vi "DetectorTest_MainV9.vi"() -> ()   [LabVIEW 2012]
uses:
  LabVIEW/Detector IV/SMU Settings.ctl
  <vilib>/Utility/file.llb/Write To Spreadsheet File (string).vi
  <vilib>/Utility/file.llb/Read From Spreadsheet File (string).vi
  <vilib>/Utility/file.llb/Read From Spreadsheet File (DBL).vi
  <vilib>/Analysis/NI_AALBase.lvlib
panel:
  out "RecipeID":string
  in  "Sweep Direction (Keysight)":i32(ring) items=["Up", "Down"]
  in  "Auto Adjust Compliance?":bool
  out "Auto Temp Counter":i32
  out "iteration":i32
  in  "Temp Data":T1={"Ambient Temperature"=20.38176242851337, "Chuck Set Temperature"=35.0} {"Chuck Set Temperature" format="%#.1g"; "Ambient Temperature" format="%#.1g"}
  in  "Wafer Info 3":T2={"Cell Name (Automatic)"="Open_Diode_1000", "Package"="", "Coating"="FOR_AIR", "Comment"="IV test for lot 371", "Flash Setup"="5500_99_03p5", "Hrs under test"=0.0}
  out "TempCounter":i32
  out "WaferCounter":i32
  in  "Profile Z":bool
  in  "Load Wafer":bool
  out "Raw Test Skipped":bool=TRUE
  out "device name w skip":string="Open_Diode_1000(skip)"
  in  "4-wire":bool
  out "Laser Counter":i32
  out "Output Power (mW)":dbl=5.674
  out "Counter":i32
  out "NameList":string[](array[string])
  in  "Wafer Info Flash 2":T3={"Cell Name"="5500_130_05", "Package"="", "Coating"="", "LRC?"=enum."J2", "Comment"="", "Hours Under Test"=0.0}
  in  "Parameters Flash 2":T4 {"Voc" format="%#_4g"; "Isc" format="%#_4g"; "FF" format="%#_4g"; "Imax" format="%#_4g"; "Vmax" format="%#_4g"; "Pmax" format="%#_4g"; "Itest" format="%#_4g"}
  in  "Wafer Info Flash":T3={"Cell Name"="Open_Diode_1000", "Package"="", "Coating"="", "LRC?"=enum."J2", "Comment"="", "Hours Under Test"=0.0}
  in  "Parameters Flash":T4={"Voc"=0.0, "Isc"=0.0, "FF"=0.0, "Vtest"=0.0, "Imax"=0.0, "Vmax"=0.0, "Pmax"=0.0, "Itest"=0.0, "Efficiency"=0.0, "Incident Power"=5.674, "Power Density (W/cm^2)"=0.6679328011361159, "Cell Area (cm²)"=849486.6535, "Number of AM1.5D Suns"=0.0, "Input Current (mA)"=40.0, "Equivalent 1 sun Jsc"=0.0} {"Voc" format="%#_4g"; "Isc" format="%#_4g"; "FF" format="%#_4g"; "Imax" format="%#_4g"; "Vmax" format="%#_4g"; "Pmax" format="%#_4g"; "Itest" format="%#_4g"}
  out "RawData file":path=path "C:/Users/Flash/Desktop/Data/Detector test data/SJC_ENG_371_4-GaAs/A-3719-2-A/Raw Data/A-3719-2-A_Open_Diode_1000_20180913075240.csv"
  out "Fine Cell Clusters":T5(array[cluster])=[{"Cell Name"="Open_Diode_1000", "X-coord"=46800.0, "Y-coord"=22950.0, "Area"=849486.6535, "Grid Shadowing"=0.0, "Xdim"=500.0, "Ydim"=500.0, "Mesa Area"=785398.1634}]
  out "Selected Data":cluster{dbl[], dbl[]}={[nan, nan, nan, nan, nan, nan, nan, nan, nan, nan, nan, nan, nan, nan, nan, nan, nan, nan, nan, nan, nan, nan, nan, nan, nan, nan, nan, nan, nan, nan, nan, nan, nan, nan, nan, nan, nan, nan, nan, nan, nan, nan, nan, nan, nan, nan, nan, nan, nan, nan, nan, nan, nan, nan, nan, nan, nan, nan, nan, nan, nan, nan, nan, nan, nan, nan, nan, nan, nan, nan, nan, nan, nan, nan, nan, nan, nan, nan, nan, nan, nan, nan, nan, nan], [nan, nan, nan, nan, nan, nan, nan, nan, nan, nan, nan, nan, nan, nan, nan, nan, nan, nan, nan, nan, nan, nan, nan, nan, nan, nan, nan, nan, nan, nan, nan, nan, nan, nan, nan, nan, nan, nan, nan, nan, nan, nan, nan, nan, nan, nan, nan, nan, nan, nan, nan, nan, nan, nan, nan, nan, nan, nan, nan, nan, nan, nan, nan, nan, nan, nan, nan, nan, nan, nan, nan, nan, nan, nan, nan, nan, nan, nan, nan, nan, nan, nan, nan, nan]}
  in  "Test Results 2":T6
  in  "Session Info 2":T7={"V set"=-1.0, "I compliance"=0.001, "J set"=0.01, "I set"=0.0, "V compliance"=1.0, "Laser Power (mW)"=0.0, "TestID"=0, "Session Time"=timestamp(0 s since 1904-01-01), "Operator"="Radek"} {"V compliance" format="%#_6f"; "I compliance" format="%#_6e"}
  in  "Die Info 2":T8={"Device Name"="", "ActiveArea_um2"=3848.451, "MesaArea_um2"=3848.451, "x"=0.0, "y"=0.0}
  in  "Wafer Info 2":T9
  in  "Test Results":T6={"I meas"=-1.83245e-12, "V meas"=6.01176, "Time"=timestamp(3619695820.3512325 s since 1904-01-01)}
  in  "Session Info":T7={"V set"=-6.0, "I compliance"=0.001, "J set"=0.01, "I set"=1.9634954079999997e-05, "V compliance"=6.0, "Laser Power (mW)"=0.0, "TestID"=1794, "Session Time"=timestamp(3619695160.866512 s since 1904-01-01), "Operator"="sswifter"} {"V compliance" format="%#_6f"; "I compliance" format="%#_6e"}
  in  "Die Info":T8={"Device Name"="Open_Diode_1000", "ActiveArea_um2"=849486.6535, "MesaArea_um2"=785398.1634, "x"=26800.0, "y"=72950.0}
  in  "Wafer Info":T9={"Wafer Name"="A-3719-2-A", "Scribe"="BJ325-089", "Mask"="PH001", "Lot"="SJC_ENG_371_4-GaAs"}
  in  "Name Array":string[](array[string])=["Wafer name", "Scribe", "Mask", "Lot", "Device name", "Active Area", "Mesa Area", "x", "y", "Imeas", "Vmeas", "Time", "Vset", "Icomp", "Jset", "Iset", "Vcomp", "Laser Power", "TestID", "SessionTime", "Operator", "Selected"]
  in  "TestID file":path=path "C:/Users/Flash/Desktop/LabVIEW/Detector IV/rawtest_log.csv"
  in  "update wafer":bool
  in  "Lot":string="SJC_ENG_370_4-GaAs"
  in  "Laser Current (mA)":dbl
  in  "Device Name":string="Open_Diode_100"
  in  "Scribe":string="BO534-034"
  in  "MesaArea_um2":dbl=15393.804
  out "Status":string="idle"
  out "error out":errorcluster
  in  "error in (no error)":errorcluster
  out "Manaul Plot 1":cluster{"V manual":dbl[], dbl[]}[](array[cluster])=[{"V manual"=[-1.0, -0.964103, -0.928205, -0.892308, -0.85641, -0.820513, -0.784615, -0.748718, -0.712821, -0.676923, -0.641026, -0.605128, -0.569231, -0.533333, -0.497436, -0.461538, -0.425641, -0.389744, -0.353846, -0.317949, -0.282051, -0.246154, -0.210256, -0.174359, -0.138462, -0.102564, -0.0666667, -0.0307693, 0.00512815, 0.0410256, 0.076923, 0.11282, 0.148718, 0.184615, 0.220513, 0.25641, 0.292308, 0.328205, 0.364102, 0.4], [6.85852e-09, 6.65466e-09, 6.5737e-09, 6.49824e-09, 6.4243e-09, 6.35309e-09, 6.27965e-09, 6.20877e-09, 6.13492e-09, 6.06098e-09, 5.98696e-09, 5.91398e-09, 5.83835e-09, 5.76118e-09, 5.68377e-09, 5.60285e-09, 5.52235e-09, 5.437e-09, 5.34957e-09, 5.26073e-09, 5.1657e-09, 5.06509e-09, 4.95213e-09, 4.8214e-09, 4.64754e-09, 4.36963e-09, 3.83525e-09, 2.58988e-09, 1.53713e-10, 2.90069e-08, 4.00867e-08, 2.32852e-07, 3.64301e-07, 1.01107e-06, 2.70206e-06, 6.95726e-06, 1.74528e-05, 3.97407e-05, 8.44992e-05, 0.000100038]}, {"V manual"=[-6.0, nan, nan, nan, nan, nan, nan, nan, nan, nan, nan, nan, nan, nan, nan, nan, nan, nan, nan, nan, nan, nan, nan, nan, nan, nan, nan, nan, nan, nan, nan, nan, nan, nan, nan, nan, nan, nan, nan, nan], [1.709842e-08, nan, nan, nan, nan, nan, nan, nan, nan, nan, nan, nan, nan, nan, nan, nan, nan, nan, nan, nan, nan, nan, nan, nan, nan, nan, nan, nan, nan, nan, nan, nan, nan, nan, nan, nan, nan, nan, nan, nan]}, {"V manual"=[0.126049, nan, nan, nan, nan, nan, nan, nan, nan, nan, nan, nan, nan, nan, nan, nan, nan, nan, nan, nan, nan, nan, nan, nan, nan, nan, nan, nan, nan, nan, nan, nan, nan, nan, nan, nan, nan, nan, nan, nan], [1.9634954080000002e-07, nan, nan, nan, nan, nan, nan, nan, nan, nan, nan, nan, nan, nan, nan, nan, nan, nan, nan, nan, nan, nan, nan, nan, nan, nan, nan, nan, nan, nan, nan, nan, nan, nan, nan, nan, nan, nan, nan, nan]}]
  out "Manual Plot 0":cluster{"V manual":dbl[], "I manual":dbl[]}[](array[cluster])=[{"V manual"=[-1.0, -0.964103, -0.928205, -0.892308, -0.85641, -0.820513, -0.784615, -0.748718, -0.712821, -0.676923, -0.641026, -0.605128, -0.569231, -0.533333, -0.497436, -0.461538, -0.425641, -0.389744, -0.353846, -0.317949, -0.282051, -0.246154, -0.210256, -0.174359, -0.138462, -0.102564, -0.0666667, -0.0307693, 0.00512815, 0.0410256, 0.076923, 0.11282, 0.148718, 0.184615, 0.220513, 0.25641, 0.292308, 0.328205, 0.364102, 0.4], "I manual"=[-6.85852e-09, -6.65466e-09, -6.5737e-09, -6.49824e-09, -6.4243e-09, -6.35309e-09, -6.27965e-09, -6.20877e-09, -6.13492e-09, -6.06098e-09, -5.98696e-09, -5.91398e-09, -5.83835e-09, -5.76118e-09, -5.68377e-09, -5.60285e-09, -5.52235e-09, -5.437e-09, -5.34957e-09, -5.26073e-09, -5.1657e-09, -5.06509e-09, -4.95213e-09, -4.8214e-09, -4.64754e-09, -4.36963e-09, -3.83525e-09, -2.58988e-09, 1.53713e-10, 2.90069e-08, 4.00867e-08, 2.32852e-07, 3.64301e-07, 1.01107e-06, 2.70206e-06, 6.95726e-06, 1.74528e-05, 3.97407e-05, 8.44992e-05, 0.000100038]}, {"V manual"=[-6.0, nan, nan, nan, nan, nan, nan, nan, nan, nan, nan, nan, nan, nan, nan, nan, nan, nan, nan, nan, nan, nan, nan, nan, nan, nan, nan, nan, nan, nan, nan, nan, nan, nan, nan, nan, nan, nan, nan, nan], "I manual"=[-1.709842e-08, nan, nan, nan, nan, nan, nan, nan, nan, nan, nan, nan, nan, nan, nan, nan, nan, nan, nan, nan, nan, nan, nan, nan, nan, nan, nan, nan, nan, nan, nan, nan, nan, nan, nan, nan, nan, nan, nan, nan]}, {"V manual"=[0.126049, nan, nan, nan, nan, nan, nan, nan, nan, nan, nan, nan, nan, nan, nan, nan, nan, nan, nan, nan, nan, nan, nan, nan, nan, nan, nan, nan, nan, nan, nan, nan, nan, nan, nan, nan, nan, nan, nan, nan], "I manual"=[1.9634954080000002e-07, nan, nan, nan, nan, nan, nan, nan, nan, nan, nan, nan, nan, nan, nan, nan, nan, nan, nan, nan, nan, nan, nan, nan, nan, nan, nan, nan, nan, nan, nan, nan, nan, nan, nan, nan, nan, nan, nan, nan]}]
  in  "Reset 1st die":bool
  in  "Sweep Settings":T10={"Channel"=enum."Channel A", "Vstart"=-2.0, "Vend"=0.5, "# of points"=30, "NPLC"=1.0, "I compliance"=0.001, "Delay ms"=500.0}
  in  "Reset xy":bool
  out "current y":i32=1870
  out "current x":i32=23900
  in  "sweep delay ms":dbl=500.0
  in  "I compliance sweep":dbl=0.0001
  in  "points":u16=40
  in  "V end":dbl=0.4
  in  "V start":dbl=-1.0
  in  "Repeat Vf":u32=1
  out "I set":dbl=1.5393804e-06
  in  "V compliance":dbl=6.0 format="%#_6f"
  in  "Vf delay ms":dbl=100.0
  in  "J set A/cm2":dbl=0.01
  in  "Repeat Id":u32=5
  in  "I compliance":dbl=0.001 format="%#_6e"
  in  "Id delay ms":dbl=500.0
  in  "V set":dbl=-6.0
  out "Vmeas Settings":T11={"Channel"=enum."Channel A", "Vset"=1.9634954080000002e-07, "NPLC"=1.0, "I compliance"=6.0, "Repeat time"=1, "Delay ms"=100.0, "4-wire"=FALSE}
  out "Imeas Settings":T11={"Channel"=enum."Channel A", "Vset"=-6.0, "NPLC"=1.0, "I compliance"=0.001, "Repeat time"=5, "Delay ms"=500.0, "4-wire"=FALSE}
  out "Array of Cell Data Clusters":T12(array[cluster])=[{"Cell Name"="Open_Diode_100", "X-coord"=19500.0, "Y-coord"=-4780.0, "Area"=7853.981634, "Grid Shadowing"=0.0, "Ydim"=70.0, "Xdim"=70.0, "Meas Area"=15393.804}, {"Cell Name"="Open_Diode_100", "X-coord"=29500.0, "Y-coord"=-4780.0, "Area"=7853.981634, "Grid Shadowing"=0.0, "Ydim"=70.0, "Xdim"=70.0, "Meas Area"=15393.804}, {"Cell Name"="Open_Diode_100", "X-coord"=3900.0, "Y-coord"=1870.0, "Area"=7853.981634, "Grid Shadowing"=0.0, "Ydim"=70.0, "Xdim"=70.0, "Meas Area"=15393.804}, {"Cell Name"="Open_Diode_100", "X-coord"=13900.0, "Y-coord"=1870.0, "Area"=7853.981634, "Grid Shadowing"=0.0, "Ydim"=70.0, "Xdim"=70.0, "Meas Area"=15393.804}, {"Cell Name"="Open_Diode_100", "X-coord"=23900.0, "Y-coord"=1870.0, "Area"=7853.981634, "Grid Shadowing"=0.0, "Ydim"=70.0, "Xdim"=70.0, "Meas Area"=15393.804}, {"Cell Name"="Open_Diode_100", "X-coord"=9500.0, "Y-coord"=5220.0, "Area"=7853.981634, "Grid Shadowing"=0.0, "Ydim"=70.0, "Xdim"=70.0, "Meas Area"=15393.804}, {"Cell Name"="Open_Diode_100", "X-coord"=19500.0, "Y-coord"=15220.0, "Area"=7853.981634, "Grid Shadowing"=0.0, "Ydim"=70.0, "Xdim"=70.0, "Meas Area"=15393.804}, {"Cell Name"="Open_Diode_100", "X-coord"=39500.0, "Y-coord"=15220.0, "Area"=7853.981634, "Grid Shadowing"=0.0, "Ydim"=70.0, "Xdim"=70.0, "Meas Area"=15393.804}, {"Cell Name"="Open_Diode_100", "X-coord"=-16100.0, "Y-coord"=31870.0, "Area"=7853.981634, "Grid Shadowing"=0.0, "Ydim"=70.0, "Xdim"=70.0, "Meas Area"=15393.804}, {"Cell Name"="Open_Diode_100", "X-coord"=-10500.0, "Y-coord"=55220.0, "Area"=7853.981634, "Grid Shadowing"=0.0, "Ydim"=70.0, "Xdim"=70.0, "Meas Area"=15393.804}]
  in  "stop":bool
  in  "ActiveArea_um2":dbl=7853.981634
  in  "NPLC":dbl=1.0
  in  "Operator":string(combo)="sswifter"
  in  "Mask":string="PH001"
  in  "Wafer Name":string="A-3680-2-A"
  in  "Tab Control":T13(tab)=enum."Manual Test"
  in  "First Wafer Loaded?":bool
  in  "begin lot test":bool
  in  "Desired Wafer Name":string
  in  "Wafer List":i32(listbox)=-1
  in  "Add to wafer list":bool
  in  "Remove from wafer list":bool
  in  "Clear wafer list":bool
  in  "Generate Report":bool
  in  "Only Raw Test":bool
  in  "Clear Laser List":bool
  in  "Remove from Laser List":bool
  in  "Add to Laser":bool
  in  "Desired Current (mA)":dbl=40.0
  in  "Laser List":i32(listbox)=-1
  in  "Start auto":bool
  in  "Clear List":bool
  in  "Refresh Device":bool
  in  "Mask Name":string
  in  "Remove from List":bool
  in  "Add to list":bool
  in  "Available Device Name":string(combo)="Open_Diode_1000"
  in  "Test List":i32(listbox)=-1
  in  "Mask File all":path=path "C:/Users/Flash/Desktop/Mask Files/PH001 Detector GSG/PH001_Detector Aligner mask map file _ full top_open top 10_open top 5 diodes.csv"
  in  "Skip Raw Test?":bool
  in  "Test description":string="IV test for lot 371"
  in  "Clear temp list Auto":bool
  in  "Remove from Temp Auto":bool
  in  "Add to Temp Auto":bool
  in  "Auto Temp Set":dbl=25.0
  in  "Auto Temperature List":i32(listbox)=-1
  in  "Manual_Test":bool
  in  "Manual IV settting":enum32{"Linear plot", "Log plot"}(radio)
  out "Vmeas manual":dbl=0.126049
  out "Imeas manual":dbl=-1.709842e-08
  out "Iarray manual":dbl[](array[numeric])=[-6.85852e-09, -6.65466e-09, -6.5737e-09, -6.49824e-09, -6.4243e-09, -6.35309e-09, -6.27965e-09, -6.20877e-09, -6.13492e-09, -6.06098e-09, -5.98696e-09, -5.91398e-09, -5.83835e-09, -5.76118e-09, -5.68377e-09, -5.60285e-09, -5.52235e-09, -5.437e-09, -5.34957e-09, -5.26073e-09, -5.1657e-09, -5.06509e-09, -4.95213e-09, -4.8214e-09, -4.64754e-09, -4.36963e-09, -3.83525e-09, -2.58988e-09, 1.53713e-10, 2.90069e-08, 4.00867e-08, 2.32852e-07, 3.64301e-07, 1.01107e-06, 2.70206e-06, 6.95726e-06, 1.74528e-05, 3.97407e-05, 8.44992e-05, 0.000100038]
  out "Varray manual":dbl[](array[numeric])=[-1.0, -0.964103, -0.928205, -0.892308, -0.85641, -0.820513, -0.784615, -0.748718, -0.712821, -0.676923, -0.641026, -0.605128, -0.569231, -0.533333, -0.497436, -0.461538, -0.425641, -0.389744, -0.353846, -0.317949, -0.282051, -0.246154, -0.210256, -0.174359, -0.138462, -0.102564, -0.0666667, -0.0307693, 0.00512815, 0.0410256, 0.076923, 0.11282, 0.148718, 0.184615, 0.220513, 0.25641, 0.292308, 0.328205, 0.364102, 0.4]
  out "y target":i32=1870
  out "x target":i32=23900
  in  "Die Number":u16(ring)=4 items=["0", "1", "2", "3", "4", "5", "6", "7", "8", "9", "10", "11", "12", "13", "14", "15", "16", "17", "18", "19", "20", "21", "22", "23", "24", "25", "26", "27", "28", "29", "30", "31", "32", "33", "34", "35", "36", "37", "38", "39", "40", "41", "42", "43", "44", "45", "46", "47", "48", "49", "50", "51", "52", "53", "54", "55", "56", "57", "58", "59", "60", "61", "62", "63", "64", "65", "66", "67", "68", "69", "70", "71", "72", "73", "74", "75", "76", "77", "78", "79", "80", "81", "82", "83", "84", "85"]
  in  "load file":bool
  in  "Move to":bool
  in  "Mask File Manual":path=path "C:/Users/Flash/Desktop/Data/Detector test data/SJC_ENG_370_4-GaAs/A-3680-2-A/Raw Data/PH001_Detector Aligner mask map file _ full top_open top 10_open top 5 diodes_Open_Diode_100_A-3680-2-A_080118_021510.3PM.csv"
  out "Manual IV":cluster{"V manual":dbl[], "I manual":dbl[]}[](graph)=[{"V manual"=[-1.0, -0.964103, -0.928205, -0.892308, -0.85641, -0.820513, -0.784615, -0.748718, -0.712821, -0.676923, -0.641026, -0.605128, -0.569231, -0.533333, -0.497436, -0.461538, -0.425641, -0.389744, -0.353846, -0.317949, -0.282051, -0.246154, -0.210256, -0.174359, -0.138462, -0.102564, -0.0666667, -0.0307693, 0.00512815, 0.0410256, 0.076923, 0.11282, 0.148718, 0.184615, 0.220513, 0.25641, 0.292308, 0.328205, 0.364102, 0.4], "I manual"=[-6.85852e-09, -6.65466e-09, -6.5737e-09, -6.49824e-09, -6.4243e-09, -6.35309e-09, -6.27965e-09, -6.20877e-09, -6.13492e-09, -6.06098e-09, -5.98696e-09, -5.91398e-09, -5.83835e-09, -5.76118e-09, -5.68377e-09, -5.60285e-09, -5.52235e-09, -5.437e-09, -5.34957e-09, -5.26073e-09, -5.1657e-09, -5.06509e-09, -4.95213e-09, -4.8214e-09, -4.64754e-09, -4.36963e-09, -3.83525e-09, -2.58988e-09, 1.53713e-10, 2.90069e-08, 4.00867e-08, 2.32852e-07, 3.64301e-07, 1.01107e-06, 2.70206e-06, 6.95726e-06, 1.74528e-05, 3.97407e-05, 8.44992e-05, 0.000100038]}, {"V manual"=[-6.0, nan, nan, nan, nan, nan, nan, nan, nan, nan, nan, nan, nan, nan, nan, nan, nan, nan, nan, nan, nan, nan, nan, nan, nan, nan, nan, nan, nan, nan, nan, nan, nan, nan, nan, nan, nan, nan, nan, nan], "I manual"=[-1.709842e-08, nan, nan, nan, nan, nan, nan, nan, nan, nan, nan, nan, nan, nan, nan, nan, nan, nan, nan, nan, nan, nan, nan, nan, nan, nan, nan, nan, nan, nan, nan, nan, nan, nan, nan, nan, nan, nan, nan, nan]}, {"V manual"=[0.126049, nan, nan, nan, nan, nan, nan, nan, nan, nan, nan, nan, nan, nan, nan, nan, nan, nan, nan, nan, nan, nan, nan, nan, nan, nan, nan, nan, nan, nan, nan, nan, nan, nan, nan, nan, nan, nan, nan, nan], "I manual"=[1.9634954080000002e-07, nan, nan, nan, nan, nan, nan, nan, nan, nan, nan, nan, nan, nan, nan, nan, nan, nan, nan, nan, nan, nan, nan, nan, nan, nan, nan, nan, nan, nan, nan, nan, nan, nan, nan, nan, nan, nan, nan, nan]}]
  in  "Measure 2 Point?":bool=TRUE
  in  "Manual Test Comments":string="IV test for lot 371"
  in  "Load raw":bool
  in  "Select":bool
  in  "Number Select":u16=10
  in  "Vmax":dbl=5.699999999999999
  in  "Vmin":dbl=0.05
  out "Test FileName":string="A-3719-2-A_Open_Diode_1000_20180913075240.csv"
  out "RawTest ID":u32=1794
  out "Progress":u8(slide)=99 scale=0.0..100.0
  out "Current Device":u32=84
  out "Total Device":u32=84
  out "V meas":dbl[](array[numeric])=[6.01142, 6.01054, 6.01089, 0.000137925, 6.01222, 6.01216, 6.01145, 6.01193, 6.0103, 6.01103, 6.01162, 6.01132, 6.01127, 6.01137, 6.01132, 6.01125, 6.01108, 6.01134, 6.01154, 6.01135, 6.01146, 6.01204, 6.01111, 6.01101, 6.01053, 6.01143, 6.01152, 6.01128, 6.00993, 6.00994, 6.01042, 3.58707, 6.01175, 6.01164, 6.01056, 6.01166, 6.01073, 6.01098, 6.01142, 6.01026, 6.01071, 6.01116, 6.01174, 6.01214, 6.01026, 6.01093, 5.99486, 6.01138, 6.01091, 6.01133, 6.01086, 6.01094, 6.01192, 6.01232, 6.01069, 6.01162, 6.01233, 6.01184, 6.0022, 5.17964, 6.01156, 6.01223, 6.01107, 6.0102, 6.0108, 6.01164, 5.75188, 5.06441, 6.01144, 6.01129, 6.01161, 6.01159, 6.01096, 5.61419, 5.16536, 6.01197, 6.01142, 6.01186, 6.01133, 6.01132, 6.01119, 6.01113, 5.83632, 6.01176]
  out "I meas":dbl[](array[numeric])=[-3.868033999999999e-11, -1.2052780000000002e-09, -6.028065999999999e-11, -0.0009999796, -3.0170019999999996e-11, -4.752688e-11, -4.8625459999999994e-11, -3.7159980000000005e-11, -1.7203160000000002e-07, -2.00883e-08, -7.974548e-11, -3.897576e-11, -3.555112e-11, -2.188194e-08, -5.2771619999999994e-11, -2.9935519999999994e-11, -3.295828e-11, -5.707007999999999e-08, -4.796104e-07, -2.002028e-08, -7.080146e-08, -4.18e-11, -2.108774e-11, -4.09959e-11, -4.424556e-11, -3.3264100000000003e-09, -2.0351338000000002e-10, -6.144901999999999e-09, -4.3002719999999993e-11, -3.898936e-09, -2.0389360000000002e-11, -2.049748e-08, -6.527374000000001e-10, -1.0336196000000001e-10, -2.697004e-11, -3.376518e-08, -6.171924e-11, -2.02069e-10, -1.200538e-09, -2.8179300000000003e-11, -6.537938e-10, -5.153115999999999e-11, -2.8508420000000003e-09, -7.534774e-07, -2.636916e-07, -1.446754e-09, -9.464432000000001e-11, -1.0602588000000001e-10, -4.217728e-11, -7.227086e-08, -3.990094e-11, -2.7389038000000002e-11, -1.90881e-07, -2.2892700000000004e-12, -4.745506e-08, -4.579318e-11, -4.5842860000000003e-11, -5.953868e-11, -3.758154e-11, -4.4363539999999995e-09, -7.143562e-11, -1.397812e-10, -7.11463e-11, -5.56664e-11, -2.6296820000000003e-08, -1.1582659999999999e-07, -2.317642e-11, -5.807276000000001e-11, -2.17813e-12, -5.7970201999999995e-11, -6.71486e-11, -8.667722000000001e-12, 3.2483739999999993e-12, -6.306573999999999e-11, -8.307524e-11, -2.4324079999999998e-12, -2.795726e-12, -2.185576e-12, -2.0225460000000002e-12, -2.122472e-12, -1.6340760000000001e-06, -2.5727129999999997e-06, -3.269066e-11, -1.83245e-12]
  in  "RawData Save Path":path=path "C:/Users/Flash/Desktop/Data/Detector test data"
  in  "StartRaw":bool
  out "Vforward hist":T14(graph)={"X Values"=[0.30074752875, 0.90196673625, 1.5031859437500001, 2.10440515125, 2.70562435875, 3.3068435662500004, 3.90806277375, 4.50928198125, 5.110501188750001, 5.7117203962500005], "Histogram: h(x)"=[1, 0, 0, 0, 0, 1, 0, 0, 3, 79]}
  out "Idark hist":T14(graph)={"X Values"=[-0.0009499806198375813, -0.0008499826595127439, -0.0007499846991879066, -0.0006499867388630691, -0.0005499887785382317, -0.0004499908182133943, -0.0003499928578885569, -0.0002499948975637195, -0.0001499969372388821, -4.99989769140447e-05], "Histogram: h(x)"=[1, 0, 0, 0, 0, 0, 0, 0, 0, 83]}
  in  "Mask File Raw":path=path "C:/Users/Flash/Desktop/Mask Files/PH001 Detector GSG/PH001_Detector Aligner mask map file _ full top_open top 10_open top 5 diodes_Open_Diode_1000.csv"
  out "Spec Plot":cluster{"V meas":dbl[], "I meas":dbl[]}[](graph)=[{"V meas"=[6.01142, 6.01054, 6.01089, 0.000137925, 6.01222, 6.01216, 6.01145, 6.01193, 6.0103, 6.01103, 6.01162, 6.01132, 6.01127, 6.01137, 6.01132, 6.01125, 6.01108, 6.01134, 6.01154, 6.01135, 6.01146, 6.01204, 6.01111, 6.01101, 6.01053, 6.01143, 6.01152, 6.01128, 6.00993, 6.00994, 6.01042, 3.58707, 6.01175, 6.01164, 6.01056, 6.01166, 6.01073, 6.01098, 6.01142, 6.01026, 6.01071, 6.01116, 6.01174, 6.01214, 6.01026, 6.01093, 5.99486, 6.01138, 6.01091, 6.01133, 6.01086, 6.01094, 6.01192, 6.01232, 6.01069, 6.01162, 6.01233, 6.01184, 6.0022, 5.17964, 6.01156, 6.01223, 6.01107, 6.0102, 6.0108, 6.01164, 5.75188, 5.06441, 6.01144, 6.01129, 6.01161, 6.01159, 6.01096, 5.61419, 5.16536, 6.01197, 6.01142, 6.01186, 6.01133, 6.01132, 6.01119, 6.01113, 5.83632, 6.01176], "I meas"=[-3.868033999999999e-11, -1.2052780000000002e-09, -6.028065999999999e-11, -0.0009999796, -3.0170019999999996e-11, -4.752688e-11, -4.8625459999999994e-11, -3.7159980000000005e-11, -1.7203160000000002e-07, -2.00883e-08, -7.974548e-11, -3.897576e-11, -3.555112e-11, -2.188194e-08, -5.2771619999999994e-11, -2.9935519999999994e-11, -3.295828e-11, -5.707007999999999e-08, -4.796104e-07, -2.002028e-08, -7.080146e-08, -4.18e-11, -2.108774e-11, -4.09959e-11, -4.424556e-11, -3.3264100000000003e-09, -2.0351338000000002e-10, -6.144901999999999e-09, -4.3002719999999993e-11, -3.898936e-09, -2.0389360000000002e-11, -2.049748e-08, -6.527374000000001e-10, -1.0336196000000001e-10, -2.697004e-11, -3.376518e-08, -6.171924e-11, -2.02069e-10, -1.200538e-09, -2.8179300000000003e-11, -6.537938e-10, -5.153115999999999e-11, -2.8508420000000003e-09, -7.534774e-07, -2.636916e-07, -1.446754e-09, -9.464432000000001e-11, -1.0602588000000001e-10, -4.217728e-11, -7.227086e-08, -3.990094e-11, -2.7389038000000002e-11, -1.90881e-07, -2.2892700000000004e-12, -4.745506e-08, -4.579318e-11, -4.5842860000000003e-11, -5.953868e-11, -3.758154e-11, -4.4363539999999995e-09, -7.143562e-11, -1.397812e-10, -7.11463e-11, -5.56664e-11, -2.6296820000000003e-08, -1.1582659999999999e-07, -2.317642e-11, -5.807276000000001e-11, -2.17813e-12, -5.7970201999999995e-11, -6.71486e-11, -8.667722000000001e-12, 3.2483739999999993e-12, -6.306573999999999e-11, -8.307524e-11, -2.4324079999999998e-12, -2.795726e-12, -2.185576e-12, -2.0225460000000002e-12, -2.122472e-12, -1.6340760000000001e-06, -2.5727129999999997e-06, -3.269066e-11, -1.83245e-12]}, {"V meas"=[3.58707, nan, nan, nan, nan, nan, nan, nan, nan, nan, nan, nan, nan, nan, nan, nan, nan, nan, nan, nan, nan, nan, nan, nan, nan, nan, nan, nan, nan, nan, nan, nan, nan, nan, nan, nan, nan, nan, nan, nan, nan, nan, nan, nan, nan, nan, nan, nan, nan, nan, nan, nan, nan, nan, nan, nan, nan, nan, nan, nan, nan, nan, nan, nan, nan, nan, nan, nan, nan, nan, nan, nan, nan, nan, nan, nan, nan, nan, nan, nan, nan, nan, nan, nan], "I meas"=[-2.049748e-08, nan, nan, nan, nan, nan, nan, nan, nan, nan, nan, nan, nan, nan, nan, nan, nan, nan, nan, nan, nan, nan, nan, nan, nan, nan, nan, nan, nan, nan, nan, nan, nan, nan, nan, nan, nan, nan, nan, nan, nan, nan, nan, nan, nan, nan, nan, nan, nan, nan, nan, nan, nan, nan, nan, nan, nan, nan, nan, nan, nan, nan, nan, nan, nan, nan, nan, nan, nan, nan, nan, nan, nan, nan, nan, nan, nan, nan, nan, nan, nan, nan, nan, nan]}]
  in  "Explore Data":bool
  out "no file":bool
  in  "Comments":string="IV test for lot 371"
  in  "FineTest save path":path=path "C:/Users/Flash/Desktop/Data/Detector test data"
  out "I fine":dbl[](array[numeric])=[-2.70504e-08, -2.32087e-08, -1.94015e-08, -1.62001e-08, -1.3396e-08, -1.06144e-08, -8.14274e-09, -5.83125e-09, -3.66964e-09, -2.05099e-09, -1.05505e-09, -6.56038e-10, -4.43558e-10, -3.24538e-10, -2.3071e-10, -1.84326e-10, -1.50747e-10, -1.31042e-10, -1.1589e-10, -1.0217e-10, -9.29752e-11, -8.22993e-11, -7.74358e-11, -6.84813e-11, -6.19634e-11, -5.51294e-11, -4.86827e-11, -4.15262e-11, -3.40749e-11, -2.82174e-11, -2.14966e-11, -1.33787e-11, -7.37435e-12, -5.50663e-12, 4.69868e-12, 1.38179e-11, 4.52471e-11, 2.99241e-10, 1.96981e-09, 2.81104e-08]
  out "V fine":dbl[](array[numeric])=[-6.0, -5.82051, -5.64103, -5.46154, -5.28205, -5.10256, -4.92308, -4.74359, -4.5641, -4.38461, -4.20513, -4.02564, -3.84615, -3.66667, -3.48718, -3.30769, -3.1282, -2.94872, -2.76923, -2.58974, -2.41026, -2.23077, -2.05128, -1.87179, -1.69231, -1.51282, -1.33333, -1.15384, -0.974358, -0.79487, -0.615383, -0.435896, -0.256409, -0.0769218, 0.102565, 0.282053, 0.46154, 0.641027, 0.820514, 1.0]
  out "Current Device":u32=1
  out "Total Device":u32=1
  out "IV fine log":cluster{dbl[], dbl[]}[](graph)=[{[-6.0, -5.82051, -5.64103, -5.46154, -5.28205, -5.10256, -4.92308, -4.74359, -4.5641, -4.38461, -4.20513, -4.02564, -3.84615, -3.66667, -3.48718, -3.30769, -3.1282, -2.94872, -2.76923, -2.58974, -2.41026, -2.23077, -2.05128, -1.87179, -1.69231, -1.51282, -1.33333, -1.15384, -0.974358, -0.79487, -0.615383, -0.435896, -0.256409, -0.0769218, 0.102565, 0.282053, 0.46154, 0.641027, 0.820514, 1.0], [2.70504e-08, 2.32087e-08, 1.94015e-08, 1.62001e-08, 1.3396e-08, 1.06144e-08, 8.14274e-09, 5.83125e-09, 3.66964e-09, 2.05099e-09, 1.05505e-09, 6.56038e-10, 4.43558e-10, 3.24538e-10, 2.3071e-10, 1.84326e-10, 1.50747e-10, 1.31042e-10, 1.1589e-10, 1.0217e-10, 9.29752e-11, 8.22993e-11, 7.74358e-11, 6.84813e-11, 6.19634e-11, 5.51294e-11, 4.86827e-11, 4.15262e-11, 3.40749e-11, 2.82174e-11, 2.14966e-11, 1.33787e-11, 7.37435e-12, 5.50663e-12, 4.69868e-12, 1.38179e-11, 4.52471e-11, 2.99241e-10, 1.96981e-09, 2.81104e-08]}]
  out "Progress 2":u8(slide)=100 scale=0.0..100.0
  in  "StartFine":bool
  out "IV fine linear":cluster{dbl[], dbl[]}[](graph)=[{[-6.0, -5.82051, -5.64103, -5.46154, -5.28205, -5.10256, -4.92308, -4.74359, -4.5641, -4.38461, -4.20513, -4.02564, -3.84615, -3.66667, -3.48718, -3.30769, -3.1282, -2.94872, -2.76923, -2.58974, -2.41026, -2.23077, -2.05128, -1.87179, -1.69231, -1.51282, -1.33333, -1.15384, -0.974358, -0.79487, -0.615383, -0.435896, -0.256409, -0.0769218, 0.102565, 0.282053, 0.46154, 0.641027, 0.820514, 1.0], [-2.70504e-08, -2.32087e-08, -1.94015e-08, -1.62001e-08, -1.3396e-08, -1.06144e-08, -8.14274e-09, -5.83125e-09, -3.66964e-09, -2.05099e-09, -1.05505e-09, -6.56038e-10, -4.43558e-10, -3.24538e-10, -2.3071e-10, -1.84326e-10, -1.50747e-10, -1.31042e-10, -1.1589e-10, -1.0217e-10, -9.29752e-11, -8.22993e-11, -7.74358e-11, -6.84813e-11, -6.19634e-11, -5.51294e-11, -4.86827e-11, -4.15262e-11, -3.40749e-11, -2.82174e-11, -2.14966e-11, -1.33787e-11, -7.37435e-12, -5.50663e-12, 4.69868e-12, 1.38179e-11, 4.52471e-11, 2.99241e-10, 1.96981e-09, 2.81104e-08]}]
  in  "Mask File Fine":path=path "C:/Users/Flash/Desktop/Data/Detector test data/SJC_ENG_371_4-GaAs/A-3719-2-A/Raw Data/PH001_Detector Aligner mask map file _ full top_open top 10_open top 5 diodes_Open_Diode_1000_A-3719-2-A_091318_080341.5AM.csv"
  out "Y":dbl
  out "X":dbl
  in  "move prober 2":bool
  in  "load file for temp series":bool
  in  "Mask File Temperature":path=path "C:/Users/Flash/Desktop/Data/Detector test data/PH001 Detector Aligner mask map file _ full top_open top 10_open top 5 diodes_Open_Diode_5_300_A-3605-1-A_052518_113739.0AM.csv"
  out "IV temp linear":cluster{dbl[], dbl[]}[](graph)
  in  "Start temp":bool
  out "IV temp log":cluster{dbl[], dbl[]}[](graph)
  out "V fine temp":dbl[](array[numeric])=[-1.5, -1.45128, -1.40256, -1.35385, -1.30513, -1.25641, -1.20769, -1.15897, -1.11026, -1.06154, -1.01282, -0.964102, -0.915384, -0.866666, -0.817948, -0.76923, -0.720512, -0.671794, -0.623076, -0.574358, -0.52564, -0.476923, -0.428205, -0.379487, -0.330769, -0.282051, -0.233333, -0.184615, -0.135897, -0.087179, -0.038461, 0.0102569, 0.0589749, 0.107693, 0.156411, 0.205129, 0.253847, 0.302565, 0.351283, 0.400001]
  out "I fine temp":dbl[](array[numeric])=[-1.28772e-07, -1.20805e-07, -1.15592e-07, -1.10987e-07, -1.06412e-07, -1.02022e-07, -4.62038e-08, -9.34188e-08, -8.97462e-08, -8.60003e-08, -8.23237e-08, -7.87101e-08, -7.52945e-08, -7.18306e-08, -6.85145e-08, -6.5287e-08, -6.2088e-08, -5.90038e-08, -5.59938e-08, -5.29941e-08, -5.00661e-08, -4.71812e-08, -4.43421e-08, -4.15389e-08, -3.87298e-08, -3.5945e-08, -3.31511e-08, -3.027e-08, -2.71168e-08, -2.30654e-08, -1.54139e-08, 7.82768e-09, 2.30625e-07, 5.07951e-07, 2.21662e-06, 9.15235e-06, 3.37902e-05, 9.47719e-05, 0.000202989, 0.000357986]
  in  "Temperature Series save path":path=path "C:/Users/Flash/Desktop/Data/Detector test data"
  in  "Comments Temp":string
  in  "Single Device Temperature List":i32(listbox)=-1
  in  "Desired Temperature":dbl=25.0
  in  "Add to Temp":bool
  in  "Remove from Temp":bool
  in  "Clear temp list":bool
  in  "Desired Device":u16(ring)=50 items=["0", "1", "2", "3", "4", "5", "6", "7", "8", "9"]
  in  "Channel Keysight":dbl
  in  "Keysight SMU":refnum<visa-resource-name>="GPIB0::23::INSTR"
  in  "update temp":bool
  out "Current Temp":string="0\r"
  in  "Temp Setpoint":string="25"
  in  "Temptronics VISA":refnum<visa-resource-name>="GPIB0::9::INSTR"
  in  "Prober GPIB":string="0:1"
  in  "Keithley SMU":refnum<visa-resource-name>="GPIB0::26::INSTR"
  in  "Channel":enum32{"Channel A", "Channel B"}(ring)
  out "Calibration":cluster{"Y":dbl[], "Y":dbl[]}[](graph)=[{"Y"=[0.1, 0.2, 0.3, 0.4, 0.5, 0.6, 0.7, 0.8, 0.9, 1.0, 1.1, 1.2, 1.3, 1.4, 1.5, 1.6, 1.7, 1.8, 1.9, 2.0, 2.1, 2.2, 2.3, 2.4, 2.5, 2.6, 2.7, 2.8, 2.9, 3.0, 3.1, 3.2, 3.3, 3.4, 3.5, 3.6, 3.7, 3.8, 3.9, 4.0, 4.1, 4.2, 4.3, 4.4, 4.5, 4.6, 4.7, 4.8, 4.9, 5.0, 5.1, 5.2, 5.3, 5.4, 5.5, 5.6, 5.7, 5.8, 5.9, 6.0, 6.1, 6.2, 6.3, 6.4, 6.5, 6.6, 6.7, 6.8, 6.9, 7.0, 7.1, 7.2, 7.3, 7.4, 7.5, 7.6, 7.7, 7.8, 7.9, 8.0, 8.1, 8.2, 8.3, 8.4, 8.5, 8.6, 8.7, 8.8, 8.9, 9.0, 9.1, 9.2, 9.3, 9.4, 9.5, 9.6, 9.7, 9.8, 9.9, 10.0, 10.1, 10.2, 10.3, 10.4, 10.5, 10.6, 10.7, 10.8, 10.9, 11.0, 11.1, 11.2, 11.3, 11.4, 11.5, 11.6, 11.7, 11.8, 11.9, 12.0, 12.1, 12.2, 12.3, 12.4, 12.5, 12.6, 12.7, 12.8, 12.9, 13.0, 13.1, 13.2, 13.3, 13.4, 13.5, 13.6, 13.7, 13.8, 13.9, 14.0, 14.1, 14.2, 14.3, 14.4, 14.5, 14.6, 14.7, 14.8, 14.9, 15.0, 15.1, 15.2, 15.3, 15.4, 15.5, 15.6, 15.7, 15.8, 15.9, 16.0, 16.1, 16.2, 16.3, 16.4, 16.5, 16.6, 16.7, 16.8, 16.9, 17.0, 17.1, 17.2, 17.3, 17.4, 17.5, 17.6, 17.7, 17.8, 17.9, 18.0, 18.1, 18.2, 18.3, 18.4, 18.5, 18.6, 18.7, 18.8, 18.9, 19.0, 19.1, 19.2, 19.3, 19.4, 19.5, 19.6, 19.7, 19.8, 19.9, 20.0, 20.1, 20.2, 20.3, 20.4, 20.5, 20.6, 20.7, 20.8, 20.9, 21.0, 21.1, 21.2, 21.3, 21.4, 21.5, 21.6, 21.7, 21.8, 21.9, 22.0, 22.1, 22.2, 22.3, 22.4, 22.5, 22.6, 22.7, 22.8, 22.9, 23.0, 23.1, 23.2, 23.3, 23.4, 23.5, 23.6, 23.7, 23.8, 23.9, 24.0, 24.1, 24.2, 24.3, 24.4, 24.5, 24.6, 24.7, 24.8, 24.9, 25.0, 25.1, 25.2, 25.3, 25.4, 25.5, 25.6, 25.7, 25.8, 25.9, 26.0, 26.1, 26.2, 26.3, 26.4, 26.5, 26.6, 26.7, 26.8, 26.9, 27.0, 27.1, 27.2, 27.3, 27.4, 27.5, 27.6, 27.7, 27.8, 27.9, 28.0, 28.1, 28.2, 28.3, 28.4, 28.5, 28.6, 28.7, 28.8, 28.9, 29.0, 29.1, 29.2, 29.3, 29.4, 29.5, 29.6, 29.7, 29.8, 29.9, 30.0, 30.1, 30.2, 30.3, 30.4, 30.5, 30.6, 30.7, 30.8, 30.9, 31.0, 31.1, 31.2, 31.3, 31.4, 31.5, 31.6, 31.7, 31.8, 31.9, 32.0, 32.1, 32.2, 32.3, 32.4, 32.5, 32.6, 32.7, 32.8, 32.9, 33.0, 33.1, 33.2, 33.3, 33.4, 33.5, 33.6, 33.7, 33.8, 33.9, 34.0, 34.1, 34.2, 34.3, 34.4, 34.5, 34.6, 34.7, 34.8, 34.9, 35.0, 35.1, 35.2, 35.3, 35.4, 35.5, 35.6, 35.7, 35.8, 35.9, 36.0, 36.1, 36.2, 36.3, 36.4, 36.5, 36.6, 36.7, 36.8, 36.9, 37.0, 37.1, 37.2, 37.3, 37.4, 37.5, 37.6, 37.7, 37.8, 37.9, 38.0, 38.1, 38.2, 38.3, 38.4, 38.5, 38.6, 38.7, 38.8, 38.9, 39.0, 39.1, 39.2, 39.3, 39.4, 39.5, 39.6, 39.7, 39.8, 39.9, 40.0], "Y"=[0.0, 0.0, 0.0, 0.0, 0.0, 0.0, 0.0, 0.0, 0.0, 0.0, 0.0, 0.0, 0.0, 0.0, 0.0, 0.0, 0.0, 0.0, 0.001, 0.001, 0.001, 0.001, 0.001, 0.001, 0.001, 0.001, 0.001, 0.001, 0.001, 0.001, 0.001, 0.001, 0.001, 0.001, 0.001, 0.002, 0.002, 0.002, 0.002, 0.002, 0.002, 0.002, 0.002, 0.002, 0.002, 0.003, 0.003, 0.003, 0.003, 0.003, 0.003, 0.004, 0.004, 0.004, 0.004, 0.004, 0.005, 0.005, 0.005, 0.005, 0.006, 0.006, 0.006, 0.007, 0.007, 0.007, 0.008, 0.008, 0.008, 0.009, 0.009, 0.01, 0.01, 0.01, 0.011, 0.012, 0.012, 0.013, 0.013, 0.014, 0.015, 0.016, 0.018, 0.023, 0.036, 0.055, 0.071, 0.088, 0.105, 0.121, 0.143, 0.159, 0.176, 0.194, 0.209, 0.232, 0.249, 0.276, 0.28, 0.301, 0.317, 0.335, 0.354, 0.37, 0.388, 0.407, 0.423, 0.438, 0.455, 0.481, 0.493, 0.522, 0.535, 0.558, 0.57, 0.579, 0.608, 0.62, 0.648, 0.662, 0.671, 0.693, 0.703, 0.738, 0.756, 0.773, 0.782, 0.813, 0.817, 0.846, 0.841, 0.865, 0.892, 0.904, 0.933, 0.952, 0.972, 0.989, 1.01, 1.002, 1.032, 1.049, 1.067, 1.088, 1.1, 1.132, 1.144, 1.168, 1.158, 1.184, 1.223, 1.242, 1.265, 1.263, 1.305, 1.322, 1.304, 1.319, 1.346, 1.374, 1.375, 1.393, 1.448, 1.465, 1.465, 1.465, 1.523, 1.539, 1.534, 1.533, 1.59, 1.598, 1.631, 1.612, 1.62, 1.669, 1.69, 1.675, 1.743, 1.708, 1.765, 1.792, 1.818, 1.802, 1.849, 1.86, 1.885, 1.878, 1.925, 1.898, 1.933, 1.954, 2.001, 1.968, 1.999, 2.011, 2.068, 2.088, 2.093, 2.076, 2.114, 2.142, 2.124, 2.194, 2.202, 2.222, 2.246, 2.238, 2.229, 2.251, 2.265, 2.274, 2.308, 2.377, 2.382, 2.344, 2.43, 2.443, 2.404, 2.426, 2.457, 2.524, 2.511, 2.511, 2.504, 2.582, 2.604, 2.555, 2.583, 2.625, 3.197, 2.696, 2.645, 2.677, 2.73, 2.716, 2.711, 2.739, 2.796, 2.848, 2.864, 2.809, 2.898, 2.837, 2.86, 2.9, 2.964, 2.937, 2.994, 2.997, 2.966, 2.981, 2.995, 3.086, 3.108, 3.131, 3.063, 3.166, 3.164, 3.177, 3.156, 3.188, 3.248, 3.2, 3.239, 3.236, 3.307, 3.278, 3.333, 3.298, 3.403, 3.412, 3.394, 3.397, 3.469, 3.414, 3.479, 3.518, 3.464, 3.525, 3.483, 3.499, 3.554, 3.529, 3.653, 3.658, 3.64, 3.606, 3.711, 3.667, 3.648, 3.756, 3.752, 3.755, 3.742, 3.808, 3.775, 3.812, 3.83, 3.884, 3.868, 3.959, 3.966, 3.901, 3.934, 4.01, 4.032, 4.011, 4.045, 4.004, 4.096, 4.131, 4.163, 4.17, 4.084, 4.219, 4.195, 4.184, 4.2, 4.165, 4.246, 4.204, 4.233, 4.256, 4.344, 4.377, 4.299, 4.33, 4.326, 4.344, 4.485, 4.513, 4.507, 4.427, 4.473, 4.582, 4.461, 4.559, 4.63, 4.638, 4.569, 4.583, 4.569, 4.63, 4.596, 4.765, 4.758, 4.682, 4.821, 4.692, 4.757, 4.868, 4.783, 4.891, 4.808, 4.879, 4.88, 4.873, 4.99, 4.965, 5.016, 4.934, 5.058, 5.076, 5.076, 5.058, 5.066, 5.085, 5.138, 5.185, 5.185, 5.228, 5.218, 5.266, 5.176, 5.184, 5.266, 5.196, 5.333, 5.358, 5.246, 5.3, 5.314, 5.297, 5.32, 5.486, 5.353, 5.483, 5.442, 5.408, 5.557, 5.436, 5.581, 5.619, 5.616, 5.564, 5.557, 5.669, 5.7, 5.674]}]
  out "Laser Error":errorcluster caption="error out" {"code" format="%.0x"}
  in  "Load Calibration File":path=path "C:/Users/Flash/Desktop/Laser Calibration Files/Calib7_23_18.csv"
  in  "TL4000 In":refnum<visa-resource-name>="USB0::0x1313::0x804F::M00445403::INSTR" caption="resource name"
  in  "Enable Laser":bool=TRUE
  out "Raw Test Filename":path=path "C:/Users/Flash/Desktop/Data/Detector test data/SJC_ENG_371_4-GaAs/A-3719-2-A/Raw Data/A-3719-2-A_Open_Diode_1000_20180913075240.csv"
  out "new raw data save path":path=path "C:/Users/Flash/Desktop/Data/Detector test data/SJC_ENG_371_4-GaAs/A-3719-2-A/Raw Data"
  out "Error Out":errorcluster
  in  "Wait after load":u32
  in  "Keysight":bool
  out "Test Type":string="Auto Test"
  in  "Update viewer":bool
  in  "Logview":i32(listbox)
  in  "Add Comments":string
  in  "Save Comment":bool
  out "Last Measurement":T15={"result string"="9_13_2018", "time string"="11:39 AM", "Wafer Name"="A-3719-2-A", "Operator"="sswifter", "Test description"="IV test for lot 371", "Test Type"="Auto Test"}
  # "0 is for dark IV!"
  # "Sweep Settings"
  # "Forward Voltage"
  # "Dark/Light Current"
  # "Check settings before click start!"
  # "Make sure current x and y are same as prober before click Start!"
  # "TEC Control"
  # "TL4000 Settings"
  # "Keithley"
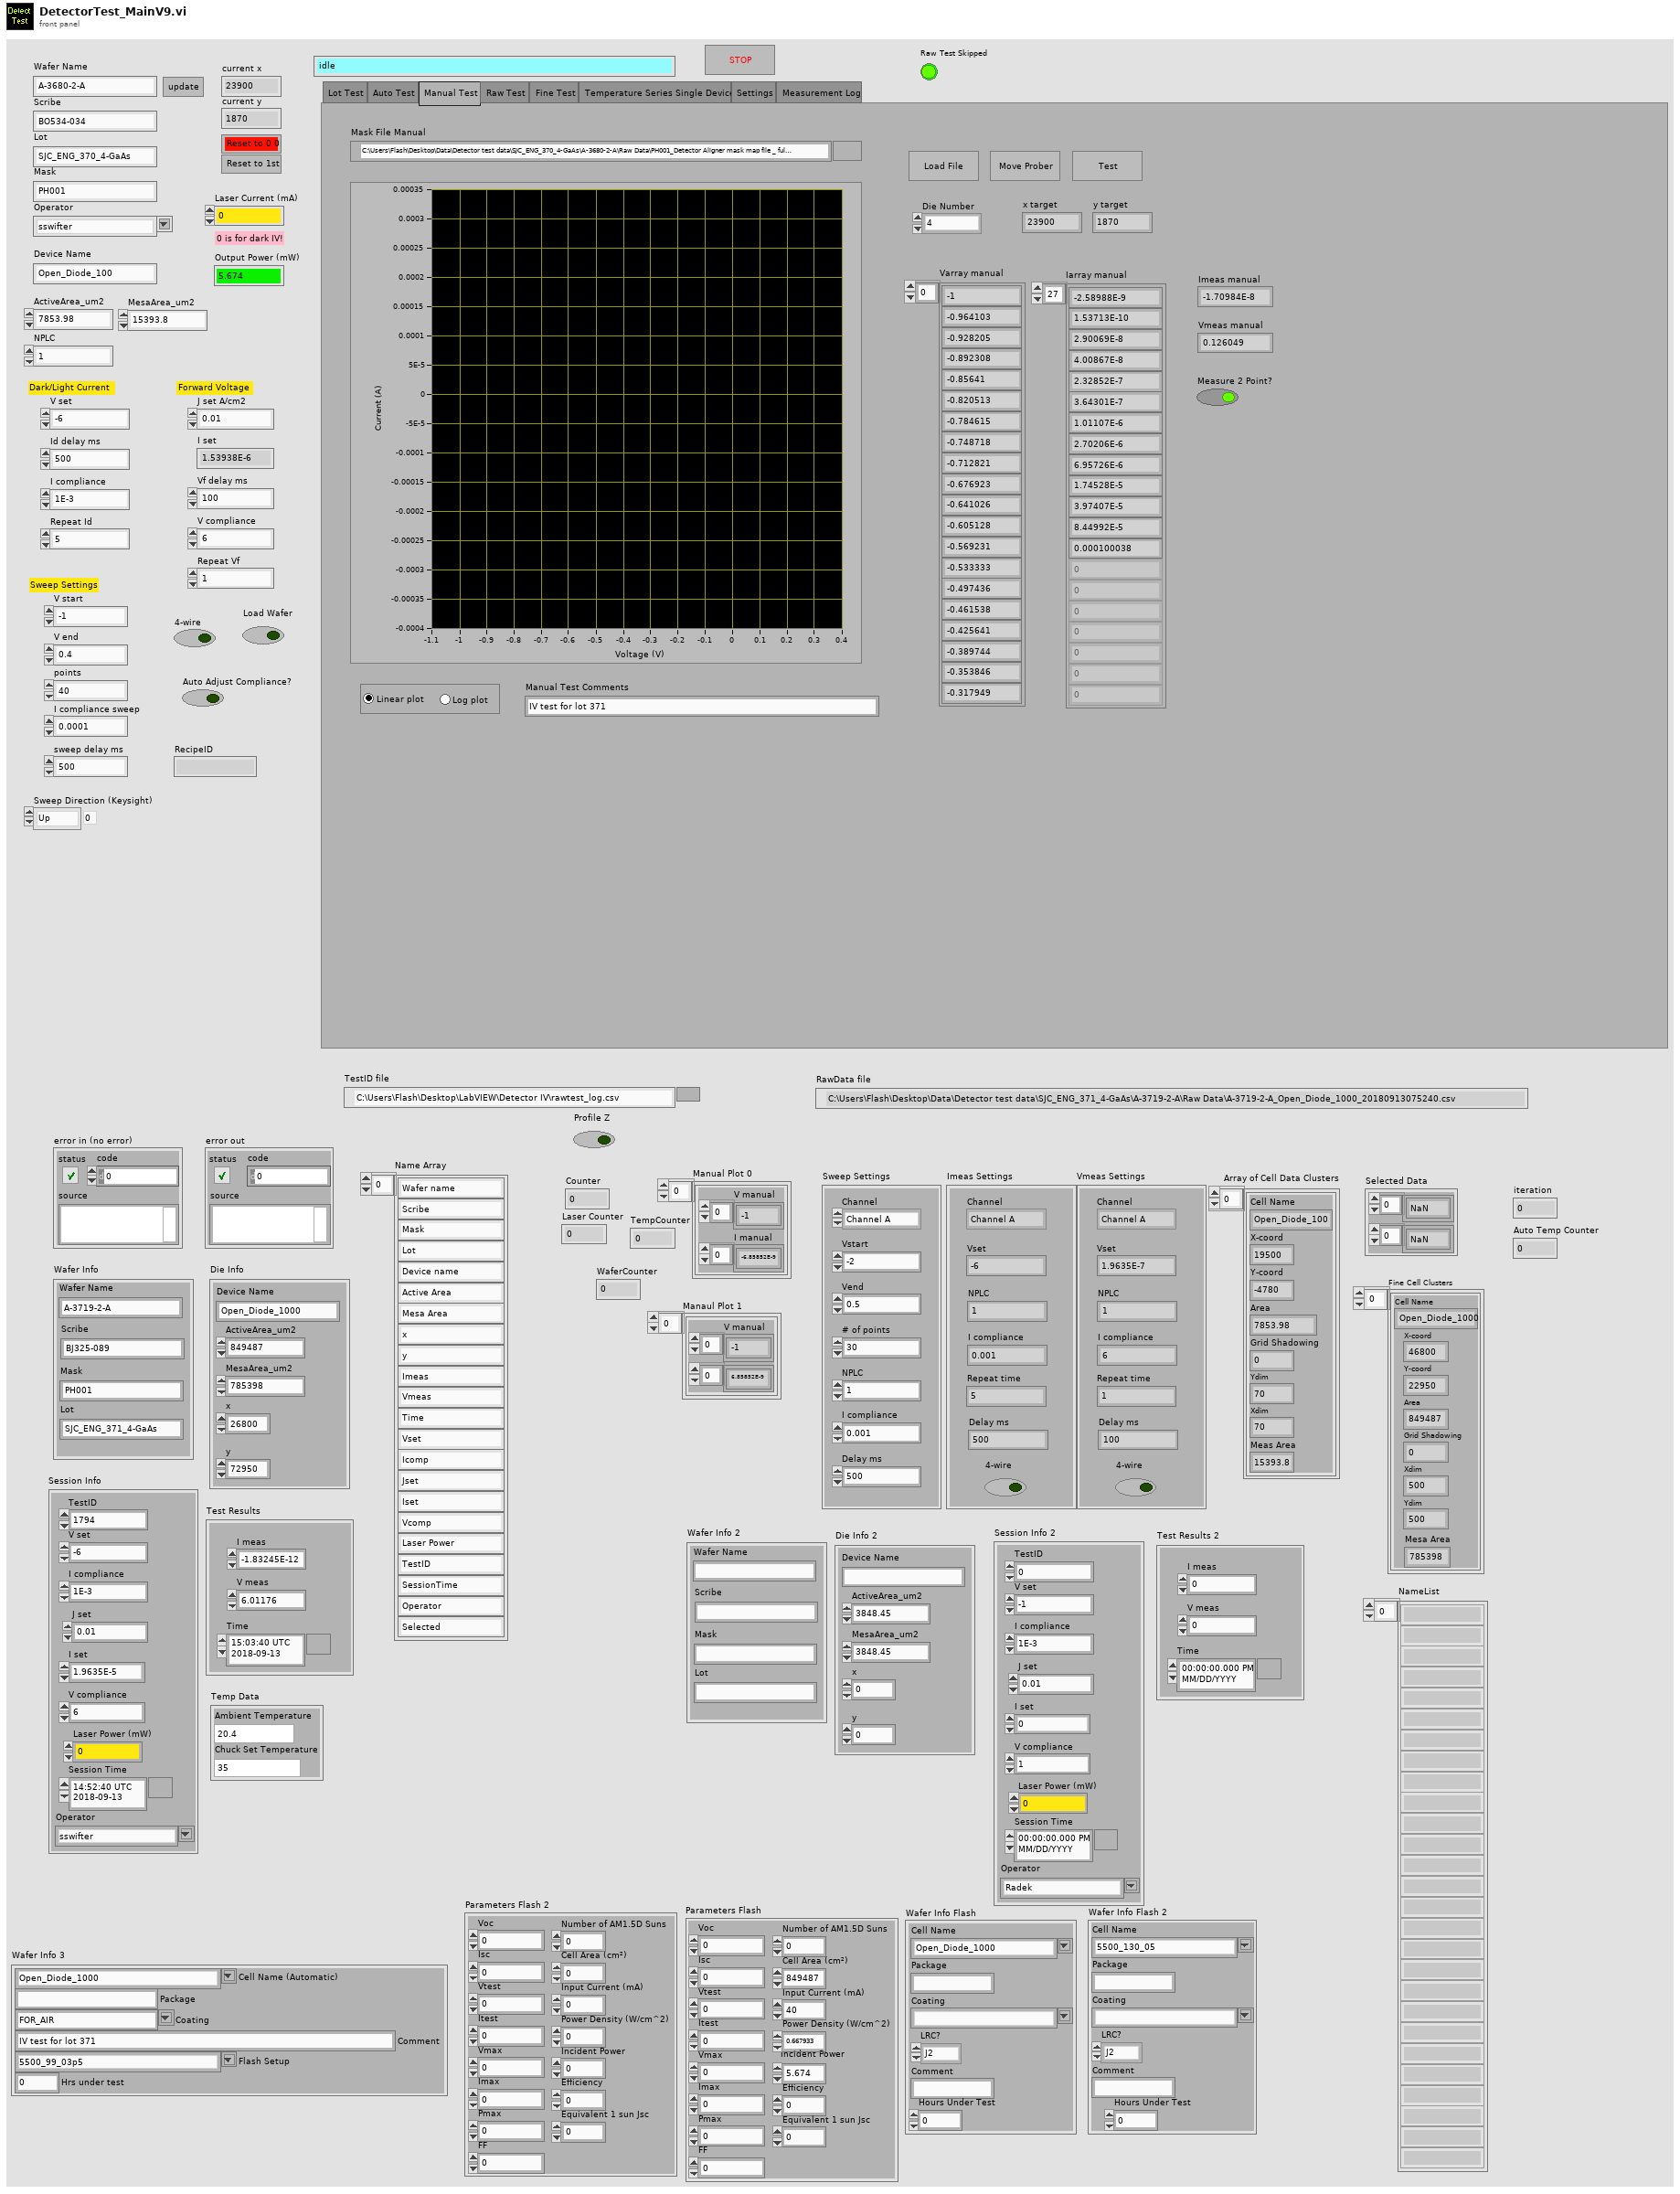
[diagram p1: front panel]
types:
  T1 = cluster{"Ambient Temperature":dbl, "Chuck Set Temperature":dbl}
  T2 = cluster{"Cell Name (Automatic)":string, "Package":string, "Coating":string, "Comment":string, "Flash Setup":string, "Hrs under test":dbl}
  T3 = cluster{"Cell Name":string, "Package":string, "Coating":string, "LRC?":enum16{"J1", "J2", "LRC"}, "Comment":string, "Hours Under Test":dbl}
  T4 = cluster{"Voc":dbl, "Isc":dbl, "FF":dbl, "Vtest":dbl, "Imax":dbl, "Vmax":dbl, "Pmax":dbl, "Itest":dbl, "Efficiency":dbl, "Incident Power":dbl, "Power Density (W/cm^2)":dbl, "Cell Area (cm²)":dbl, "Number of AM1.5D Suns":dbl, "Input Current (mA)":dbl, "Equivalent 1 sun Jsc":dbl}
  T5 = cluster{"Cell Name":string, "X-coord":dbl, "Y-coord":dbl, "Area":dbl, "Grid Shadowing":dbl, "Xdim":dbl, "Ydim":dbl, "Mesa Area":dbl}[]
  T6 = cluster{"I meas":dbl, "V meas":dbl, "Time":timestamp}
  T7 = cluster{"V set":dbl, "I compliance":dbl, "J set":dbl, "I set":dbl, "V compliance":dbl, "Laser Power (mW)":dbl, "TestID":u32, "Session Time":timestamp, "Operator":string}
  T8 = cluster{"Device Name":string, "ActiveArea_um2":dbl, "MesaArea_um2":dbl, "x":dbl, "y":dbl}
  T9 = cluster{"Wafer Name":string, "Scribe":string, "Mask":string, "Lot":string}
  T10 = cluster{"Channel":enum32{"Channel A", "Channel B"}, "Vstart":dbl, "Vend":dbl, "# of points":u16, "NPLC":dbl, "I compliance":dbl, "Delay ms":dbl}
  T11 = typedef "SMU Settings.ctl" = cluster{"Channel":enum32{"Channel A", "Channel B"}, "Vset":dbl, "NPLC":dbl, "I compliance":dbl, "Repeat time":u16, "Delay ms":dbl, "4-wire":bool}
  T12 = cluster{"Cell Name":string, "X-coord":dbl, "Y-coord":dbl, "Area":dbl, "Grid Shadowing":dbl, "Ydim":dbl, "Xdim":dbl, "Meas Area":dbl}[]
  T13 = enum32{"Lot Test", "Auto Test", "Manual Test", "Raw Test", "Fine Test", "Temperature Series Single Device", "Settings", "Measurement Log"}
  T14 = cluster{"X Values":dbl[], "Histogram: h(x)":i32[]}
  T15 = cluster{"result string":string, "time string":string, "Wafer Name":string, "Operator":string, "Test description":string, "Test Type":string}
  T16 = enum32{"Lot Test", "Auto Test", "Manual Test", "Raw Test", "Fine Test", "Temperature Series Single Device", "Settings"}
  T17 = cluster{"Cell Name":string, "X-coord":dbl, "Y-coord":dbl, "Area":dbl, "Grid Shadowing":dbl, "Ydim":dbl, "Xdim":dbl, "Meas Area":dbl}
  T18 = cluster{"Varray manual":dbl[], "Iarray manual":dbl[]}[]
  T19 = cluster{"WaferName":string, "Scribe":string, "Structure":string, "Lot":string, "Mask":string}
  T20 = cluster{"V set":dbl, "I compliance":dbl, "J set":dbl, "I set":dbl, "V compliance":dbl, "Laser Power (mW)":dbl, "TestID":u32, "Operator":string}
  T21 = cluster{"Device Name":string, "ActiveArea_um2":dbl, "MesaArea_um2":dbl}
  T22 = cluster{"Cell Name":string, "X-coord":dbl, "Y-coord":dbl, "Area":dbl, "Grid Shadowing":dbl, "Xdim":dbl, "Ydim":dbl, "Mesa Area":dbl}
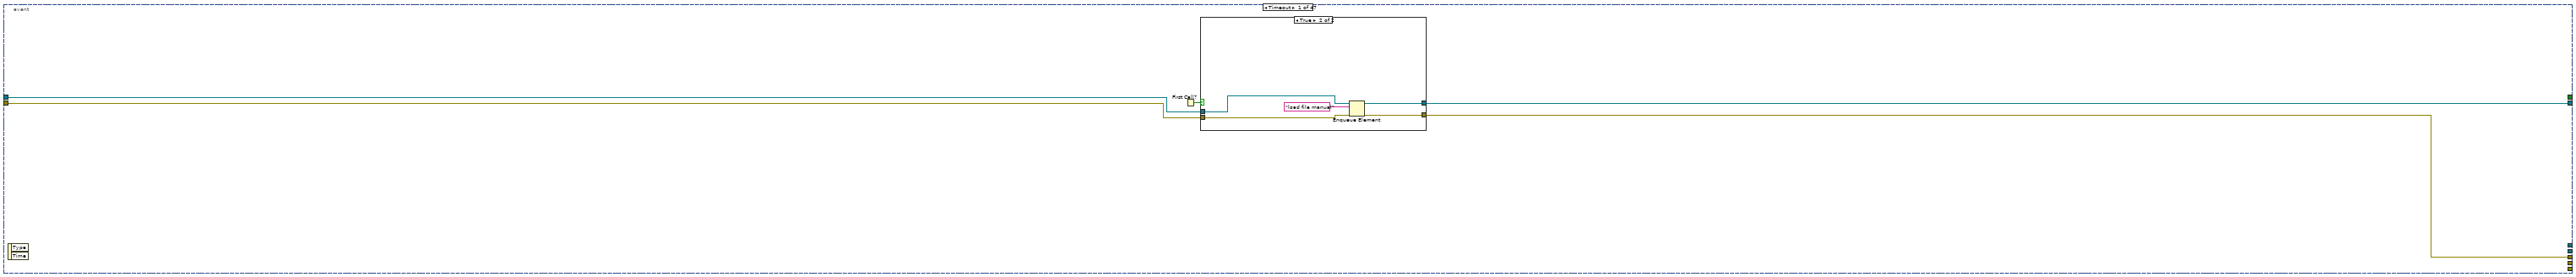
[diagram p3: hidden frame]
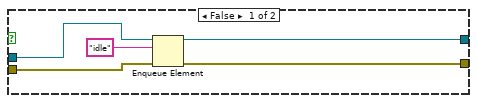
[diagram p4: hidden frame]
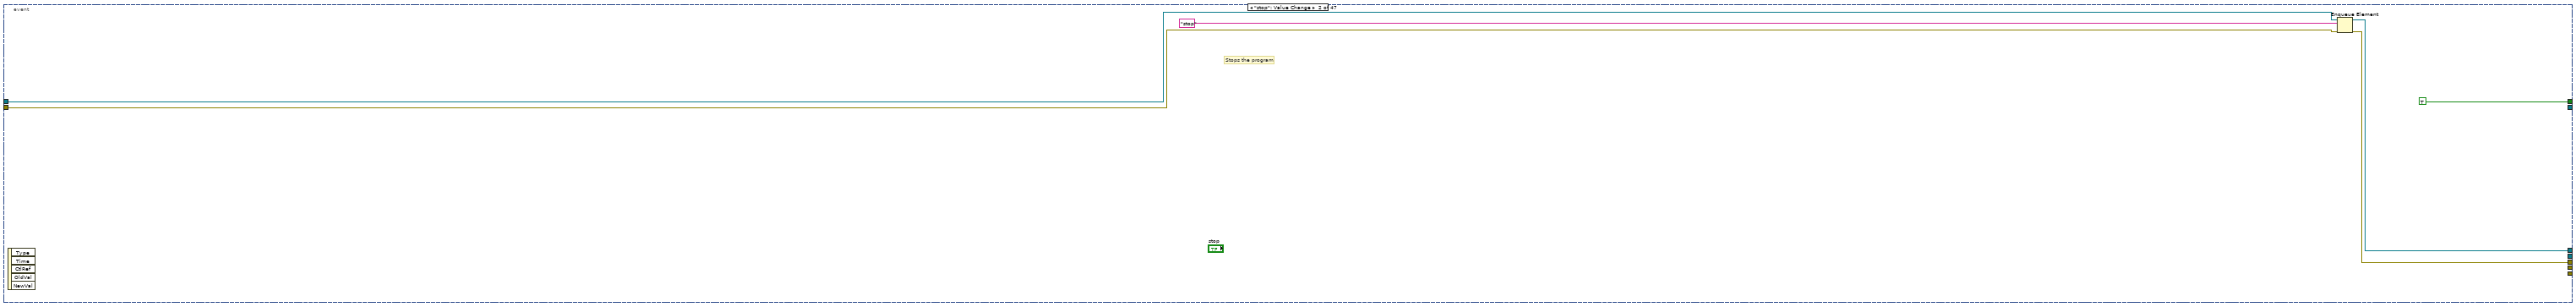
[diagram p5: hidden frame]
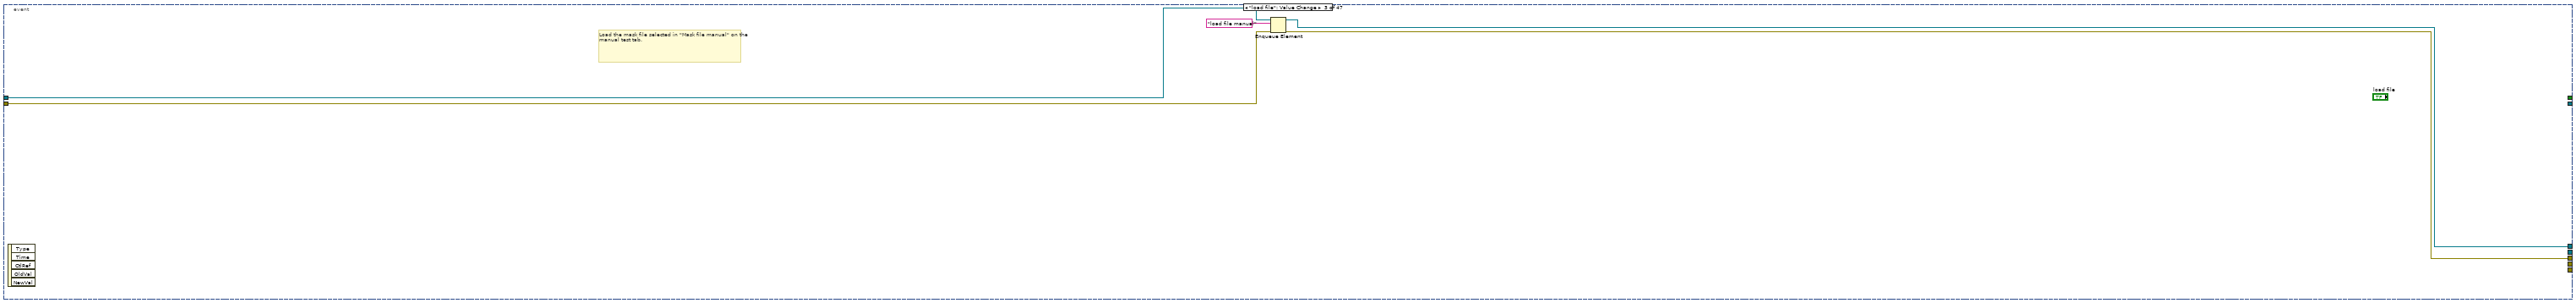
[diagram p6: hidden frame]
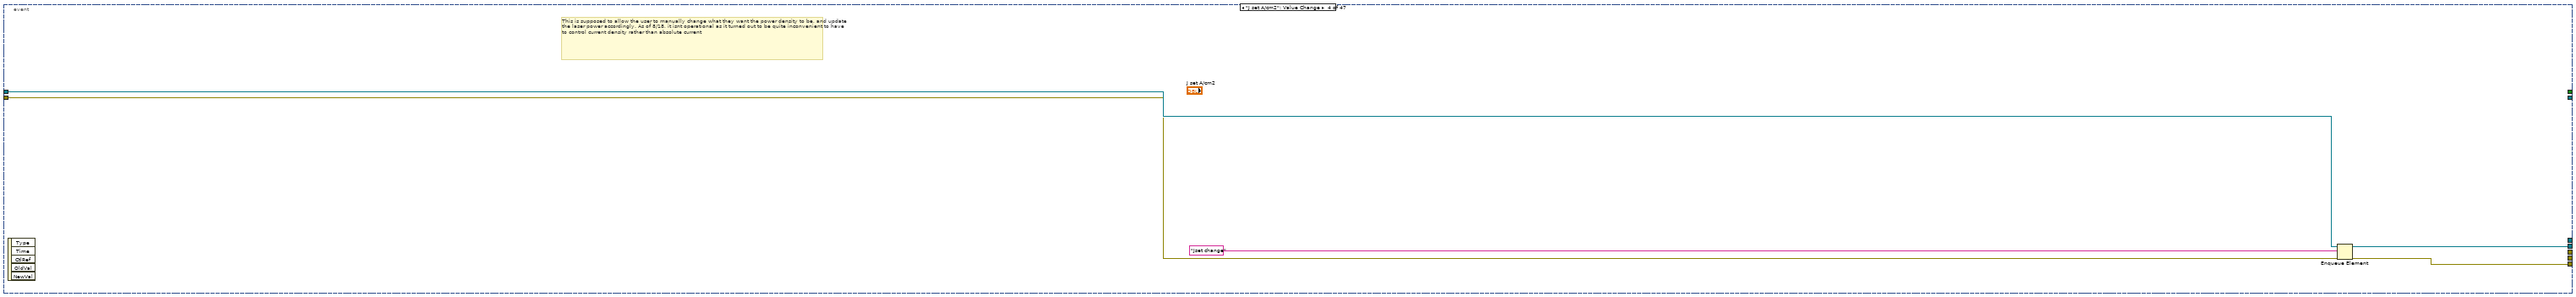
[diagram p7: hidden frame]
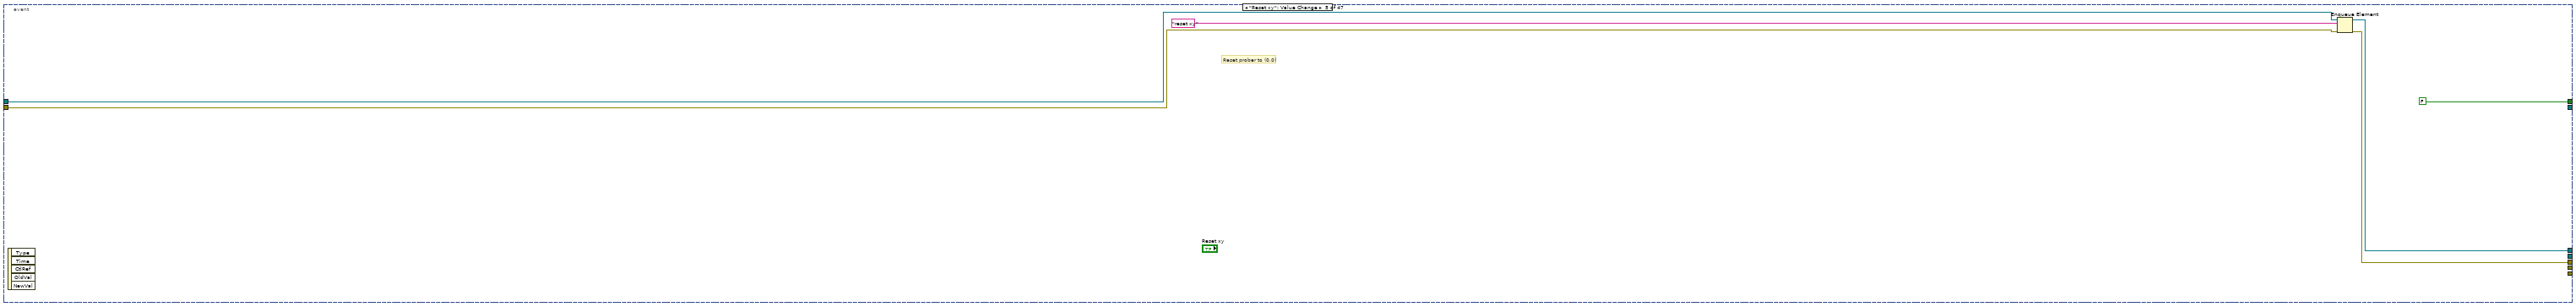
[diagram p8: hidden frame]
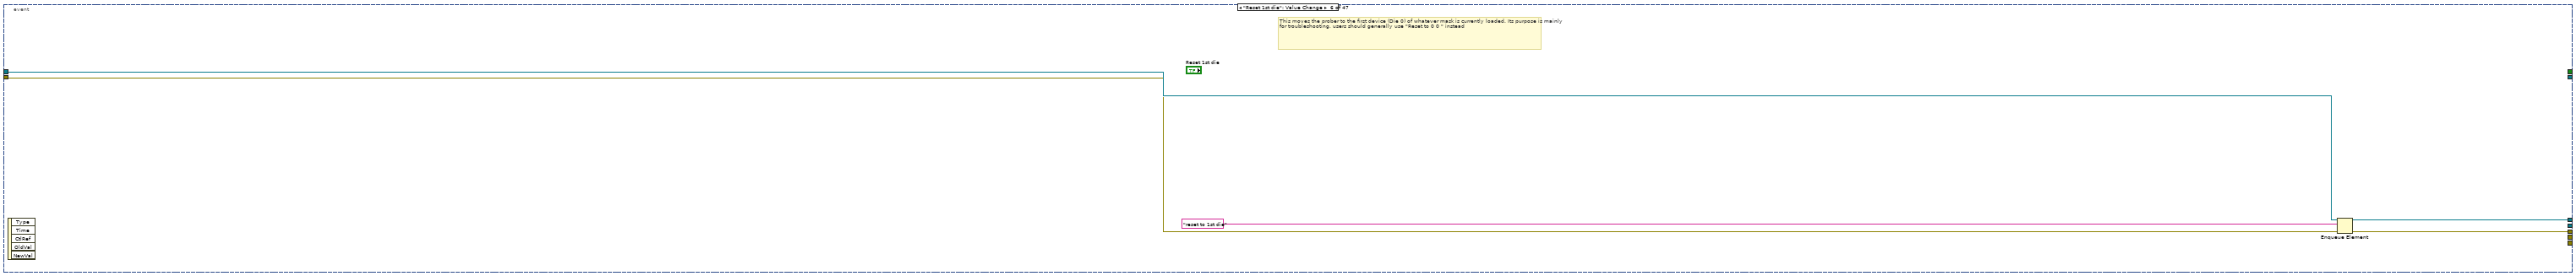
[diagram p9: hidden frame]
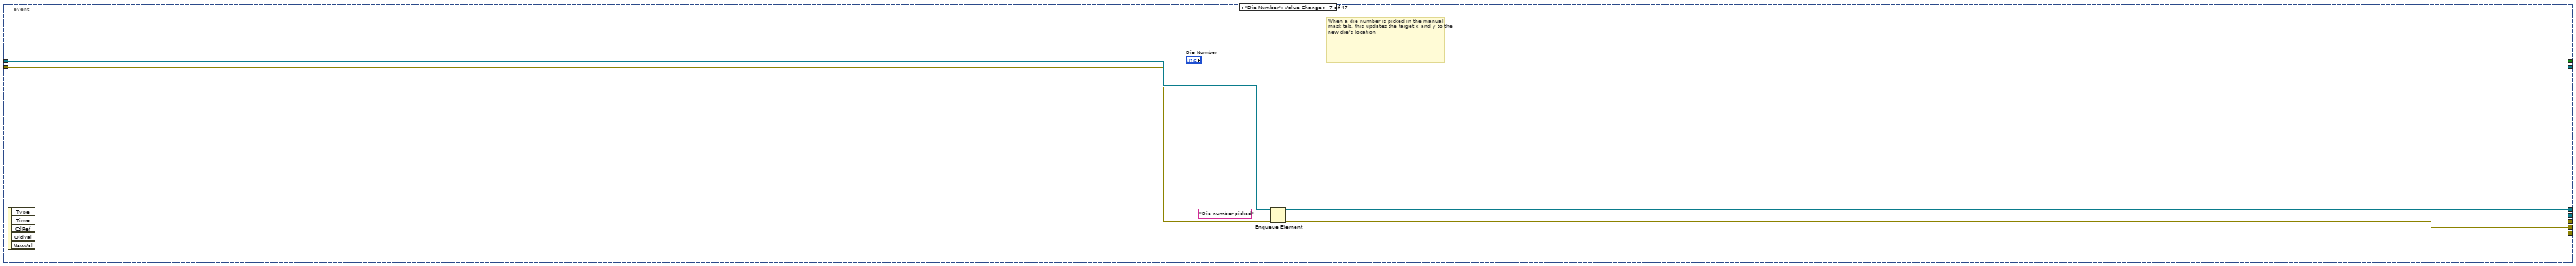
[diagram p10: hidden frame]
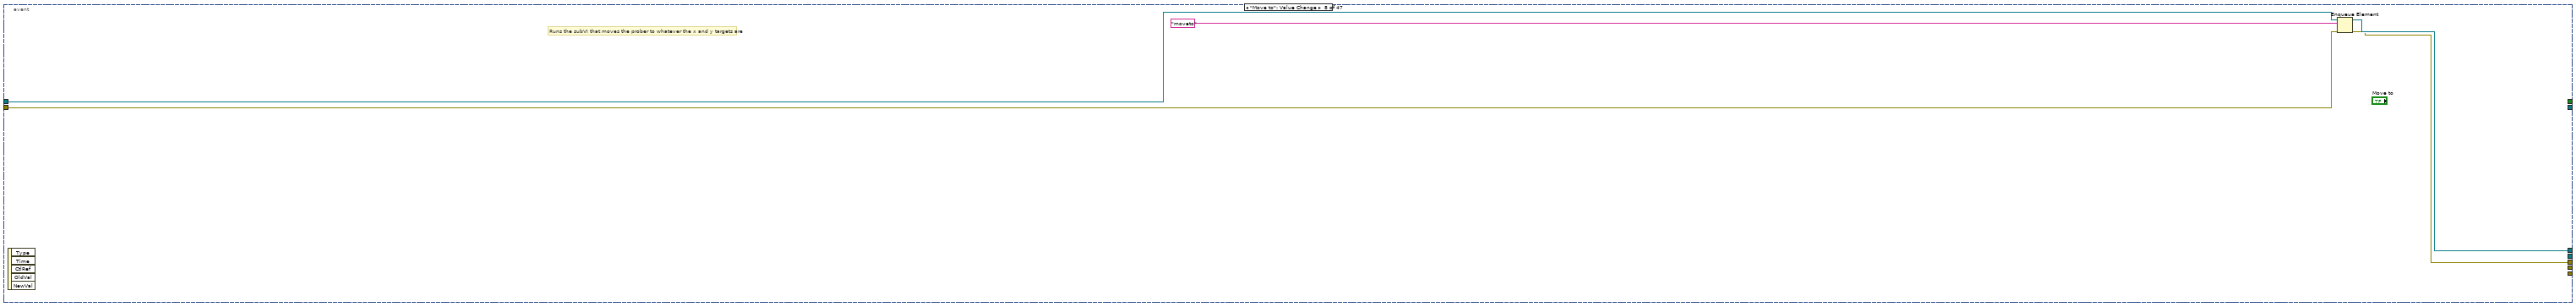
[diagram p11: hidden frame]
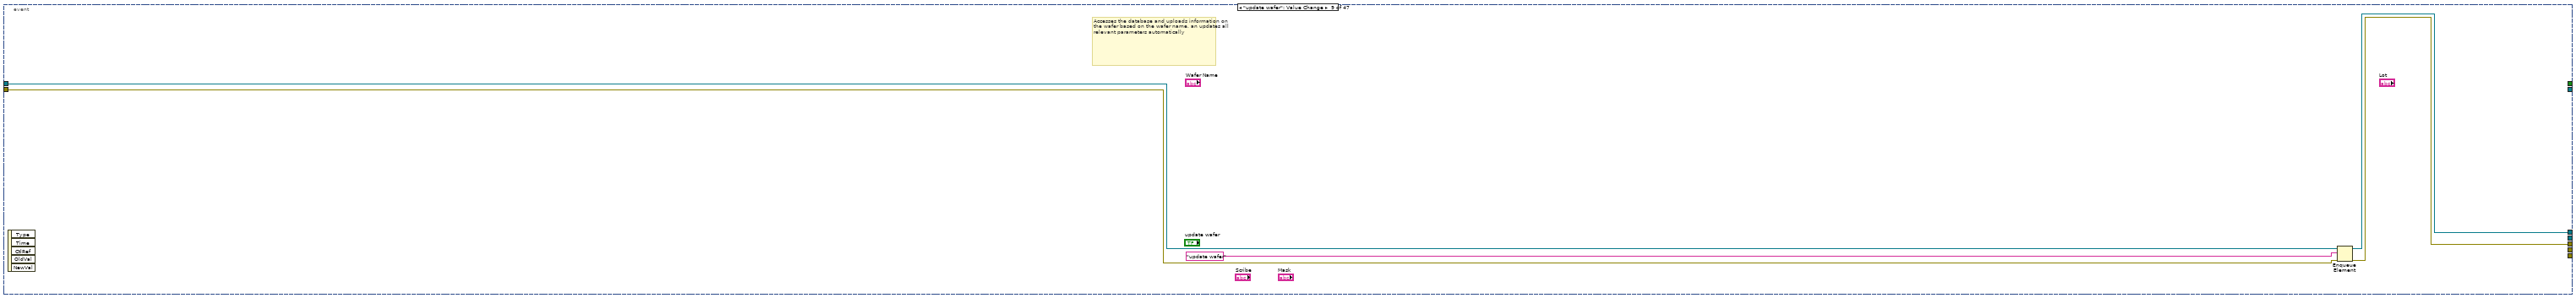
[diagram p12: hidden frame]
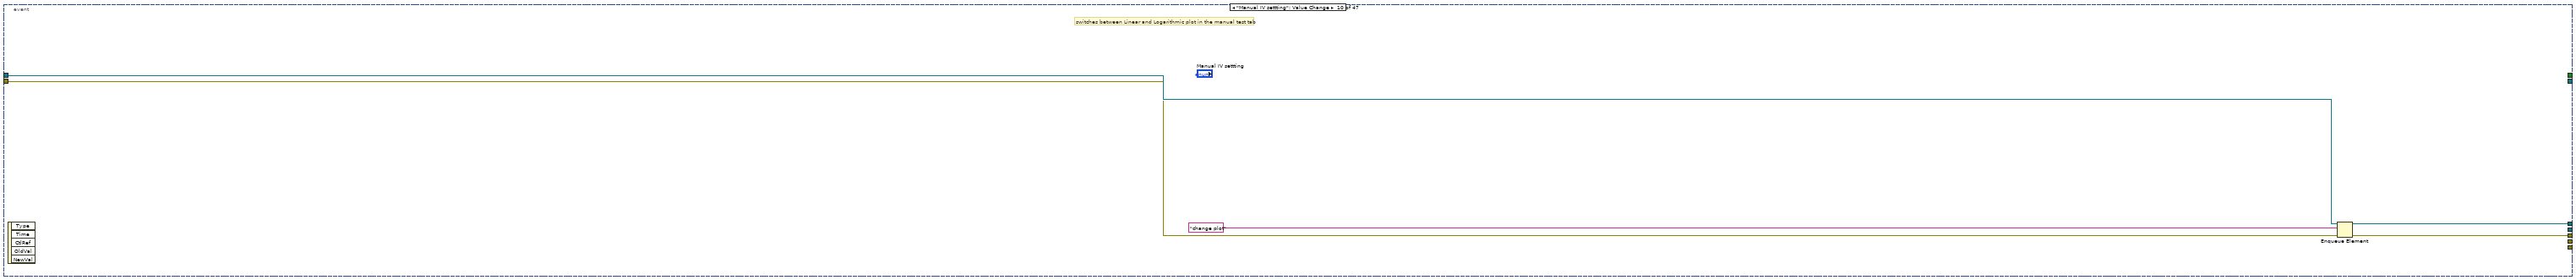
[diagram p13: hidden frame]
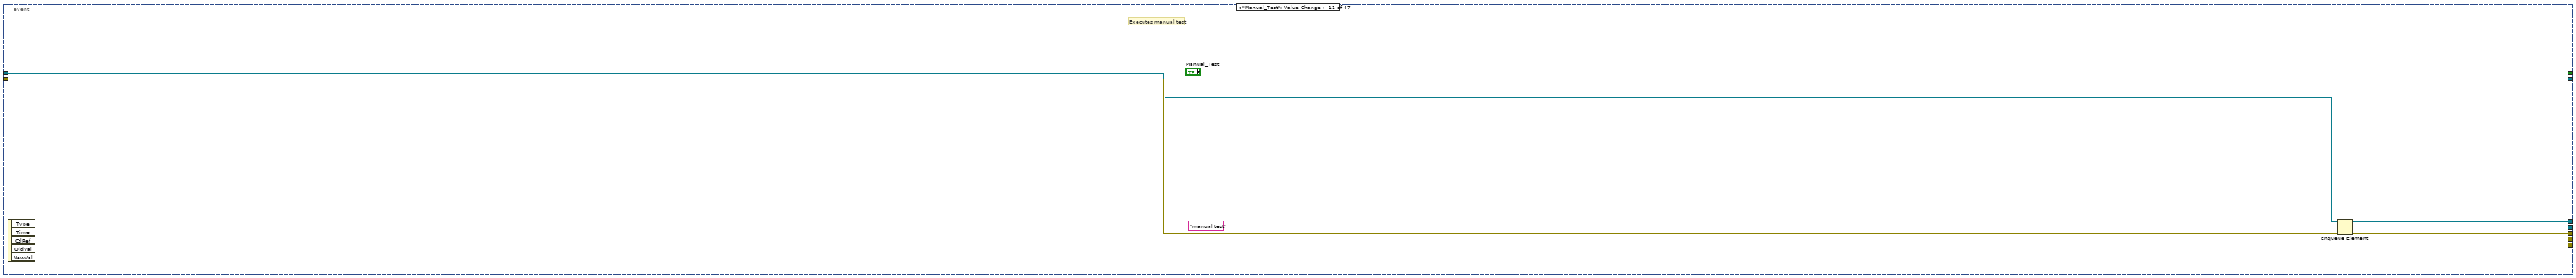
[diagram p14: hidden frame]
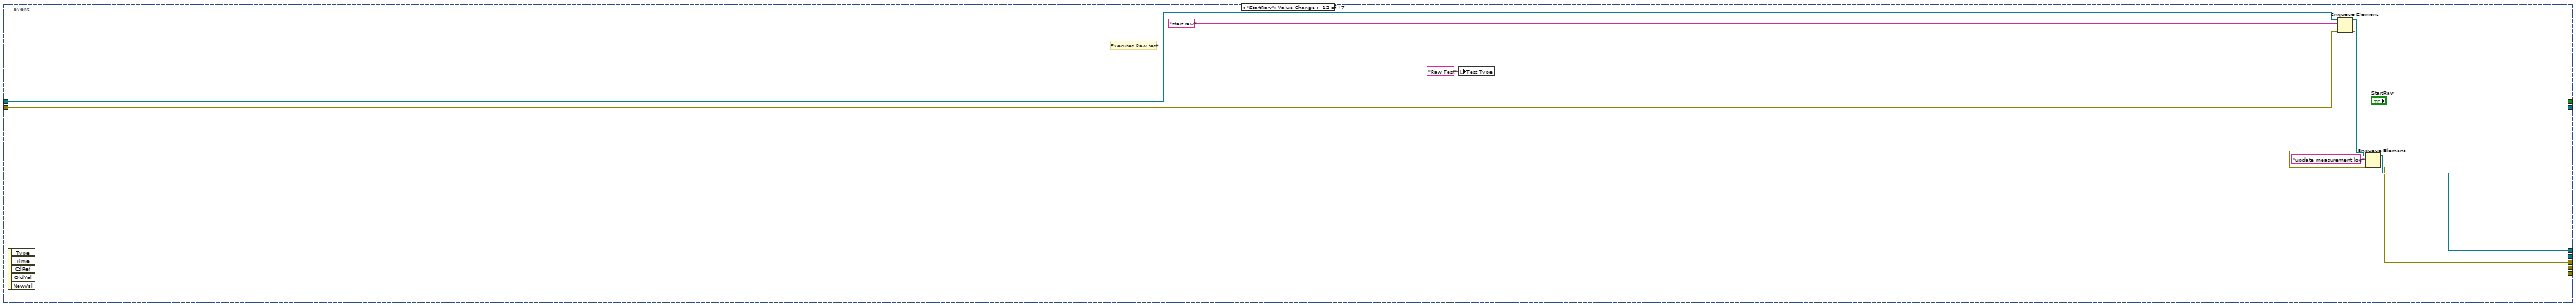
[diagram p15: hidden frame]
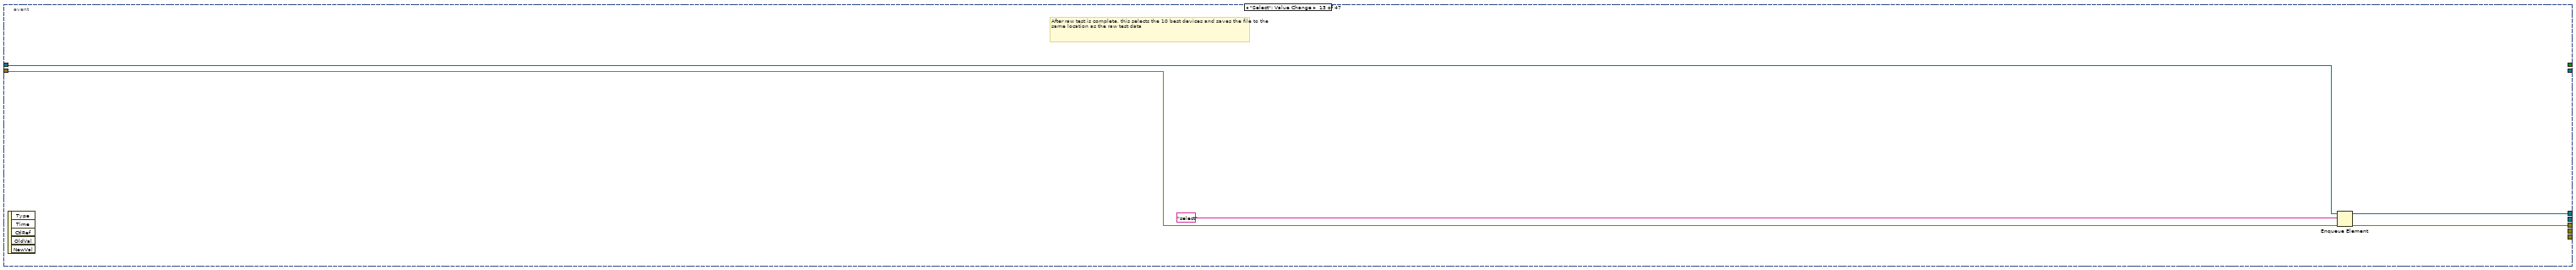
[diagram p16: hidden frame]
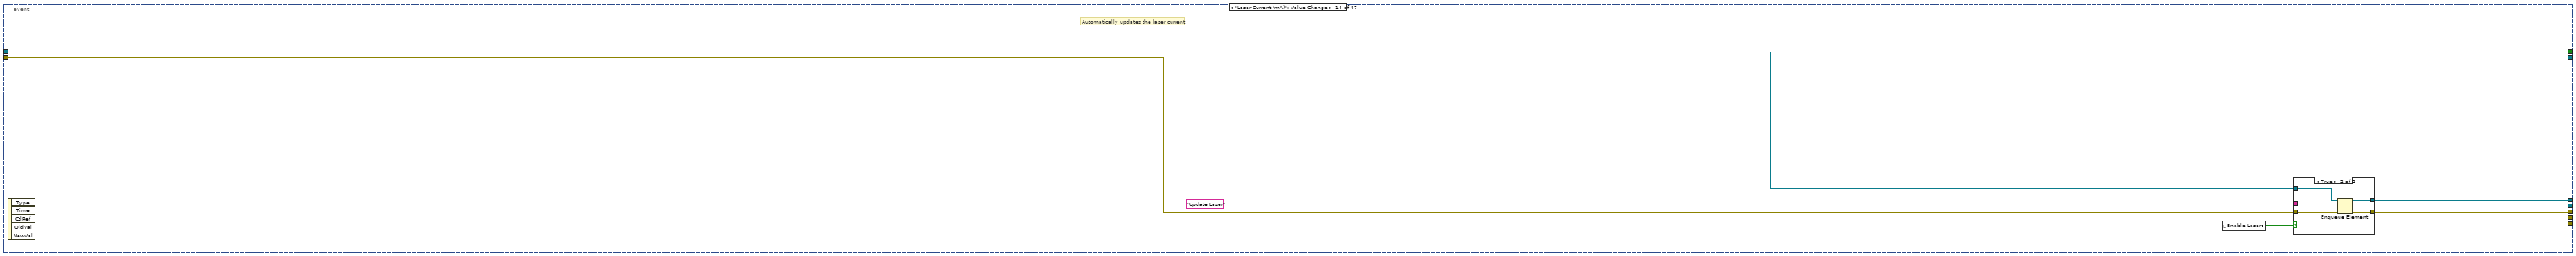
[diagram p17: hidden frame]
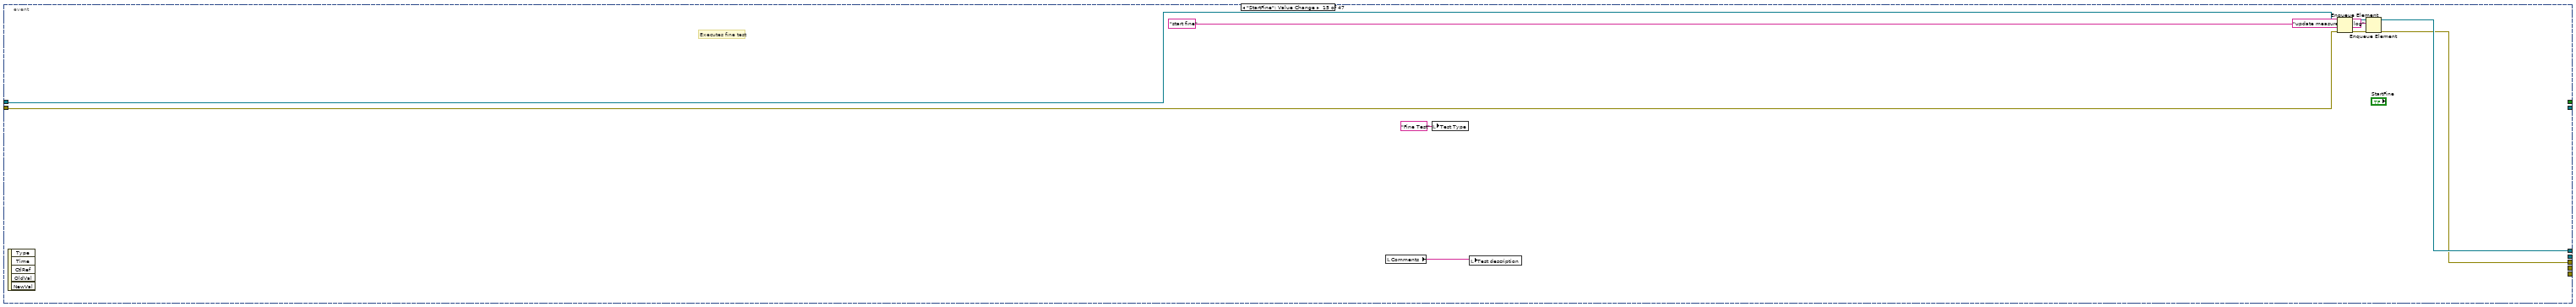
[diagram p19: hidden frame]
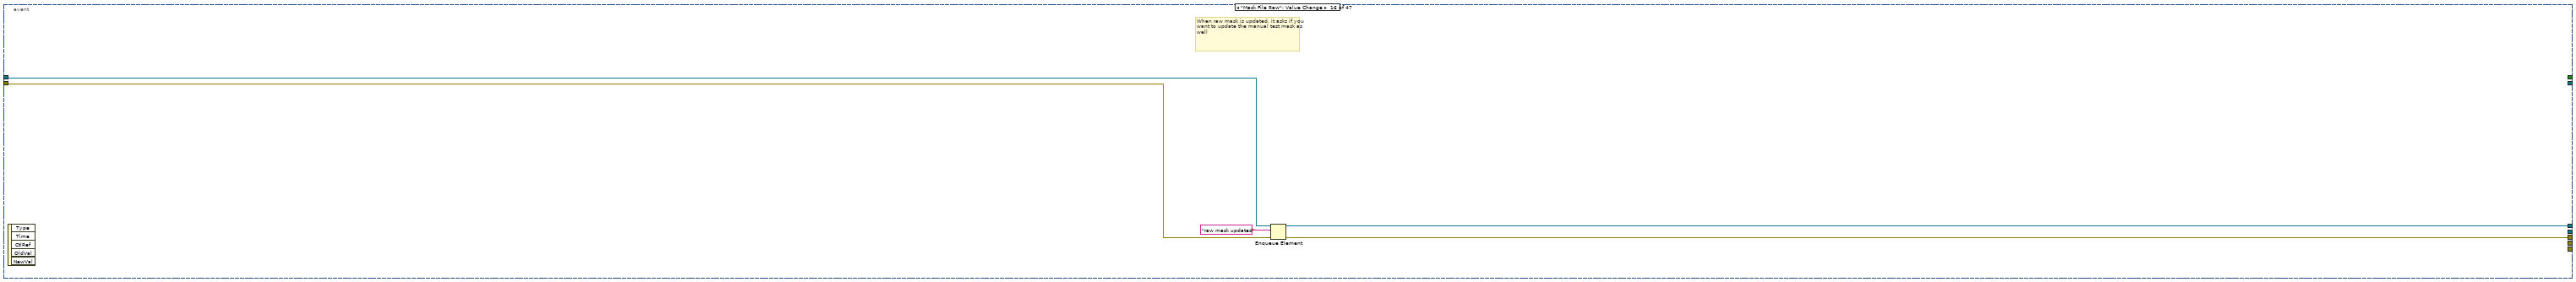
[diagram p20: hidden frame]
diagram:
  n1 = flat-sequence {
    tunnel: ["error in (no error)"] -> w1
    tunnel: w1 -> [w40]
    frame #0 {
      n2 = local read "Enable Laser"() -> (w2:bool)
      n3 = case shown="True" w2 {
        frame False {
        }
        frame True {
          n4 = flat-sequence {
            tunnel: [w10] -> w6
            tunnel: [w8] -> w5
            tunnel: w6 -> [w14]
            tunnel: w5 -> [w15]
            tunnel: [w14] -> w4
            tunnel: [w13] -> w3
            tunnel: w4 -> [w18]
            tunnel: w3 -> [w17]
            frame #0 {
              n5 = call <instrlib>:"TL4000 Initialize.vi"("error in (no error)"=errorcluster {"status"=FALSE, "code"=0, "source"=""}, "Reset Device (Reset Device)"=FALSE, "ID Query (Do Query)"=TRUE, "resource name"="TL4000 In") -> ("error out"=w8:errorcluster, "instrument handle out"=w10:refnum<visa-resource-name>)  [unwired: 6 in]
            }
            frame #1 {
              n6 = call <instrlib>:"TL4000 Switch TEC Output.vi"("error in (no error)"=w15, "TEC Output (Off)"=TRUE, "instrument handle"=w14) -> ("error out"=w13:errorcluster)  [unwired: 7 in, 1 out]
            }
            frame #2 {
              n7 = call <instrlib>:"TL4000 Switch LD Output.vi"("error in (no error)"=w17, "LD Output (Off)"=TRUE, "instrument handle"=w18) -> ("error out"=→"Laser Error":errorcluster)  [unwired: 7 in, 1 out]
            }
          }
        }
      }
    }
    frame #1 {
      w24 = FALSE ("Visible")
      n8 = call "getFile TestID.vi"("Path"="TestID file") -> ("TestID"=→"RawTest ID":u32)  [unwired: 9 in, 1 out]
      n9 = local write "Auto Temp Counter"(0 ("Auto Temp Counter")) -> ()
      n10 = property on="Test Type" class="Str"("Visible"=FALSE) -> ()  [unwired: 2 in, 2 out]
      n11 = Multiply(x="V compliance", y=0.95) -> (x*y=w28:dbl)
      n12 = property on="device name w skip" class="Str"("Visible"=w24) -> ()  [unwired: 2 in, 2 out]
      n13 = local write "Vmax"(w28) -> ()
      n14 = property on="no file" class="Bool (strict)"("Visible"=w24) -> ()  [unwired: 2 in, 2 out]
      "Counter" <- u32 0 ("Counter")
      "Laser Counter" <- u32 0 ("Counter")
      "WaferCounter" <- u32 0 ("Counter")
      "TempCounter" <- u32 0 ("Counter")
    }
    frame #2 {
      n15 = Obtain Queue(name (unnamed)="q", element data type="test" ("name (unnamed)"), create if not found? (T)=TRUE, error in (no error)=w40) -> (queue out=w42:refnum<queue>, error out=w41:errorcluster)  [unwired: 1 in, 1 out]
      n16 = while {
        shift-right: [w47] -> w43
        shift-left: w42 -> [w48]
        shift-right: [w45] -> w34
        shift-left: w41 -> [w46]
        stop <- w49 stop-if-true
        n17 = event shown="[18] \"Start auto\": Value Change" {
          selector: _ -> [_ _ _ _ _ _ _ _ _ _ _ _ _ _ _ _ _ _ _ _ _ _ _ _ _ _ _ _ _ _ _ _ _ _ _ _ _ _ _ _ _ _ _ _ _ _ _]
          dyn-events: _ -> [_ _ _ _ _ _ _ _ _ _ _ _ _ _ _ _ _ _ _ _ _ _ _ _ _ _ _ _ _ _ _ _ _ _ _ _ _ _ _ _ _ _ _ _ _ _ _]
          timeout: -1 -> [_ _ _ _ _ _ _ _ _ _ _ _ _ _ _ _ _ _ _ _ _ _ _ _ _ _ _ _ _ _ _ _ _ _ _ _ _ _ _ _ _ _ _ _ _ _ _]
          tunnel: [_ TRUE _ _ FALSE _ _ _ _ _ _ _ _ _ _ _ _ _ _ _ _ _ _ _ _ _ _ _ _ _ _ _ _ _ _ _ _ _ _ _ _ _ _ _ _ _ _] -> w49
          tunnel: w48 -> [w53 w65 w75 w80 w86 w91 w96 w100 w106 w111 w114 w125 w130 w135 w153 w158 w163 w168 w184 w290 w296 w301 w307 w310 w464 w469 w474 w479 w483 w488 w494 w503 w509 w514 w519 w524 w538 w543 w547 w552 w557 w563 w567 w572 w578 w586 w590]
          tunnel: [_ w69 w74 _ w85 w90 w95 w98 w104 w110 w113 w120 w128 w134 w147 w156 w161 w166 w182 w289 w294 w299 w305 w313 w462 w467 w472 w477 w481 w486 w492 w498 w507 w512 w518 w522 w533 w542 w544 w549 w556 w560 w565 w570 w576 w582 w588] -> w47
          tunnel: w46 -> [w52 w68 w73 w79 w83 w89 w94 w99 w105 w109 w115 w124 w129 w133 w152 w157 w162 w167 w183 w292 w295 w300 w306 w309 w463 w468 w473 w478 w482 w489 w493 w502 w508 w513 w517 w523 w537 w541 w546 w551 w555 w562 w566 w571 w577 w585 w589]
          tunnel: [w51 w67 w72 _ w84 w88 _ w97 w103 w108 w112 w119 w127 w132 w146 w155 w160 w165 w181 w291 w293 w298 w304 w312 w461 w466 w471 w476 w480 w487 w491 w497 w506 w511 w516 w521 w531 w540 w545 w550 w554 w559 w564 w569 w575 w580 w587] -> w45
          tunnel: [_ _ _ w78 _ _ _ _ _ _ _ _ _ _ _ _ _ _ _ _ _ _ _ _ _ _ _ _ _ _ _ _ _ _ _ _ _ _ _ _ _ _ _ _ _ _ _] -> _
          tunnel: [_ _ _ w77 _ _ _ _ _ _ _ _ _ _ _ _ _ _ _ _ _ _ _ _ _ _ _ _ _ _ _ _ _ _ _ _ _ _ _ _ _ _ _ _ _ _ _] -> _
          tunnel: [w50 _ _ _ _ _ _ _ _ _ _ _ _ _ _ _ _ _ _ _ _ _ _ _ _ _ _ _ _ _ _ _ _ _ _ _ _ _ _ _ _ _ _ _ _ _ _] -> _
          tunnel: [_ _ _ _ _ _ w93 _ _ _ _ _ _ _ _ _ _ _ _ _ _ _ _ _ _ _ _ _ _ _ _ _ _ _ _ _ _ _ _ _ _ _ _ _ _ _ _] -> _
          event Timeout {
            n18 = event-data() -> ()  [unwired: 1 in, 2 out]
            n19 = First Call?() -> (First Call?: T/F=w54:bool)
            n20 = case shown="True" w54 {
              tunnel: w52 -> [w57 w63]
              tunnel: w53 -> [w59 w64]
              tunnel: [w56 w62] -> w51
              tunnel: [w58 w61] -> w50
              frame False {
                n21 = Enqueue Element(queue=w59, element="idle", error in (no error)=w57) -> (queue out=w58:refnum<queue>, error out=w56:errorcluster)  [unwired: 1 in, 1 out]
              }
              frame True {
                n22 = Enqueue Element(queue=w64, element="load file manual", error in (no error)=w63) -> (queue out=w61:refnum<queue>, error out=w62:errorcluster)  [unwired: 1 in, 1 out]
              }
            }
          }
          event "stop": Value Change {
            # "Stops the program"
            n23 = event-data() -> ()  [unwired: 1 in, 5 out]
            n24 = Enqueue Element(queue=w65, element="stop", error in (no error)=w68) -> (queue out=w69:refnum<queue>, error out=w67:errorcluster)  [unwired: 1 in, 1 out]
          }
          event "load file": Value Change {
            # "Load the mask file selected in \"Mask file manual\" on the manual test tab."
            n25 = event-data() -> ()  [unwired: 1 in, 5 out]
            n26 = Enqueue Element(queue=w75, element="load file manual", error in (no error)=w73) -> (queue out=w74:refnum<queue>, error out=w72:errorcluster)  [unwired: 1 in, 1 out]
          }
          event "J set A/cm2": Value Change {
            # "This is supposed to allow the user to manually change what they want the power density to be, and update the laser power accordingly. As of 8/18, it isnt operational as it turned out to be quite inconvenient to have to control current density rather than absolute current"
            n27 = event-data() -> ()  [unwired: 1 in, 5 out]
            n28 = Enqueue Element(queue=w80, element="Jset change", error in (no error)=w79) -> (queue out=w78:refnum<queue>, error out=w77:errorcluster)  [unwired: 1 in, 1 out]
          }
          event "Reset xy": Value Change {
            # "Reset prober to (0,0)"
            n29 = event-data() -> ()  [unwired: 1 in, 5 out]
            n30 = Enqueue Element(queue=w86, element="reset xy", error in (no error)=w83) -> (queue out=w85:refnum<queue>, error out=w84:errorcluster)  [unwired: 1 in, 1 out]
          }
          event "Reset 1st die": Value Change {
            # "This moves the prober to the first device (Die 0) of whatever mask is currently loaded. Its purpose is mainly for troubleshooting, users should generally use \"Reset to 0 0 \" instead"
            n31 = event-data() -> ()  [unwired: 1 in, 5 out]
            n32 = Enqueue Element(queue=w91, element="reset to 1st die", error in (no error)=w89) -> (queue out=w90:refnum<queue>, error out=w88:errorcluster)  [unwired: 1 in, 1 out]
          }
          event "Die Number": Value Change {
            # "When a die number is picked in the manual mask tab, this updates the target x and y to the new die's location"
            n33 = event-data() -> ()  [unwired: 1 in, 5 out]
            n34 = Enqueue Element(queue=w96, element="Die number picked", error in (no error)=w94) -> (queue out=w95:refnum<queue>, error out=w93:errorcluster)  [unwired: 1 in, 1 out]
          }
          event "Move to": Value Change {
            # "Runs the subVI that moves the prober to whatever the x and y targets are"
            n35 = event-data() -> ()  [unwired: 1 in, 5 out]
            n36 = Enqueue Element(queue=w100, element="moveto", error in (no error)=w99) -> (queue out=w98:refnum<queue>, error out=w97:errorcluster)  [unwired: 1 in, 1 out]
          }
          event "update wafer": Value Change {
            # "Accesses the database and uploads information on the wafer based on the wafer name, an updates all relevant parameters automatically"
            n37 = event-data() -> ()  [unwired: 1 in, 5 out]
            n38 = Enqueue Element(queue=w106, element="update wafer", error in (no error)=w105) -> (queue out=w104:refnum<queue>, error out=w103:errorcluster)  [unwired: 1 in, 1 out]
          }
          event "Manual IV settting": Value Change {
            # "switches between Linear and Logarithmic plot in the manual test tab"
            n39 = event-data() -> ()  [unwired: 1 in, 5 out]
            n40 = Enqueue Element(queue=w111, element="change plot", error in (no error)=w109) -> (queue out=w110:refnum<queue>, error out=w108:errorcluster)  [unwired: 1 in, 1 out]
          }
          event "Manual_Test": Value Change {
            # "Executes manual test"
            n41 = event-data() -> ()  [unwired: 1 in, 5 out]
            n42 = Enqueue Element(queue=w114, element="manual test", error in (no error)=w115) -> (queue out=w113:refnum<queue>, error out=w112:errorcluster)  [unwired: 1 in, 1 out]
          }
          event "StartRaw": Value Change {
            # "Executes Raw test"
            n43 = event-data() -> ()  [unwired: 1 in, 5 out]
            n44 = local write "Test Type"("Raw Test" ("Test Type")) -> ()
            n45 = Enqueue Element(queue=w125, element="start raw", error in (no error)=w124) -> (queue out=w121:refnum<queue>, error out=w118:errorcluster)  [unwired: 1 in, 1 out]
            n46 = Enqueue Element(queue=w121, element="update measurement log", error in (no error)=w118) -> (queue out=w120:refnum<queue>, error out=w119:errorcluster)  [unwired: 1 in, 1 out]
          }
          event "Select": Value Change {
            # "After raw test is complete, this selects the 10 best devices and saves the file to the same location as the raw test data"
            n47 = event-data() -> ()  [unwired: 1 in, 5 out]
            n48 = Enqueue Element(queue=w130, element="select", error in (no error)=w129) -> (queue out=w128:refnum<queue>, error out=w127:errorcluster)  [unwired: 1 in, 1 out]
          }
          event "Laser Current (mA)": Value Change {
            # "Automatically updates the laser current"
            n49 = event-data() -> ()  [unwired: 1 in, 5 out]
            n50 = local read "Enable Laser"() -> (w131:bool)
            n51 = case shown="True" w131 {
              tunnel: "Update Laser" ("element") -> [_ w143]
              tunnel: w135 -> [w138 w142]
              tunnel: [w138 w141] -> w134
              tunnel: w133 -> [w137 w140]
              tunnel: [w137 w139] -> w132
              frame False {
              }
              frame True {
                n52 = Enqueue Element(queue=w142, element=w143, error in (no error)=w140) -> (queue out=w141:refnum<queue>, error out=w139:errorcluster)  [unwired: 1 in, 1 out]
              }
            }
          }
          event "StartFine": Value Change {
            # "Executes fine test"
            n53 = event-data() -> ()  [unwired: 1 in, 5 out]
            n54 = local read "Comments"() -> (w144:string)
            n55 = local write "Test Type"("Fine Test" ("Test Type")) -> ()
            n56 = local write "Test description"(w144) -> ()
            n57 = Enqueue Element(queue=w153, element="start fine", error in (no error)=w152) -> (queue out=w149:refnum<queue>, error out=w148:errorcluster)  [unwired: 1 in, 1 out]
            n58 = Enqueue Element(queue=w149, element="update measurement log", error in (no error)=w148) -> (queue out=w147:refnum<queue>, error out=w146:errorcluster)  [unwired: 1 in, 1 out]
          }
          event "Mask File Raw": Value Change {
            # "When raw mask is updated, it asks if you want to update the manual test mask as well"
            n59 = event-data() -> ()  [unwired: 1 in, 5 out]
            n60 = Enqueue Element(queue=w158, element="raw mask updated", error in (no error)=w157) -> (queue out=w156:refnum<queue>, error out=w155:errorcluster)  [unwired: 1 in, 1 out]
          }
          event "Mask File Manual": Value Change {
            # "When manual mask is updated, it asks if the user would want to update the raw test as well"
            n61 = event-data() -> ()  [unwired: 1 in, 5 out]
            n62 = Enqueue Element(queue=w163, element="mask manual update", error in (no error)=w162) -> (queue out=w161:refnum<queue>, error out=w160:errorcluster)  [unwired: 1 in, 1 out]
          }
          event "Load raw": Value Change {
            # "Gives the user the option to pick a raw data file, and then displays that on the graphical display on the raw test tab"
            n63 = event-data() -> ()  [unwired: 1 in, 5 out]
            n64 = Enqueue Element(queue=w168, element="load raw data", error in (no error)=w167) -> (queue out=w166:refnum<queue>, error out=w165:errorcluster)  [unwired: 1 in, 1 out]
          }
          event "Start auto": Value Change {
            # "Exectues Auto Test:\n1) For loop - repeats as many times as there are test names.\n2) Skip raw? - check to see if the user would like to skip raw test (see guide). If raw test is skipped, the variable \"Raw test skipped\" is set to TRUE\n3) Case Structure - If the laser is enabled, the program sets the laser current to zero prior to the raw test.; if the user has elected to disable the laser, then this step is skipped\n4) Start Raw - The raw test is executed. If the raw test is skipped, this element is still queued up, and the entire test is skipped within the event structure. This is because the timing didn't work when I tried to skip the raw test here.\n5)Select - This selects the best ten devices. Again, if raw test is skipped, this still is added to the queue, and is skipped in the event structure\n6) Double Case Structure - There are 4 options\n         a) Laser Disabled & Only Raw test TRUE -  The entire fine test portion is skipped\n         b)  Laser Disabled & Only Raw Test FALSE - The fine test is run ONLY dark. Find best devices mask still queues up, but only runs if the raw test has been skipped\n         c) Laser Enabled - Only Raw Test TRUE - the entire fine test is still skipped\n         d) Laser Enabled - Only Raw Test FALSE - fine test is run through a for loop that repeats the test for every laser power in the Laser List. Find best devices mask only runs if the raw test is skipped.\n7) Reset skip - replaces the (skip) on the device name if the raw test was skipped, as for the duration of the test it had to be removed. This is in case multiple tests are to be run - so the user doesn't have to keep specifying that they want to skip the raw test every time they run the auto test\n8) Zero/Update Laser - Turns the laser to zero after the test is complete\n9) Update Measurement log - automatically updates the measurement lof with the details of the test"
            n65 = event-data() -> ()  [unwired: 1 in, 1 out]
            n66 = local read "Test description"() -> (w179:string)
            n67 = property on="Auto Temperature List" class="LstBox (strict)"() -> ("Item Names"=w177:string[])  [unwired: 2 in, 2 out]
            n68 = local write "Test Type"("Auto Test" ("Test Type")) -> ()
            n69 = local write "Comments"(w179) -> ()
            n70 = for {
              tunnel: w184 -> [w195]
              tunnel: w183 -> [w194]
              tunnel: [w198] -> w176
              tunnel: [w197] -> w173
              tunnel: w177 -> [_] mode=indexing
              n71 = Enqueue Element(queue=w195, element="select temperature", error in (no error)=w194) -> (queue out=w189:refnum<queue>, error out=w187:errorcluster)  [unwired: 1 in, 1 out]
              n72 = Enqueue Element(queue=w189, element="update temperature", error in (no error)=w187) -> (queue out=w188:refnum<queue>, error out=w186:errorcluster)  [unwired: 1 in, 1 out]
              n73 = Enqueue Element(queue=w188, element="wait for temperature", error in (no error)=w186) -> (queue out=w193:refnum<queue>, error out=w192:errorcluster)  [unwired: 1 in, 1 out]
              n74 = property on="Test List" class="LstBox (strict)"() -> ("Item Names"=w204:string[])  [unwired: 2 in, 2 out]
              n75 = for {
                shift-right: [w205] -> w201
                shift-left: w192 -> [w213]
                shift-right: [w208] -> w202
                shift-left: w193 -> [w214]
                tunnel: w204 -> [_] mode=indexing
                n76 = Enqueue Element(queue=w214, element="skip raw?", error in (no error)=w213) -> (queue out=w212:refnum<queue>, error out=w211:errorcluster)  [unwired: 1 in, 1 out]
                n77 = Enqueue Element(queue=w212, element="pick device", error in (no error)=w211) -> (queue out=w220:refnum<queue>, error out=w219:errorcluster)  [unwired: 1 in, 1 out]
                n78 = case shown="False" FALSE {
                  tunnel: w220 -> [w273 w286]
                  tunnel: w219 -> [w272 w287]
                  tunnel: [w270 w286] -> w218
                  tunnel: [w269 w287] -> w217
                  frame False {
                    n79 = local read "Enable Laser"() -> (w271:bool)
                    n80 = case shown="True" w271 {
                      tunnel: [w277 w285] -> w275
                      tunnel: [w276 w284] -> w274
                      tunnel: w273 -> [w277 w282]
                      tunnel: w272 -> [w276 w280]
                      frame False {
                      }
                      frame True {
                        n81 = Enqueue Element(queue=w282, element="Zero Laser", error in (no error)=w280) -> (queue out=w281:refnum<queue>, error out=w279:errorcluster)  [unwired: 1 in, 1 out]
                        n82 = Enqueue Element(queue=w281, element="Update Laser", error in (no error)=w279) -> (queue out=w285:refnum<queue>, error out=w284:errorcluster)  [unwired: 1 in, 1 out]
                      }
                    }
                    n83 = Enqueue Element(queue=w275, element="start raw", error in (no error)=w274) -> (queue out=w266:refnum<queue>, error out=w265:errorcluster)  [unwired: 1 in, 1 out]
                    n84 = Enqueue Element(queue=w266, element="select", error in (no error)=w265) -> (queue out=w270:refnum<queue>, error out=w269:errorcluster)  [unwired: 1 in, 1 out]
                  }
                  frame True {
                  }
                }
                n85 = local read "Enable Laser"() -> (w215:bool)
                n86 = case shown="True" w215 {
                  tunnel: [w227 w243] -> w209
                  tunnel: [w226 w242] -> w206
                  tunnel: w218 -> [w225 w241]
                  tunnel: w217 -> [w224 w240]
                  frame False {
                    n87 = local read "Only Raw Test"() -> (w222:bool)
                    n88 = Not(x=w222) -> (.not. x?=w223:bool)
                    n89 = case shown="False" w223 {
                      tunnel: [w229 w237] -> w227
                      tunnel: [w228 w236] -> w226
                      tunnel: w225 -> [w229 w235]
                      tunnel: w224 -> [w228 w233]
                      frame False {
                      }
                      frame True {
                        n90 = Enqueue Element(queue=w235, element="find best devices mask", error in (no error)=w233) -> (queue out=w234:refnum<queue>, error out=w232:errorcluster)  [unwired: 1 in, 1 out]
                        n91 = Enqueue Element(queue=w234, element="start fine", error in (no error)=w232) -> (queue out=w237:refnum<queue>, error out=w236:errorcluster)  [unwired: 1 in, 1 out]
                      }
                    }
                  }
                  frame True {
                    n92 = Not(x="Only Raw Test") -> (.not. x?=w238:bool)
                    n93 = case shown="True" w238 {
                      tunnel: [w245 w250] -> w243
                      tunnel: [w244 w249] -> w242
                      tunnel: w241 -> [w245 w248]
                      tunnel: w240 -> [w244 w247]
                      frame False {
                      }
                      frame True {
                        n94 = property on="Laser List" class="LstBox (strict)"() -> ("Item Names"=w246:string[])  [unwired: 2 in, 2 out]
                        n95 = for {
                          tunnel: [w264] -> w250
                          tunnel: [w263] -> w249
                          tunnel: w248 -> [w259]
                          tunnel: w247 -> [w262]
                          tunnel: w246 -> [_] mode=indexing
                          n96 = Enqueue Element(queue=w259, element="pick laser", error in (no error)=w262) -> (queue out=w258:refnum<queue>, error out=w260:errorcluster)  [unwired: 1 in, 1 out]
                          n97 = Enqueue Element(queue=w258, element="Update Laser", error in (no error)=w260) -> (queue out=w253:refnum<queue>, error out=w256:errorcluster)  [unwired: 1 in, 1 out]
                          n98 = Enqueue Element(queue=w253, element="find best devices mask", error in (no error)=w256) -> (queue out=w254:refnum<queue>, error out=w255:errorcluster)  [unwired: 1 in, 1 out]
                          n99 = Enqueue Element(queue=w254, element="start fine", error in (no error)=w255) -> (queue out=w264:refnum<queue>, error out=w263:errorcluster)  [unwired: 1 in, 1 out]
                        }
                      }
                    }
                  }
                }
                n100 = Enqueue Element(queue=w209, element="reset skip", error in (no error)=w206) -> (queue out=w208:refnum<queue>, error out=w205:errorcluster)  [unwired: 1 in, 1 out]
              }
              n101 = Enqueue Element(queue=w202, element="Zero Laser", error in (no error)=w201) -> (queue out=w200:refnum<queue>, error out=w199:errorcluster)  [unwired: 1 in, 1 out]
              n102 = Enqueue Element(queue=w200, element="update laser", error in (no error)=w199) -> (queue out=w198:refnum<queue>, error out=w197:errorcluster)  [unwired: 1 in, 1 out]
            }
            n103 = Enqueue Element(queue=w176, element="temp to 25", error in (no error)=w173) -> (queue out=w175:refnum<queue>, error out=w172:errorcluster)  [unwired: 1 in, 1 out]
            n104 = Enqueue Element(queue=w175, element="update temperature", error in (no error)=w172) -> (queue out=w174:refnum<queue>, error out=w171:errorcluster)  [unwired: 1 in, 1 out]
            n105 = Enqueue Element(queue=w174, element="update measurement log", error in (no error)=w171) -> (queue out=w182:refnum<queue>, error out=w181:errorcluster)  [unwired: 1 in, 1 out]
          }
          event "Generate Report": Value Change {
            n106 = event-data() -> ()  [unwired: 1 in, 5 out]
            n107 = Enqueue Element(queue=w290, element="generate prelim report", error in (no error)=w292) -> (queue out=w289:refnum<queue>, error out=w291:errorcluster)  [unwired: 1 in, 1 out]
          }
          event "Add to Temp Auto": Value Change {
            n108 = event-data() -> ()  [unwired: 1 in, 5 out]
            n109 = Enqueue Element(queue=w296, element="add temp auto", error in (no error)=w295) -> (queue out=w294:refnum<queue>, error out=w293:errorcluster)  [unwired: 1 in, 1 out]
          }
          event "Remove from Temp Auto": Value Change {
            n110 = event-data() -> ()  [unwired: 1 in, 5 out]
            n111 = Enqueue Element(queue=w301, element="remove temp auto", error in (no error)=w300) -> (queue out=w299:refnum<queue>, error out=w298:errorcluster)  [unwired: 1 in, 1 out]
          }
          event "Clear temp list Auto": Value Change {
            n112 = event-data() -> ()  [unwired: 1 in, 5 out]
            n113 = Enqueue Element(queue=w307, element="clear temp auto", error in (no error)=w306) -> (queue out=w305:refnum<queue>, error out=w304:errorcluster)  [unwired: 1 in, 1 out]
          }
          event "begin lot test": Value Change {
            n114 = event-data() -> ()  [unwired: 1 in, 5 out]
            n115 = local write "Test Type"("Lot Test" ("Test Type")) -> ()
            n116 = property on="Wafer List" class="LstBox (strict)"() -> ("Item Names"=w311:string[])  [unwired: 2 in, 2 out]
            n117 = for {
              tunnel: w311 -> [_] mode=indexing
              shift-right: [w321] -> w313
              shift-left: w310 -> [w340]
              shift-right: [w320] -> w312
              shift-left: w309 -> [w339]
              i -> [w338]
              n118 = Equal?(x=w338, y=0) -> (x = y?=w336:bool)
              n119 = And(x="First Wafer Loaded?", y=w336) -> (x .and. y?=w334:bool)
              n120 = case shown="False" w334 {
                tunnel: w340 -> [w447 w459]
                tunnel: w339 -> [w446 w458]
                tunnel: [w445 w459] -> w333
                tunnel: [w444 w458] -> w328
                frame False {
                  n121 = Enqueue Element(queue=w447, element="load wafer", error in (no error)=w446) -> (queue out=w452:refnum<queue>, error out=w451:errorcluster)  [unwired: 1 in, 1 out]
                  n122 = Enqueue Element(queue=w452, element="wait", error in (no error)=w451) -> (queue out=w450:refnum<queue>, error out=w449:errorcluster)  [unwired: 1 in, 1 out]
                  n123 = Enqueue Element(queue=w450, element="profile z", error in (no error)=w449) -> (queue out=w455:refnum<queue>, error out=w454:errorcluster)  [unwired: 1 in, 1 out]
                  n124 = Enqueue Element(queue=w455, element="auto align", error in (no error)=w454) -> (queue out=w445:refnum<queue>, error out=w444:errorcluster)  [unwired: 1 in, 1 out]
                }
                frame True {
                }
              }
              n125 = property on="Auto Temperature List" class="LstBox (strict)"() -> ("Item Names"=w314:string[])  [unwired: 2 in, 2 out]
              n126 = Enqueue Element(queue=w333, element="desired wafer to current wafer", error in (no error)=w328) -> (queue out=w332:refnum<queue>, error out=w329:errorcluster)  [unwired: 1 in, 1 out]
              n127 = Enqueue Element(queue=w332, element="update wafer", error in (no error)=w329) -> (queue out=w331:refnum<queue>, error out=w330:errorcluster)  [unwired: 1 in, 1 out]
              n128 = for {
                tunnel: [w353] -> w324
                tunnel: [w352] -> w317
                tunnel: w331 -> [w351]
                tunnel: w330 -> [w350]
                tunnel: w314 -> [_] mode=indexing
                # "Executes Lot Test\n1) First Wafer Loaded? - If the first wafer in the lot is already on the chuck, the user selects this and the loading wafer steps are skipped for the first iteration of the the for loop.\n2) Load wafer - loads the wafer from the cassette to the chuck\n3)wait - waits ten seconds  - if the profile command comes while the cwafer is still being loaded the probe station gives an error\n4) Profile z and autoalign - completes the rest of the loading procedure\n5) desired wafer to current wafer - changes wafer name to the next on on the \"Wafer List\"\n6) update wafer - update wafer info\n7) Runs auto test (see auto test tab)"
                n129 = Enqueue Element(queue=w351, element="select temperature", error in (no error)=w350) -> (queue out=w349:refnum<queue>, error out=w348:errorcluster)  [unwired: 1 in, 1 out]
                n130 = Enqueue Element(queue=w349, element="update temperature", error in (no error)=w348) -> (queue out=w347:refnum<queue>, error out=w346:errorcluster)  [unwired: 1 in, 1 out]
                n131 = Enqueue Element(queue=w347, element="wait for temperature", error in (no error)=w346) -> (queue out=w345:refnum<queue>, error out=w344:errorcluster)  [unwired: 1 in, 1 out]
                n132 = property on="Test List" class="LstBox (strict)"() -> ("Item Names"=w359:string[])  [unwired: 2 in, 2 out]
                n133 = for {
                  shift-right: [w364] -> w354
                  shift-left: w344 -> [w369]
                  shift-right: [w365] -> w355
                  shift-left: w345 -> [w370]
                  tunnel: w359 -> [_] mode=indexing
                  n134 = Enqueue Element(queue=w370, element="skip raw?", error in (no error)=w369) -> (queue out=w368:refnum<queue>, error out=w367:errorcluster)  [unwired: 1 in, 1 out]
                  n135 = Enqueue Element(queue=w368, element="pick device", error in (no error)=w367) -> (queue out=w376:refnum<queue>, error out=w375:errorcluster)  [unwired: 1 in, 1 out]
                  n136 = case shown="False" FALSE {
                    tunnel: w376 -> [w429 w442]
                    tunnel: w375 -> [w428 w443]
                    tunnel: [w426 w442] -> w374
                    tunnel: [w425 w443] -> w373
                    frame False {
                      n137 = local read "Enable Laser"() -> (w427:bool)
                      n138 = case shown="True" w427 {
                        tunnel: [w433 w441] -> w431
                        tunnel: [w432 w440] -> w430
                        tunnel: w429 -> [w433 w438]
                        tunnel: w428 -> [w432 w436]
                        frame False {
                        }
                        frame True {
                          n139 = Enqueue Element(queue=w438, element="Zero Laser", error in (no error)=w436) -> (queue out=w437:refnum<queue>, error out=w435:errorcluster)  [unwired: 1 in, 1 out]
                          n140 = Enqueue Element(queue=w437, element="Update Laser", error in (no error)=w435) -> (queue out=w441:refnum<queue>, error out=w440:errorcluster)  [unwired: 1 in, 1 out]
                        }
                      }
                      n141 = Enqueue Element(queue=w431, element="start raw", error in (no error)=w430) -> (queue out=w422:refnum<queue>, error out=w421:errorcluster)  [unwired: 1 in, 1 out]
                      n142 = Enqueue Element(queue=w422, element="select", error in (no error)=w421) -> (queue out=w426:refnum<queue>, error out=w425:errorcluster)  [unwired: 1 in, 1 out]
                    }
                    frame True {
                    }
                  }
                  n143 = local read "Enable Laser"() -> (w371:bool)
                  n144 = case shown="True" w371 {
                    tunnel: [w383 w399] -> w362
                    tunnel: [w382 w398] -> w363
                    tunnel: w374 -> [w381 w397]
                    tunnel: w373 -> [w380 w396]
                    frame False {
                      n145 = local read "Only Raw Test"() -> (w378:bool)
                      n146 = Not(x=w378) -> (.not. x?=w379:bool)
                      n147 = case shown="False" w379 {
                        tunnel: [w385 w393] -> w383
                        tunnel: [w384 w392] -> w382
                        tunnel: w381 -> [w385 w391]
                        tunnel: w380 -> [w384 w389]
                        frame False {
                        }
                        frame True {
                          n148 = Enqueue Element(queue=w391, element="find best devices mask", error in (no error)=w389) -> (queue out=w390:refnum<queue>, error out=w388:errorcluster)  [unwired: 1 in, 1 out]
                          n149 = Enqueue Element(queue=w390, element="start fine", error in (no error)=w388) -> (queue out=w393:refnum<queue>, error out=w392:errorcluster)  [unwired: 1 in, 1 out]
                        }
                      }
                    }
                    frame True {
                      n150 = local read "Only Raw Test"() -> (w394:bool)
                      n151 = Not(x=w394) -> (.not. x?=w395:bool)
                      n152 = case shown="True" w395 {
                        tunnel: [w401 w406] -> w399
                        tunnel: [w400 w405] -> w398
                        tunnel: w397 -> [w401 w404]
                        tunnel: w396 -> [w400 w403]
                        frame False {
                        }
                        frame True {
                          n153 = property on="Laser List" class="LstBox (strict)"() -> ("Item Names"=w402:string[])  [unwired: 2 in, 2 out]
                          n154 = for {
                            tunnel: [w420] -> w406
                            tunnel: [w419] -> w405
                            tunnel: w404 -> [w415]
                            tunnel: w403 -> [w418]
                            tunnel: w402 -> [_] mode=indexing
                            n155 = Enqueue Element(queue=w415, element="pick laser", error in (no error)=w418) -> (queue out=w414:refnum<queue>, error out=w416:errorcluster)  [unwired: 1 in, 1 out]
                            n156 = Enqueue Element(queue=w414, element="Update Laser", error in (no error)=w416) -> (queue out=w409:refnum<queue>, error out=w412:errorcluster)  [unwired: 1 in, 1 out]
                            n157 = Enqueue Element(queue=w409, element="find best devices mask", error in (no error)=w412) -> (queue out=w410:refnum<queue>, error out=w411:errorcluster)  [unwired: 1 in, 1 out]
                            n158 = Enqueue Element(queue=w410, element="start fine", error in (no error)=w411) -> (queue out=w420:refnum<queue>, error out=w419:errorcluster)  [unwired: 1 in, 1 out]
                          }
                        }
                      }
                    }
                  }
                  n159 = Enqueue Element(queue=w362, element="reset skip", error in (no error)=w363) -> (queue out=w365:refnum<queue>, error out=w364:errorcluster)  [unwired: 1 in, 1 out]
                }
                n160 = Enqueue Element(queue=w355, element="Zero Laser", error in (no error)=w354) -> (queue out=w358:refnum<queue>, error out=w357:errorcluster)  [unwired: 1 in, 1 out]
                n161 = Enqueue Element(queue=w358, element="update laser", error in (no error)=w357) -> (queue out=w353:refnum<queue>, error out=w352:errorcluster)  [unwired: 1 in, 1 out]
              }
              n162 = Enqueue Element(queue=w324, element="temp to 25", error in (no error)=w317) -> (queue out=w323:refnum<queue>, error out=w318:errorcluster)  [unwired: 1 in, 1 out]
              n163 = Enqueue Element(queue=w323, element="update temperature", error in (no error)=w318) -> (queue out=w322:refnum<queue>, error out=w319:errorcluster)  [unwired: 1 in, 1 out]
              n164 = Enqueue Element(queue=w322, element="update measurement log", error in (no error)=w319) -> (queue out=w321:refnum<queue>, error out=w320:errorcluster)  [unwired: 1 in, 1 out]
            }
          }
          event "update temp": Value Change {
            # "Gives the VISA commands to update chuck temperature"
            n165 = event-data() -> ()  [unwired: 1 in, 5 out]
            n166 = Enqueue Element(queue=w464, element="update temperature", error in (no error)=w463) -> (queue out=w462:refnum<queue>, error out=w461:errorcluster)  [unwired: 1 in, 1 out]
          }
          event "Add to Temp": Value Change {
            # "adds value from desired temperature to temperature list"
            n167 = event-data() -> ()  [unwired: 1 in, 5 out]
            n168 = Enqueue Element(queue=w469, element="add to temp list", error in (no error)=w468) -> (queue out=w467:refnum<queue>, error out=w466:errorcluster)  [unwired: 1 in, 1 out]
          }
          event "Remove from Temp": Value Change {
            # "removes highlighted value from temperature list"
            n169 = event-data() -> ()  [unwired: 1 in, 5 out]
            n170 = Enqueue Element(queue=w474, element="remove from temp list", error in (no error)=w473) -> (queue out=w472:refnum<queue>, error out=w471:errorcluster)  [unwired: 1 in, 1 out]
          }
          event "Clear temp list": Value Change {
            # "removes all values from temperature list"
            n171 = event-data() -> ()  [unwired: 1 in, 5 out]
            n172 = Enqueue Element(queue=w479, element="clear temp list", error in (no error)=w478) -> (queue out=w477:refnum<queue>, error out=w476:errorcluster)  [unwired: 1 in, 1 out]
          }
          event "load file for temp series": Value Change {
            # "works the same as loading manual mask file, but this is just in the temperature series tab"
            n173 = event-data() -> ()  [unwired: 1 in, 5 out]
            n174 = Enqueue Element(queue=w483, element="load file for temp", error in (no error)=w482) -> (queue out=w481:refnum<queue>, error out=w480:errorcluster)  [unwired: 1 in, 1 out]
          }
          event "move prober 2": Value Change {
            # "does the same as \"moveto\" from a different button"
            n175 = event-data() -> ()  [unwired: 1 in, 5 out]
            n176 = Enqueue Element(queue=w488, element="moveto", error in (no error)=w489) -> (queue out=w486:refnum<queue>, error out=w487:errorcluster)  [unwired: 1 in, 1 out]
          }
          event "Desired Device": Value Change {
            # "Does the same as \"Die number changed\" but from the temperature series tab"
            n177 = event-data() -> ()  [unwired: 1 in, 5 out]
            n178 = Enqueue Element(queue=w494, element="desired device change", error in (no error)=w493) -> (queue out=w492:refnum<queue>, error out=w491:errorcluster)  [unwired: 1 in, 1 out]
          }
          event "Start temp": Value Change {
            # "Begins Temperature Series\n1) Selects Temperature - updates current temprature from temp list\n2) Update temperature - writes current temperature to Temptronic TEC\n3) Wait fr temperature - waits until the temperature has settled on the correct value\n4) begin temperature series - runs a few fine tests with different tempreatures (in progress)"
            n179 = event-data() -> ()  [unwired: 1 in, 5 out]
            n180 = local read "Comments Temp"() -> (w495:string)
            n181 = local write "Test Type"("Temperature Test" ("Test Type")) -> ()
            n182 = local write "Comments"(w495) -> ()
            n183 = Enqueue Element(queue=w503, element="begin temperature series", error in (no error)=w502) -> (queue out=w500:refnum<queue>, error out=w499:errorcluster)  [unwired: 1 in, 1 out]
            n184 = Enqueue Element(queue=w500, element="update measurement log", error in (no error)=w499) -> (queue out=w498:refnum<queue>, error out=w497:errorcluster)  [unwired: 1 in, 1 out]
          }
          event "Refresh Device": Value Change {
            # "This is supposed to populate the device mane list from the given mask file. As of 8/5/18 it isn't working properly"
            n185 = event-data() -> ()  [unwired: 1 in, 5 out]
            n186 = Enqueue Element(queue=w509, element="refresh device names", error in (no error)=w508) -> (queue out=w507:refnum<queue>, error out=w506:errorcluster)  [unwired: 1 in, 1 out]
          }
          event "Add to list": Value Change {
            # "Adds device name value to test list"
            n187 = event-data() -> ()  [unwired: 1 in, 5 out]
            n188 = Enqueue Element(queue=w514, element="add to list", error in (no error)=w513) -> (queue out=w512:refnum<queue>, error out=w511:errorcluster)  [unwired: 1 in, 1 out]
          }
          event "Remove from List": Value Change {
            # "removes highlighted walue from test list"
            n189 = event-data() -> ()  [unwired: 1 in, 5 out]
            n190 = Enqueue Element(queue=w519, element="remove from list", error in (no error)=w517) -> (queue out=w518:refnum<queue>, error out=w516:errorcluster)  [unwired: 1 in, 1 out]
          }
          event "Clear List": Value Change {
            # "removes all entries from test list"
            n191 = event-data() -> ()  [unwired: 1 in, 5 out]
            n192 = Enqueue Element(queue=w524, element="clear list", error in (no error)=w523) -> (queue out=w522:refnum<queue>, error out=w521:errorcluster)  [unwired: 1 in, 1 out]
          }
          event "Load Wafer": Value Change {
            # "Loads wafer and performs profilng and auto alignment procedures"
            n193 = event-data() -> ()  [unwired: 1 in, 5 out]
            n194 = Enqueue Element(queue=w538, element="load wafer", error in (no error)=w537) -> (queue out=w529:refnum<queue>, error out=w528:errorcluster)  [unwired: 1 in, 1 out]
            n195 = Enqueue Element(queue=w529, element="wait", error in (no error)=w528) -> (queue out=w527:refnum<queue>, error out=w526:errorcluster)  [unwired: 1 in, 1 out]
            n196 = Enqueue Element(queue=w527, element="profile z", error in (no error)=w526) -> (queue out=w534:refnum<queue>, error out=w532:errorcluster)  [unwired: 1 in, 1 out]
            n197 = Enqueue Element(queue=w534, element="auto align", error in (no error)=w532) -> (queue out=w533:refnum<queue>, error out=w531:errorcluster)  [unwired: 1 in, 1 out]
          }
          event "Profile Z": Value Change {
            # "Performs just the z profile"
            n198 = event-data() -> ()  [unwired: 1 in, 5 out]
            n199 = Enqueue Element(queue=w543, element="profile z", error in (no error)=w541) -> (queue out=w542:refnum<queue>, error out=w540:errorcluster)  [unwired: 1 in, 1 out]
          }
          event "Add to Laser": Value Change {
            # "adds desired laser value to laser list"
            n200 = event-data() -> ()  [unwired: 1 in, 5 out]
            n201 = Enqueue Element(queue=w547, element="add to laser list", error in (no error)=w546) -> (queue out=w544:refnum<queue>, error out=w545:errorcluster)  [unwired: 1 in, 1 out]
          }
          event "Remove from Laser List": Value Change {
            # "removes highlighted value from laser list"
            n202 = event-data() -> ()  [unwired: 1 in, 5 out]
            n203 = Enqueue Element(queue=w552, element="remove from laser list", error in (no error)=w551) -> (queue out=w549:refnum<queue>, error out=w550:errorcluster)  [unwired: 1 in, 1 out]
          }
          event "Clear Laser List": Value Change {
            # "removes all entries from laser list"
            n204 = event-data() -> ()  [unwired: 1 in, 5 out]
            n205 = Enqueue Element(queue=w557, element="clear laser list", error in (no error)=w555) -> (queue out=w556:refnum<queue>, error out=w554:errorcluster)  [unwired: 1 in, 1 out]
          }
          event "Add to wafer list": Value Change {
            # "Adds desired value to wafer list"
            n206 = event-data() -> ()  [unwired: 1 in, 5 out]
            n207 = Enqueue Element(queue=w563, element="add to wafer list", error in (no error)=w562) -> (queue out=w560:refnum<queue>, error out=w559:errorcluster)  [unwired: 1 in, 1 out]
          }
          event "Remove from wafer list": Value Change {
            # "removes highlighted value from wafer list"
            n208 = event-data() -> ()  [unwired: 1 in, 5 out]
            n209 = Enqueue Element(queue=w567, element="remove from wafer list", error in (no error)=w566) -> (queue out=w565:refnum<queue>, error out=w564:errorcluster)  [unwired: 1 in, 1 out]
          }
          event "Clear wafer list": Value Change {
            # "removes all values from wafer list"
            n210 = event-data() -> ()  [unwired: 1 in, 5 out]
            n211 = Enqueue Element(queue=w572, element="clear wafer list", error in (no error)=w571) -> (queue out=w570:refnum<queue>, error out=w569:errorcluster)  [unwired: 1 in, 1 out]
          }
          event "Update viewer": Value Change {
            # "Updates the measurement log viewer from the csv file in case of manual changes to the log"
            n212 = event-data() -> ()  [unwired: 1 in, 5 out]
            n213 = Enqueue Element(queue=w578, element="update viewer", error in (no error)=w577) -> (queue out=w576:refnum<queue>, error out=w575:errorcluster)  [unwired: 1 in, 1 out]
          }
          event "Save Comment": Value Change {
            # "Saves the comment to the highlighted entry in the measurement log, and updates the viewer to match the csv file. I still havent gotten the measurement log to close automatically however"
            n214 = event-data() -> ()  [unwired: 1 in, 5 out]
            n215 = Enqueue Element(queue=w586, element="save comment", error in (no error)=w585) -> (queue out=w583:refnum<queue>, error out=w581:errorcluster)  [unwired: 1 in, 1 out]
            n216 = Enqueue Element(queue=w583, element="update viewer", error in (no error)=w581) -> (queue out=w582:refnum<queue>, error out=w580:errorcluster)  [unwired: 1 in, 1 out]
          }
          event "Explore Data": Value Change {
            n217 = event-data() -> ()  [unwired: 1 in, 5 out]
            n218 = Enqueue Element(queue=w590, element="explore data", error in (no error)=w589) -> (queue out=w588:refnum<queue>, error out=w587:errorcluster)  [unwired: 1 in, 1 out]
          }
        }
      }
      n219 = while {
        shift-right: [w599] -> _
        shift-left: w42 -> [w596]
        shift-right: [w598] -> _
        shift-left: w41 -> [w595]
        stop <- w601 stop-if-true
        n220 = Dequeue Element(queue=w596, error in (no error)=w595) -> (queue out=w594:refnum<queue>, element=w600:string, error out=w597:errorcluster)  [unwired: 1 in, 1 out]
        n221 = local read "Laser Current (mA)"() -> (w593:dbl)
        n222 = Greater Than 0?(x=w593) -> (x > 0?=w592:bool)
        n223 = case shown="\"begin temperature series\"" w600 {
          tunnel: [FALSE TRUE FALSE FALSE FALSE FALSE FALSE FALSE FALSE FALSE FALSE _ FALSE _ FALSE FALSE FALSE FALSE FALSE FALSE _ FALSE FALSE FALSE FALSE FALSE FALSE FALSE FALSE FALSE FALSE FALSE FALSE FALSE FALSE _ _ _ FALSE FALSE FALSE _ _ _ _ _ _ _ _ _ _ _ _ _ _ _ _ _] -> w601
          tunnel: w597 -> [w603 w606 w610 w808 w852 w863 w874 w905 w929 w940 w972 w1174 w1180 w1190 w1202 w1209 w1223 w1260 w1304 w1341 w1573 w1576 w1612 w1621 w1632 w1638 w1689 w1702 w1714 w1737 w1760 w1763 w1769 w1775 w1783 w1793 w1798 w1801 w1806 w1822 w1841 w1856 w1866 w1868 w1876 w1881 w1886 w1889 w1892 w1911 w1924 w1948 w1952 w1983 w2260 w2265 w2268 w2270]
          tunnel: [w603 w606 w611 w808 w853 w860 w871 w908 w930 w943 w971 w1174 w1185 w1190 w1202 w1208 w1225 w1260 w1306 w1343 w1573 w1576 w1612 w1623 w1634 w1638 w1689 w1698 w1717 w1737 w1760 w1763 w1769 w1777 w1786 w1793 w1798 w1801 w1805 w1822 w1841 w1856 w1866 w1868 w1876 w1881 w1886 w1889 w1892 w1911 w1924 w1948 w1951 w1983 w2260 w2265 w2268 w2270] -> w598
          tunnel: w594 -> [w602 w605 w613 w809 w855 w862 w873 w906 w932 w945 w969 w1175 w1187 w1191 w1203 w1207 w1224 w1261 w1305 w1340 w1574 w1577 w1613 w1622 w1633 w1639 w1690 w1703 w1716 w1738 w1761 w1764 w1770 w1776 w1785 w1794 w1799 w1802 w1808 w1823 w1842 w1857 w1867 w1869 w1877 w1882 w1887 w1890 w1893 w1912 w1925 w1949 w1954 w1984 w2261 w2266 w2269 w2271]
          tunnel: [w602 w605 w612 w809 w854 w861 w872 w907 w931 w944 w970 w1175 w1186 w1191 w1203 w1206 w1226 w1261 w1307 w1342 w1574 w1577 w1613 w1624 w1635 w1639 w1690 w1704 w1718 w1738 w1761 w1764 w1770 w1778 w1787 w1794 w1799 w1802 w1807 w1823 w1842 w1857 w1867 w1869 w1877 w1882 w1887 w1890 w1893 w1912 w1925 w1949 w1953 w1984 w2261 w2266 w2269 w2271] -> w599
          tunnel: w592 -> [_ _ _ _ _ _ _ _ _ _ _ _ _ _ _ _ _ _ _ w1344 _ _ _ _ _ _ _ _ _ _ _ _ _ _ _ _ _ _ _ _ _ _ _ _ _ _ _ _ _ _ _ _ _ _ _ _ _ _]
          frame "False", Default {
          }
          frame "stop" {
            # "Ends the for loop that contains the event structure, effectively ending the program"
          }
          frame "start raw" {
            # "Raw Test:\n(If Raw Test Skipped is TRUE, the entire raw test is not run. This only happens as part of the auto or lot tests)\n1) Loads mask file and updates info\n2) Finds/Creates directory for new Raw test file and creates file\n3) Runs raw test and updates graph after every measurement is taken\n4) Resets the prober to 0 0"
            n224 = local read "Raw Test Skipped"() -> (w609:bool)
            n225 = Not(x=w609) -> (.not. x?=w608:bool)
            n226 = Enqueue Element At Opposite End(queue=w613, element="idle", error in (no error)=w610) -> (queue out=w612:refnum<queue>, error out=w611:errorcluster)  [unwired: 1 in, 1 out]
            n227 = case shown="True" w608 {
              frame False {
              }
              frame True {
                n228 = flat-sequence {
                  tunnel: [w628] -> w618
                  tunnel: w618 -> [w664]
                  tunnel: [w664] -> w617
                  tunnel: [w657] -> w616
                  tunnel: w617 -> [w666]
                  tunnel: w616 -> [w665]
                  frame #0 {
                    n229 = local read "Wafer Name"() -> (w626:string)
                    n230 = local read "RawTest ID"() -> (w631:u32)
                    n231 = local write "Tab Control"(T16."Raw Test" ("Tab Control")) -> ()
                    n232 = Increment(x=w631) -> (x+1=w630:u32)
                    n233 = local read "Scribe"() -> (w625:string)
                    n234 = local read "Mask"() -> (w624:string)
                    n235 = call "Device Files v1.vi"("Rows"=1200, "Mask file path"="Mask File Raw") -> ("size(s)"=w628:i32, "Array of Cell Clusters"=→"Array of Cell Data Clusters":T5)  [unwired: 6 in, 2 out]
                    "Total Device" <- w628
                    n236 = local read "Lot"() -> (w623:string)
                    n237 = local write "Status"("Prepare raw test" ("Status")) -> ()
                    n238 = local write "RawTest ID"(w630) -> ()
                    n239 = Bundle By Name(cluster="Wafer Info 2", "Wafer Name"=w626, "Scribe"=w625, "Mask"=w624, "Lot"=w623) -> (w627:T9)
                    n240 = local write "Wafer Info"(w627) -> ()
                    n241 = Initialize Array(nan ("element"), w628) -> (w621:dbl[])
                    n242 = local write "I meas"(w621) -> ()
                    n243 = local write "V meas"(w621) -> ()
                    n244 = Bundle(w621, w621) -> (→"Selected Data":cluster{dbl[], dbl[]})  [unwired: 1 in]
                    "Progress" <- u8 0 ("Progress")
                  }
                  frame #1 {
                    n245 = local read "RawData Save Path"() -> (w639:path)
                    n246 = local read "Wafer Name"() -> (w643:string)
                    n247 = local read "J set A/cm2"() -> (w651:dbl)
                    n248 = local read "RawTest ID"() -> (w647:u32)
                    n249 = local read "Operator"() -> (w646:string)
                    n250 = local read "Laser Current (mA)"() -> (w648:dbl)
                    n251 = local read "Lot"() -> (w645:string)
                    n252 = local read "V compliance"() -> (w649:dbl)
                    n253 = local read "Array of Cell Data Clusters"() -> (w663:T12)
                    n254 = local read "I compliance"() -> (w652:dbl)
                    n255 = Build Path(base path=w639, name or relative path=w645) -> (appended path=w644:path)
                    n256 = call "CreateDirectory.vi"("Path to be created"=w644) -> ()  [unwired: 10 in, 1 out]
                    n257 = Build Path(base path=w644, name or relative path=w643) -> (appended path=w642:path)
                    n258 = Index Array(array=w663, index=0) -> (element=w661:T17)
                    n259 = call "CreateDirectory.vi"("Path to be created"=w642) -> ()  [unwired: 10 in, 1 out]
                    n260 = Unbundle By Name(w661) -> ("Cell Name"=w660:string)
                    n261 = Build Path(base path=w642, name or relative path="Raw Data") -> (appended path=w640:path)
                    "new raw data save path" <- w640
                    n262 = call "CreateDirectory.vi"("Path to be created"=w640) -> ("Output"=w637:path)  [unwired: 10 in]
                    n263 = call "get RawTest filename.vi"("Device Name"=w660, "Wafer Name"=w643) -> ("current time"=w654:timestamp, "FileName"=w659:string)  [unwired: 8 in]
                    n264 = local write "Test FileName"(w659) -> ()
                    n265 = local read "V set"() -> (w653:dbl)
                    n266 = local read "I set"() -> (w650:dbl)
                    n267 = Build Path(base path=w637, name or relative path=w659) -> (appended path=w638:path)
                    "Raw Test Filename" <- w638
                    n268 = Bundle By Name(cluster="Session Info 2", "V set"=w653, "I compliance"=w652, "J set"=w651, "I set"=w650, "V compliance"=w649, "Laser Power (mW)"=w648, "TestID"=w647, "Session Time"=w654, "Operator"=w646) -> (w655:T7)
                    n269 = call "writeFile RawTestHead.vi"("Name Array"="Name Array", "Path"=w638) -> ("Path out"=w657:path)  [unwired: 9 in]
                    "RawData file" <- w657
                    n270 = local write "Session Info"(w655) -> ()
                  }
                  frame #2 {
                    n271 = for {
                      N: w666 -> [w679]
                      tunnel: w665 -> [w667]
                      i -> [w668]
                      n272 = flat-sequence {
                        tunnel: [w713] -> w688
                        tunnel: [w712] -> w687
                        tunnel: w668 -> [w706]
                        tunnel: [w708] -> w683
                        tunnel: [w707] -> w682
                        tunnel: [w690] -> w681
                        tunnel: [w689] -> w680
                        tunnel: w688 -> [w714]
                        tunnel: w687 -> [w722]
                        tunnel: [w721] -> w686
                        tunnel: [w720] -> w685
                        tunnel: w683 -> [w718]
                        tunnel: w682 -> [w717]
                        tunnel: w681 -> [w716]
                        tunnel: w680 -> [w715]
                        tunnel: w686 -> [w725]
                        tunnel: w685 -> [w724]
                        tunnel: [w727] -> w684
                        tunnel: w684 -> [w751]
                        tunnel: [w751] -> w670
                        tunnel: [w752] -> w669
                        tunnel: w670 -> [w784]
                        tunnel: w669 -> [w783]
                        tunnel: w668 -> [w790]
                        tunnel: w667 -> [w781]
                        frame #0 {
                          n273 = Increment(x=w706) -> (x+1=→"Current Device":i32)
                          n274 = local read "Prober GPIB"() -> (w704:string)
                          n275 = local read "J set A/cm2"() -> (w698:dbl)
                          n276 = local read "current y"() -> (w709:i32)
                          n277 = local read "current x"() -> (w711:i32)
                          n278 = local read "Laser Current (mA)"() -> (w702:dbl)
                          n279 = local read "Device Name"() -> (w693:string)
                          n280 = local read "Array of Cell Data Clusters"() -> (w710:T12)
                          n281 = call "EG2001 Move Z Down.vi"("GPIB Address"=w704) -> ("Error Out"=w712:errorcluster, "GPIB Address Out"=w713:string)  [unwired: 9 in]
                          n282 = Index Array(array=w710, index=w706) -> (element=w703:T17)
                          n283 = Unbundle By Name(w703) -> ("X-coord"=w690:dbl, "Y-coord"=w689:dbl, "Area"=w691:dbl, "Meas Area"=w692:dbl, "Cell Name"=w696:string)
                          n284 = call "get Area.vi"("Laser"=w702, "Cell Data Cluster"=w703) -> ("Area"=w700:dbl)  [unwired: 9 in]
                          n285 = local write "ActiveArea_um2"(w691) -> ()
                          n286 = local write "Device Name"(w696) -> ()
                          n287 = local write "MesaArea_um2"(w692) -> ()
                          n288 = Divide(x=w700, y=100000000.0) -> (x/y=w699:dbl)
                          n289 = Bundle By Name(cluster="Die Info 2", "Device Name"=w693, "ActiveArea_um2"=w691, "MesaArea_um2"=w692, "x"=w690, "y"=w689) -> (w694:T8)
                          n290 = Multiply(x=w698, y=w699) -> (x*y=w697:dbl)
                          n291 = local write "Die Info"(w694) -> ()
                          n292 = local write "I set"(w697) -> ()
                          n293 = Subtract(x=w689, y=w709) -> (x-y=w707:dbl)
                          n294 = Subtract(x=w690, y=w711) -> (x-y=w708:dbl)
                        }
                        frame #1 {
                          n295 = local write "current y"(w715) -> ()
                          n296 = local write "current x"(w716) -> ()
                          n297 = call "EG2001 Move Machine Step X-Y.vi"("Flip X Coordinates?"=FALSE, "Y"=w717, "Steps/Microns"=enum32{"Steps", "Microns"}."Microns", "X"=w718, "error in (no error)"=w722, "GPIB Address"=w714) -> ("Error Out"=w720:errorcluster, "GPIB Address Out"=w721:string)  [unwired: 4 in]
                        }
                        frame #2 {
                          n298 = call "EG2001 Move Z Up.vi"("error in (no error)"=w724, "GPIB Address"=w725) -> ()  [unwired: 10 out]
                        }
                        frame #3 {
                          n299 = local read "Keysight"() -> (w726:bool)
                          n300 = case shown="False" w726 {
                            tunnel: [w728 w749] -> w727
                            frame False {
                              n301 = local read "Channel Keysight"() -> (w738:dbl)
                              n302 = local read "Id delay ms"() -> (w734:dbl)
                              n303 = local read "Repeat Id"() -> (w735:u32)
                              n304 = local read "Imeas Settings"() -> (w732:T11)
                              n305 = local read "I compliance"() -> (w736:dbl)
                              n306 = local read "4-wire"() -> (w731:bool)
                              n307 = local read "NPLC"() -> (w737:dbl)
                              n308 = local read "V set"() -> (w733:dbl)
                              n309 = Bundle By Name(cluster=w732, "Channel"=w738, "Vset"=w733, "NPLC"=w737, "I compliance"=w736, "Repeat time"=w735, "Delay ms"=w734, "4-wire"=w731) -> (w730:T11)
                              n310 = local read "Keysight SMU"() -> (w729:refnum<visa-resource-name>)
                              n311 = local write "Imeas Settings"(w730) -> ()
                              n312 = call "Agilent B2900 Measure I at Vset.vi"("Imeas Settings"=w730, "VISA resource name"=w729) -> ("Avg I"=w728:dbl)  [unwired: 9 in]
                            }
                            frame True {
                              n313 = local read "Id delay ms"() -> (w743:dbl)
                              n314 = local read "Repeat Id"() -> (w744:u32)
                              n315 = local read "Imeas Settings"() -> (w741:T11)
                              n316 = local read "Channel"() -> (w747:enum32{"Channel A", "Channel B"})
                              n317 = local read "I compliance"() -> (w745:dbl)
                              n318 = local read "4-wire"() -> (w740:bool)
                              n319 = local read "NPLC"() -> (w746:dbl)
                              n320 = local read "V set"() -> (w742:dbl)
                              n321 = Bundle By Name(cluster=w741, "Channel"=w747, "Vset"=w742, "NPLC"=w746, "I compliance"=w745, "Repeat time"=w744, "Delay ms"=w743, "4-wire"=w740) -> (w739:T11)
                              n322 = local read "Keithley SMU"() -> (w748:refnum<visa-resource-name>)
                              n323 = local write "Imeas Settings"(w739) -> ()
                              n324 = call "K2602 setVmeasI.vi"("Settings"=w739, "SMU"=w748) -> ("Iavg"=w749:dbl)  [unwired: 6 in, 3 out]
                            }
                          }
                        }
                        frame #4 {
                          n325 = local read "Keysight"() -> (w750:bool)
                          n326 = case shown="False" w750 {
                            tunnel: [w753 w768] -> w752
                            frame False {
                              n327 = local read "Repeat Vf"() -> (w760:u32)
                              n328 = local read "Vf delay ms"() -> (w759:dbl)
                              n329 = local read "V compliance"() -> (w761:dbl)
                              n330 = local read "Vmeas Settings"() -> (w763:T11)
                              n331 = local read "Channel"() -> (w762:enum32{"Channel A", "Channel B"})
                              n332 = local read "4-wire"() -> (w756:bool)
                              n333 = local read "NPLC"() -> (w758:dbl)
                              n334 = local read "I set"() -> (w757:dbl)
                              n335 = local read "Keysight SMU"() -> (w754:refnum<visa-resource-name>)
                              n336 = Bundle By Name(cluster=w763, "Channel"=w762, "Vset"=w757, "NPLC"=w758, "I compliance"=w761, "Repeat time"=w760, "Delay ms"=w759, "4-wire"=w756) -> (w755:T11)
                              n337 = local write "Vmeas Settings"(w755) -> ()
                              n338 = call "Agilent B2900 Measure V at Iset.vi"("Imeas Settings"=w755, "VISA resource name"=w754) -> ("Avg V"=w753:dbl)  [unwired: 9 in]
                            }
                            frame True {
                              n339 = local read "Repeat Vf"() -> (w770:u32)
                              n340 = local read "Vf delay ms"() -> (w769:dbl)
                              n341 = local read "V compliance"() -> (w771:dbl)
                              n342 = local read "Channel Keysight"() -> (w772:dbl)
                              n343 = local read "Vmeas Settings"() -> (w773:T11)
                              n344 = local read "4-wire"() -> (w765:bool)
                              n345 = local read "NPLC"() -> (w767:dbl)
                              n346 = local read "I set"() -> (w766:dbl)
                              n347 = Bundle By Name(cluster=w773, "Channel"=w772, "Vset"=w766, "NPLC"=w767, "I compliance"=w771, "Repeat time"=w770, "Delay ms"=w769, "4-wire"=w765) -> (w764:T11)
                              n348 = local write "Vmeas Settings"(w764) -> ()
                              n349 = call "K2602 setImeasV.vi"("Settings"=w764) -> ("Vavg"=w768:dbl)  [unwired: 7 in, 3 out]
                            }
                          }
                        }
                        frame #5 {
                          n350 = local read "Session Info"() -> (w777:T7)
                          n351 = local read "Wafer Info"() -> (w779:T9)
                          n352 = local read "Die Info"() -> (w778:T8)
                          n353 = local read "V meas"() -> (w791:dbl[])
                          n354 = local read "I meas"() -> (w792:dbl[])
                          n355 = local read "Selected Data"() -> (w775:cluster{dbl[], dbl[]})
                          n356 = Replace Array Subset(array=w792, new element=w784, index=w790) -> (w787:dbl[])
                          n357 = Replace Array Subset(array=w791, new element=w783, index=w790) -> (w786:dbl[])
                          n358 = Get Date/Time In Seconds() -> (seconds since 1Jan1904=w782:timestamp)
                          n359 = local write "I meas"(w787) -> ()
                          n360 = Bundle By Name(cluster="Test Results 2", "I meas"=w784, "V meas"=w783, "Time"=w782) -> (w780:T6)
                          n361 = local write "V meas"(w786) -> ()
                          n362 = call <vilib>:"Histogram.vi"("X"=w786) -> ("Histogram Graph"=→"Vforward hist":T14)  [unwired: 7 in, 3 out]
                          n363 = call "writeFile RawTestData.vi"("Test Results"=w780, "Session Info"=w777, "Die Info"=w778, "Wafer Info"=w779, "Path"=w781) -> ()  [unwired: 6 in, 1 out]
                          n364 = local write "Test Results"(w780) -> ()
                          n365 = call <vilib>:"Histogram.vi"("X"=w787) -> ("Histogram Graph"=→"Idark hist":T14)  [unwired: 7 in, 3 out]
                          n366 = Bundle("V meas"=w786, "I meas"=w787) -> (w776:cluster{"V meas":dbl[], "I meas":dbl[]})  [unwired: 1 in]
                          n367 = Build Array(w776, w775) -> (→"Spec Plot":cluster{"V meas":dbl[], "I meas":dbl[]}[])
                        }
                      }
                      n368 = Divide(x=w668, y=w679) -> (x/y=w677:dbl)
                      n369 = Increment(x=w668) -> (x+1=w671:i32)
                      n370 = Number To Decimal String(number=w671) -> (decimal integer string=w673:string)  [unwired: 1 in]
                      n371 = Multiply(x=w677, y=100.0) -> (x*y=w675:dbl)
                      n372 = To Unsigned Byte Integer(number=w675) -> (unsigned 8bit integer=w678:u8)
                      n373 = local write "Progress"(w678) -> ()
                      n374 = Concatenate Strings("Raw Test for die number:" ("string"), w673) -> (w674:string)
                      n375 = local write "Status"(w674) -> ()
                    }
                  }
                  frame #3 {
                    w797 = -1
                    n376 = local read "Prober GPIB"() -> (w804:string)
                    n377 = local read "RawTest ID"() -> (w794:u32)
                    n378 = local read "TestID file"() -> (w793:path)
                    n379 = local read "current y"() -> (w798:i32)
                    n380 = local read "current x"() -> (w799:i32)
                    n381 = Multiply(x=w797, y=w798) -> (x*y=w795:i32)
                    n382 = Multiply(x=w797, y=w799) -> (x*y=w796:i32)
                    n383 = call "writeFile TestID.vi"("TestID"=w794, "Path"=w793) -> ()  [unwired: 10 in]
                    n384 = call "EG2001 Move Z Down.vi"("GPIB Address"=w804) -> ("Error Out"=w803:errorcluster, "GPIB Address Out"=w802:string)  [unwired: 9 in]
                    n385 = call "EG2001 Move Machine Step X-Y.vi"("Flip X Coordinates?"=FALSE, "Y"=w795, "Steps/Microns"=enum32{"Steps", "Microns"}."Microns", "X"=w796, "error in (no error)"=w803, "GPIB Address"=w802) -> ()  [unwired: 4 in, 2 out]
                  }
                  frame #4 {
                    w805 = 0
                    n386 = local write "current y"(w805) -> ()
                    n387 = local write "current x"(w805) -> ()
                  }
                }
              }
            }
          }
          frame "find best devices mask" {
            # "If raw test is skipped - this searches through the saving structure (see guide) by lot, wafer name, and device name to find previous raw test measurements. When the file is found, it updates the fine mask file. If no file is found, a dialogue box alets the user of that"
            n388 = local read "Raw Test Skipped"() -> (w807:bool)
            n389 = case shown="True" w807 {
              frame False {
              }
              frame True {
                w823 = path "C:/Users/Flash/Desktop/Data/Detector test data" ("path")
                n390 = List Folder(path=w823) -> (folder names=w822:string[])  [unwired: 3 in, 3 out]
                n391 = for {
                  tunnel: w822 -> [w832] mode=indexing
                  tunnel: [w831] -> w824
                  tunnel: [w830] -> w814
                  stop <- w830 stop-if-true
                  n392 = local read "Lot"() -> (w831:string)
                  n393 = Equal?(x=w832, y=w831) -> (x = y?=w830:bool)
                }
                n394 = Build Path(base path=w823, name or relative path=w824) -> (appended path=w819:path)
                n395 = List Folder(path=w819) -> (folder names=w821:string[])  [unwired: 3 in, 3 out]
                n396 = for {
                  tunnel: w821 -> [w829] mode=indexing
                  tunnel: [w828] -> w820
                  tunnel: [w827] -> w816
                  stop <- w827 stop-if-true
                  n397 = local read "Wafer Name"() -> (w828:string)
                  n398 = Equal?(x=w829, y=w828) -> (x = y?=w827:bool)
                }
                n399 = Build Path(base path=w819, name or relative path=w820) -> (appended path=w812:path)
                n400 = Build Path(base path=w812, name or relative path="Raw Data") -> (appended path=w811:path)
                n401 = List Folder(path=w811) -> (filenames=w818:string[])  [unwired: 3 in, 3 out]
                n402 = for {
                  tunnel: w818 -> [w843] mode=indexing
                  tunnel: [w843] -> w825
                  tunnel: [w836] -> w817
                  stop <- w836 stop-if-true
                  w842 = "" ("y")
                  n403 = local read "Device Name"() -> (w835:string)
                  n404 = local read "Wafer Name"() -> (w846:string)
                  n405 = Concatenate Strings(w835, "_" ("string")) -> (w833:string)
                  n406 = Match Pattern(string=w843, regular expression=w833) -> (after substring=w847:string)  [unwired: 1 in, 3 out]
                  n407 = Match Pattern(string=w843, regular expression=w846) -> (after substring=w845:string)  [unwired: 1 in, 3 out]
                  n408 = Not Equal?(x=w842, y=w845) -> (x != y?=w839:bool)
                  n409 = Not Equal?(x=w847, y=w842) -> (x != y?=w848:bool)
                  n410 = And(x=w848, y=w839) -> (x .and. y?=w837:bool)
                  n411 = Match Pattern(string=w843, regular expression="mask") -> (after substring=w841:string)  [unwired: 1 in, 3 out]
                  n412 = Not Equal?(x=w842, y=w841) -> (x != y?=w840:bool)
                  n413 = And(x=w839, y=w840) -> (x .and. y?=w838:bool)
                  n414 = And(x=w837, y=w838) -> (x .and. y?=w836:bool)
                }
                n415 = Build Path(base path=w811, name or relative path=w825) -> (appended path=w826:path)
                n416 = Or(x=w817, y=w816) -> (x .or. y?=w815:bool)
                n417 = local write "Mask File Fine"(w826) -> ()
                n418 = Or(x=w815, y=w814) -> (x .or. y?=w813:bool)
                n419 = case shown="False" w813 {
                  frame False {
                    n420 = One Button Dialog(message="There is no file from which to run the fine test") -> ()  [unwired: 1 in, 1 out]
                    n421 = local write "no file"(TRUE ("no file")) -> ()
                  }
                  frame True {
                  }
                }
              }
            }
          }
          frame "reset xy" {
            # "Pretty Obvious"
            n422 = local read "Prober GPIB"() -> (w851:string)
            n423 = Enqueue Element At Opposite End(queue=w855, element="idle", error in (no error)=w852) -> (queue out=w854:refnum<queue>, error out=w853:errorcluster)  [unwired: 1 in, 1 out]
            n424 = call "EG2001 Move First.vi"("GPIB Address"=w851) -> ()  [unwired: 9 in, 2 out]
            "current x" <- u32 0 ("current x")
            "current y" <- u32 0 ("current y")
          }
          frame "reset to 1st die" {
            # "Moves prober to first die"
            n425 = Enqueue Element At Opposite End(queue=w862, element="idle", error in (no error)=w863) -> (queue out=w861:refnum<queue>, error out=w860:errorcluster)  [unwired: 1 in, 1 out]
            n426 = local read "Array of Cell Data Clusters"() -> (w869:T12)
            n427 = Index Array(array=w869, index=0) -> (element=w867:T17)
            n428 = Unbundle By Name(w867) -> ("X-coord"=w866:dbl, "Y-coord"=w865:dbl)
            n429 = local write "current x"(w866) -> ()
            n430 = local write "current y"(w865) -> ()
          }
          frame "load file manual" {
            # "Update informaiton from mask file to relevant variables"
            n431 = Enqueue Element At Opposite End(queue=w873, element="idle", error in (no error)=w874) -> (queue out=w872:refnum<queue>, error out=w871:errorcluster)  [unwired: 1 in, 1 out]
            n432 = flat-sequence {
              tunnel: [w881] -> w876
              tunnel: w876 -> [w885]
              frame #0 {
                n433 = local write "Status"("Loading mask file" ("Status")) -> ()
                n434 = call "Device Files v1.vi"("Rows"=1200, "Mask file path"="Mask File Manual") -> ("Mask Name"=w882:string, "size(s)"=w881:i32, "Array of Cell Clusters"=w878:T5)  [unwired: 6 in, 1 out]
                n435 = local write "Mask"(w882) -> ()
                n436 = local write "Array of Cell Data Clusters"(w878) -> ()
              }
              frame #1 {
                n437 = for {
                  N: w885 -> [_]
                  tunnel: [w886] -> w884 mode=indexing
                  i -> [w887]
                  n438 = Number To Decimal String(number=w887) -> (decimal integer string=w886:string)  [unwired: 1 in]
                }
                n439 = property on="Die Number" class="Ring (strict)"("Strings []"=w884) -> ()  [unwired: 2 in, 2 out]
              }
              frame #2 {
                n440 = local read "Die Number"() -> (w894:u16)
                n441 = local read "Array of Cell Data Clusters"() -> (w895:T12)
                n442 = Index Array(array=w895, index=w894) -> (element=w893:T17)
                n443 = Unbundle By Name(w893) -> ("Cell Name"=w888:string, "X-coord"=w891:dbl, "Y-coord"=w892:dbl, "Area"=w890:dbl, "Meas Area"=w889:dbl)
                n444 = local write "Device Name"(w888) -> ()
                n445 = local write "x target"(w891) -> ()
                n446 = local write "y target"(w892) -> ()
                n447 = local write "ActiveArea_um2"(w890) -> ()
                n448 = local write "MesaArea_um2"(w889) -> ()
              }
              frame #3 {
                n449 = local read "J set A/cm2"() -> (w901:dbl)
                n450 = local read "Laser Current (mA)"() -> (w898:dbl)
                n451 = Equal To 0?(x=w898) -> (x = 0?=w897:bool)
                n452 = case shown="False" w897 {
                  tunnel: [w903 w904] -> w896
                  frame False {
                    n453 = local read "ActiveArea_um2"() -> (w903:dbl)
                  }
                  frame True {
                    n454 = local read "MesaArea_um2"() -> (w904:dbl)
                  }
                }
                n455 = Divide(x=w896, y=100000000.0) -> (x/y=w900:dbl)
                n456 = Multiply(x=w900, y=w901) -> (x*y=w902:dbl)
                n457 = local write "I set"(w902) -> ()
              }
            }
          }
          frame "Die number picked" {
            # "Update target x and y when a new die is picked in the manual test tab"
            n458 = Enqueue Element At Opposite End(queue=w906, element="idle", error in (no error)=w905) -> (queue out=w907:refnum<queue>, error out=w908:errorcluster)  [unwired: 1 in, 1 out]
            n459 = local write "Status"("Changing Die" ("Status")) -> ()
            n460 = flat-sequence {
              frame #0 {
                n461 = local read "Die Number"() -> (w918:u16)
                n462 = local read "Array of Cell Data Clusters"() -> (w919:T12)
                n463 = Index Array(array=w919, index=w918) -> (element=w917:T17)
                n464 = Unbundle By Name(w917) -> ("Cell Name"=w914:string, "X-coord"=w916:dbl, "Y-coord"=w915:dbl, "Area"=w913:dbl, "Meas Area"=w912:dbl)
                n465 = local write "Device Name"(w914) -> ()
                n466 = local write "x target"(w916) -> ()
                n467 = local write "y target"(w915) -> ()
                n468 = local write "ActiveArea_um2"(w913) -> ()
                n469 = local write "MesaArea_um2"(w912) -> ()
              }
              frame #1 {
                n470 = local read "J set A/cm2"() -> (w925:dbl)
                n471 = local read "Laser Current (mA)"() -> (w922:dbl)
                n472 = Equal To 0?(x=w922) -> (x = 0?=w921:bool)
                n473 = case shown="True" w921 {
                  tunnel: [w927 w928] -> w920
                  frame False {
                    n474 = local read "ActiveArea_um2"() -> (w927:dbl)
                  }
                  frame True {
                    n475 = local read "MesaArea_um2"() -> (w928:dbl)
                  }
                }
                n476 = Divide(x=w920, y=100000000.0) -> (x/y=w924:dbl)
                n477 = Multiply(x=w924, y=w925) -> (x*y=w926:dbl)
                n478 = local write "I set"(w926) -> ()
              }
            }
          }
          frame "Jset change" {
            # "Updates Current setpoint for a desired current density"
            n479 = local read "J set A/cm2"() -> (w935:dbl)
            n480 = Enqueue Element At Opposite End(queue=w932, element="idle", error in (no error)=w929) -> (queue out=w931:refnum<queue>, error out=w930:errorcluster)  [unwired: 1 in, 1 out]
            n481 = local read "ActiveArea_um2"() -> (w938:dbl)
            n482 = Divide(x=w938, y=100000000.0) -> (x/y=w936:dbl)
            n483 = Multiply(x=w936, y=w935) -> (x*y=w934:dbl)
            n484 = local write "I set"(w934) -> ()
          }
          frame "moveto" {
            # "Moves from current xy to target xy, and then changes current xy to match lcation"
            n485 = Enqueue Element At Opposite End(queue=w945, element="idle", error in (no error)=w940) -> (queue out=w944:refnum<queue>, error out=w943:errorcluster)  [unwired: 1 in, 1 out]
            n486 = flat-sequence {
              tunnel: [w951] -> w942
              tunnel: [w950] -> w941
              tunnel: w942 -> [w956]
              tunnel: w941 -> [w955]
              frame #0 {
                n487 = local read "Prober GPIB"() -> (w949:string)
                n488 = local write "Status"("Probe up" ("Status")) -> ()
                n489 = call "EG2001 Move Z Down.vi"("GPIB Address"=w949) -> ("Error Out"=w950:errorcluster, "GPIB Address Out"=w951:string)  [unwired: 9 in]
              }
              frame #1 {
                n490 = local read "current y"() -> (w959:i32)
                n491 = local read "current x"() -> (w961:i32)
                n492 = local read "y target"() -> (w960:i32)
                n493 = local read "x target"() -> (w962:i32)
                n494 = local write "Status"("Moving Probe" ("Status")) -> ()
                n495 = Subtract(x=w960, y=w959) -> (x-y=w957:i32)
                n496 = Subtract(x=w962, y=w961) -> (x-y=w958:i32)
                n497 = call "EG2001 Move Machine Step X-Y.vi"("Flip X Coordinates?"=FALSE, "Y"=w957, "Steps/Microns"=enum32{"Steps", "Microns"}."Microns", "X"=w958, "error in (no error)"=w955, "GPIB Address"=w956) -> ()  [unwired: 4 in, 2 out]
              }
              frame #2 {
                n498 = local read "y target"() -> (w964:i32)
                n499 = local read "x target"() -> (w965:i32)
                n500 = local write "Status"("Done" ("Status")) -> ()
                n501 = local write "current x"(w965) -> ()
                n502 = local write "current y"(w964) -> ()
              }
            }
          }
          frame "manual test" {
            # "Manual Test execution - first runs sweep VI, then measures the two points for the raw test. It doesn NOT save anywhere automatically, just displays results on the graph"
            n503 = Enqueue Element At Opposite End(queue=w969, element="idle", error in (no error)=w972) -> (queue out=w970:refnum<queue>, error out=w971:errorcluster)  [unwired: 1 in, 1 out]
            n504 = flat-sequence {
              tunnel: [w983] -> w980
              tunnel: [w982] -> w979
              tunnel: [w989] -> w978
              tunnel: w980 -> [w989]
              tunnel: [w988] -> w977
              tunnel: w979 -> [w988]
              tunnel: [w1014] -> w976
              tunnel: w978 -> [w1014]
              tunnel: [w1013] -> w975
              tunnel: w977 -> [w1013]
              tunnel: ["Measure 2 Point?"] -> w967
              tunnel: [w1045] -> w974
              tunnel: w976 -> [w1045]
              tunnel: [w1044] -> w973
              tunnel: w975 -> [w1044]
              tunnel: w967 -> [w1043]
              tunnel: [w1043] -> w966
              tunnel: w974 -> [w1081]
              tunnel: w973 -> [w1080]
              tunnel: w966 -> [w1074]
              frame #0 {
                n505 = local read "Prober GPIB"() -> (w984:string)
                n506 = call "EG2001 Move Z Up.vi"("GPIB Address"=w984) -> ("Error Out"=w982:errorcluster, "GPIB Address Out"=w983:string)  [unwired: 1 in, 8 out]
              }
              frame #1 {
                n507 = local read "Channel"() -> (w999:enum32{"Channel A", "Channel B"})
                n508 = local read "I compliance sweep"() -> (w994:dbl)
                n509 = local read "sweep delay ms"() -> (w993:dbl)
                n510 = local read "Sweep Settings"() -> (w1000:T10)
                n511 = local write "Status"("Sweeping IV Curve") -> ()
                n512 = local read "V start"() -> (w998:dbl)
                n513 = local read "points"() -> (w996:u16)
                n514 = local read "V end"() -> (w997:dbl)
                n515 = local read "NPLC"() -> (w995:dbl)
                n516 = Bundle By Name(cluster=w1000, "Channel"=w999, "Vstart"=w998, "Vend"=w997, "# of points"=w996, "NPLC"=w995, "I compliance"=w994, "Delay ms"=w993) -> (w992:T10)
                n517 = local read "4-wire"() -> (w986:bool)
                n518 = local read "Keysight"() -> (w985:bool)
                n519 = case shown="False" w985 {
                  tunnel: w992 -> [w1006 w1011]
                  tunnel: [w1003 w1010] -> w991
                  tunnel: [w1002 w1009] -> w990
                  tunnel: w986 -> [w1005 w1007]
                  frame False {
                    n520 = local read "Keysight SMU"() -> (w1004:refnum<visa-resource-name>)
                    n521 = call "IVSweep (SubVI).vi"("SweepSettings"=w1006, "4 wire"=w1005, "VISA Refnum in"=w1004, "Sweep Direction (0: Up)"="Sweep Direction (Keysight)") -> ("V"=w1002:dbl[], "I"=w1003:dbl[])  [unwired: 2 out]
                  }
                  frame True {
                    n522 = local read "Keithley SMU"() -> (w1008:refnum<visa-resource-name>)
                    n523 = call "K2602 Vsweep.vi"("4-wire"=w1007, "Settings"=w1011, "SMU"=w1008) -> ("V"=w1009:dbl[], "I"=w1010:dbl[])  [unwired: 6 in, 1 out]
                  }
                }
                "Varray manual" <- w990
                "Iarray manual" <- w991
              }
              frame #2 {
                n524 = case shown="False" "Measure 2 Point?" {
                  frame False {
                    n525 = local read "Iarray manual"() -> (w1016:dbl[])
                    n526 = Array Max & Min(array=w1016) -> (min value=w1015:dbl)  [unwired: 3 out]
                    n527 = local write "Imeas manual"(w1015) -> ()
                  }
                  frame True {
                    n528 = local read "Keysight"() -> (w1017:bool)
                    n529 = case shown="False" w1017 {
                      tunnel: [w1019 w1041] -> w1018
                      frame False {
                        n530 = local read "Channel Keysight"() -> (w1022:dbl)
                        n531 = local read "Id delay ms"() -> (w1025:dbl)
                        n532 = local read "Repeat Id"() -> (w1026:u32)
                        n533 = local read "Imeas Settings"() -> (w1030:T11)
                        n534 = local read "I compliance"() -> (w1027:dbl)
                        n535 = local read "4-wire"() -> (w1023:bool)
                        n536 = local write "Status"("Measuring I @ Vset") -> ()
                        n537 = local read "NPLC"() -> (w1028:dbl)
                        n538 = local read "V set"() -> (w1029:dbl)
                        n539 = Bundle By Name(cluster=w1030, "Channel"=w1022, "Vset"=w1029, "NPLC"=w1028, "I compliance"=w1027, "Repeat time"=w1026, "Delay ms"=w1025, "4-wire"=w1023) -> (w1021:T11)
                        n540 = local read "Keysight SMU"() -> (w1020:refnum<visa-resource-name>)
                        n541 = local write "Imeas Settings"(w1021) -> ()
                        n542 = call "Agilent B2900 Measure I at Vset.vi"("Imeas Settings"=w1021, "VISA resource name"=w1020) -> ("Avg I"=w1019:dbl)  [unwired: 9 in]
                      }
                      frame True {
                        n543 = local read "Id delay ms"() -> (w1035:dbl)
                        n544 = local read "Repeat Id"() -> (w1036:u32)
                        n545 = local read "Channel"() -> (w1040:enum32{"Channel A", "Channel B"})
                        n546 = local read "Imeas Settings"() -> (w1042:T11)
                        n547 = local read "I compliance"() -> (w1037:dbl)
                        n548 = local read "4-wire"() -> (w1033:bool)
                        n549 = local write "Status"("Measuring I @ Vset") -> ()
                        n550 = local read "NPLC"() -> (w1038:dbl)
                        n551 = local read "V set"() -> (w1039:dbl)
                        n552 = Bundle By Name(cluster=w1042, "Channel"=w1040, "Vset"=w1039, "NPLC"=w1038, "I compliance"=w1037, "Repeat time"=w1036, "Delay ms"=w1035, "4-wire"=w1033) -> (w1032:T11)
                        n553 = local read "Keithley SMU"() -> (w1031:refnum<visa-resource-name>)
                        n554 = local write "Imeas Settings"(w1032) -> ()
                        n555 = call "K2602 setVmeasI.vi"("Settings"=w1032, "SMU"=w1031) -> ("Iavg"=w1041:dbl)  [unwired: 6 in, 3 out]
                      }
                    }
                    n556 = local write "Imeas manual"(w1018) -> ()
                  }
                }
              }
              frame #3 {
                n557 = case shown="False" w1043 {
                  frame False {
                    n558 = local read "Varray manual"() -> (w1046:dbl[])
                    n559 = Array Max & Min(array=w1046) -> (min value=w1047:dbl)  [unwired: 3 out]
                    n560 = local write "Vmeas manual"(w1047) -> ()
                  }
                  frame True {
                    n561 = local read "Keysight"() -> (w1048:bool)
                    n562 = case shown="True" w1048 {
                      tunnel: [w1050 w1063] -> w1049
                      frame False {
                        n563 = local read "Vf delay ms"() -> (w1055:dbl)
                        n564 = local read "Repeat Vf"() -> (w1056:u32)
                        n565 = local read "Channel"() -> (w1060:enum32{"Channel A", "Channel B"})
                        n566 = local read "Vmeas Settings"() -> (w1061:T11)
                        n567 = local read "V compliance"() -> (w1057:dbl)
                        n568 = local read "4-wire"() -> (w1053:bool)
                        n569 = local write "Status"("Measuring V @ Iset") -> ()
                        n570 = local read "NPLC"() -> (w1058:dbl)
                        n571 = local read "I set"() -> (w1059:dbl)
                        n572 = Bundle By Name(cluster=w1061, "Channel"=w1060, "Vset"=w1059, "NPLC"=w1058, "I compliance"=w1057, "Repeat time"=w1056, "Delay ms"=w1055, "4-wire"=w1053) -> (w1052:T11)
                        n573 = local read "Keysight SMU"() -> (w1051:refnum<visa-resource-name>)
                        n574 = local write "Vmeas Settings"(w1052) -> ()
                        n575 = call "Agilent B2900 Measure V at Iset.vi"("Imeas Settings"=w1052, "VISA resource name"=w1051) -> ("Avg V"=w1050:dbl)  [unwired: 9 in]
                      }
                      frame True {
                        n576 = local read "Vf delay ms"() -> (w1067:dbl)
                        n577 = local read "Repeat Vf"() -> (w1068:u32)
                        n578 = local read "Channel"() -> (w1072:enum32{"Channel A", "Channel B"})
                        n579 = local read "Vmeas Settings"() -> (w1073:T11)
                        n580 = local read "V compliance"() -> (w1069:dbl)
                        n581 = local read "4-wire"() -> (w1065:bool)
                        n582 = local write "Status"("Measuring V @ Iset") -> ()
                        n583 = local read "NPLC"() -> (w1070:dbl)
                        n584 = local read "I set"() -> (w1071:dbl)
                        n585 = Bundle By Name(cluster=w1073, "Channel"=w1072, "Vset"=w1071, "NPLC"=w1070, "I compliance"=w1069, "Repeat time"=w1068, "Delay ms"=w1067, "4-wire"=w1065) -> (w1064:T11)
                        n586 = local read "Keithley SMU"() -> (w1062:refnum<visa-resource-name>)
                        n587 = call "K2602 setImeasV.vi"("Settings"=w1064, "SMU"=w1062) -> ("Vavg"=w1063:dbl)  [unwired: 6 in, 3 out]
                        n588 = local write "Vmeas Settings"(w1064) -> ()
                      }
                    }
                    n589 = local write "Vmeas manual"(w1049) -> ()
                  }
                }
              }
              frame #4 {
                n590 = call "EG2001 Move Z Down.vi"("error in (no error)"=w1080, "GPIB Address"=w1081) -> ()  [unwired: 8 in, 2 out]
                n591 = local write "Status"("Done") -> ()
                n592 = case shown="False" w1074 {
                  tunnel: [w1086 w1101] -> w1079
                  tunnel: [w1084 w1100] -> w1076
                  tunnel: [w1085 w1099] -> w1075
                  frame False {
                    n593 = local read "Manual IV settting"() -> (w1086:enum32{"Linear plot", "Log plot"})
                    n594 = local read "Vmeas manual"() -> (w1089:dbl)
                    n595 = local read "Varray manual"() -> (w1090:dbl[])
                    n596 = local read "Imeas manual"() -> (w1088:dbl)
                    n597 = local read "Iarray manual"() -> (w1083:dbl[])
                    n598 = local read "points"() -> (w1091:u16)
                    n599 = local read "V set"() -> (w1087:dbl)
                    n600 = Array Max & Min(array=w1083) -> (min value=w1082:dbl)  [unwired: 3 out]
                    n601 = call "get Plot.vi"("I set"=w1082, "Imeas"=w1088, "V set"=w1087, "Vmeas"=w1089, "Iarray"=w1083, "Varray"=w1090, "points"=w1091) -> ("logplot"=w1084:cluster{"Varray manual":dbl[], dbl[]}[], "Linearplot"=w1085:T18)  [unwired: 3 in]
                  }
                  frame True {
                    n602 = local read "Manual IV settting"() -> (w1101:enum32{"Linear plot", "Log plot"})
                    n603 = local read "Vmeas manual"() -> (w1095:dbl)
                    n604 = local read "Varray manual"() -> (w1097:dbl[])
                    n605 = local read "Imeas manual"() -> (w1094:dbl)
                    n606 = local read "Iarray manual"() -> (w1096:dbl[])
                    n607 = local read "points"() -> (w1098:u16)
                    n608 = local read "V set"() -> (w1093:dbl)
                    n609 = local read "I set"() -> (w1092:dbl)
                    n610 = call "get Plot.vi"("I set"=w1092, "Imeas"=w1094, "V set"=w1093, "Vmeas"=w1095, "Iarray"=w1096, "Varray"=w1097, "points"=w1098) -> ("logplot"=w1100:cluster{"Varray manual":dbl[], dbl[]}[], "Linearplot"=w1099:T18)  [unwired: 3 in]
                  }
                }
                "Manual Plot 0" <- w1075
                "Manaul Plot 1" <- w1076
                n611 = case shown="\"Linear plot\", Default" w1079 {
                  tunnel: w1075 -> [w1104 _]
                  tunnel: [w1104 w1107] -> w1078
                  tunnel: w1076 -> [_ w1107]
                  frame "Linear plot", Default {
                    n612 = property on="Manual IV" class="XYGraph (strict)"("YScale.Mapping Mode"=u8 0 ("Y Scale.Mapping Mode")) -> ()  [unwired: 2 in, 2 out]
                    n613 = property on="Manual IV" class="XYGraph (strict)"("YScale.NameLbl.Text"="Current (A)" ("X Scale.Name Label.Text")) -> ()  [unwired: 2 in, 2 out]
                  }
                  frame "Log plot" {
                    n614 = property on="Manual IV" class="XYGraph (strict)"("YScale.NameLbl.Text"="Abs(I)" ("Y Scale.Name Label.Text")) -> ()  [unwired: 2 in, 2 out]
                    n615 = property on="Manual IV" class="XYGraph (strict)"("YScale.Mapping Mode"=u8 1 ("Y Scale.Mapping Mode")) -> ()  [unwired: 2 in, 2 out]
                  }
                }
                "Manual IV" <- w1078
              }
              frame #5 {
                n616 = Two Button Dialog(message="Save Data?", 1:"Nay" ("F button name (\"Cancel\")"), 2:"Yea" ("T button name (\"OK\")")) -> (T button?=w1111:bool)
                n617 = case shown="True" w1111 {
                  frame False {
                  }
                  frame True {
                    n618 = flat-sequence {
                      tunnel: [w1117] -> w1113
                      tunnel: w1113 -> [w1140]
                      tunnel: [w1140] -> w1112
                      tunnel: w1112 -> [w1157]
                      frame #0 {
                        n619 = local read "Wafer Info 3"() -> (w1116:T2)
                        n620 = Bundle By Name(cluster=w1116, "Comment"="Manual Test Comments") -> (w1115:T2)
                        n621 = local write "Wafer Info 3"(w1115) -> ()
                      }
                      frame #1 {
                        n622 = local read "FineTest save path"() -> (w1124:path)
                        n623 = local read "Lot"() -> (w1125:string)
                        n624 = Build Path(base path=w1124, name or relative path=w1125) -> (appended path=w1126:path)
                        n625 = local read "Wafer Name"() -> (w1127:string)
                        n626 = call "CreateDirectory.vi"("Path to be created"=w1126) -> ()  [unwired: 10 in, 1 out]
                        n627 = Build Path(base path=w1126, name or relative path=w1127) -> (appended path=w1128:path)
                        n628 = local read "Output Power (mW)"() -> (w1119:dbl)
                        n629 = call "CreateDirectory.vi"("Path to be created"=w1128) -> ()  [unwired: 10 in, 1 out]
                        n630 = local read "Device Name"() -> (w1118:string)
                        n631 = Build Path(base path=w1128, name or relative path="IV") -> (appended path=w1130:path)
                        n632 = call "CreateDirectory.vi"("Path to be created"=w1130) -> ()  [unwired: 10 in, 1 out]
                        n633 = Number To Decimal String(number=w1119) -> (decimal integer string=w1121:string)  [unwired: 1 in]
                        n634 = Build Path(base path=w1130, name or relative path=w1118) -> (appended path=w1120:path)
                        n635 = call "CreateDirectory.vi"("Path to be created"=w1120) -> ()  [unwired: 10 in, 1 out]
                        n636 = Concatenate Strings(w1121, " mW" ("string")) -> (w1123:string)
                        n637 = Build Path(base path=w1120, name or relative path=w1123) -> (appended path=w1117:path)
                        n638 = call "CreateDirectory.vi"("Path to be created"=w1117) -> ()  [unwired: 10 in, 1 out]
                      }
                      frame #2 {
                        n639 = local read "I compliance sweep"() -> (w1135:dbl)
                        n640 = local read "sweep delay ms"() -> (w1134:dbl)
                        n641 = local read "Sweep Direction (Keysight)"() -> (w1139:i32)
                        n642 = local read "points"() -> (w1136:u16)
                        n643 = local read "V end"() -> (w1137:dbl)
                        n644 = local read "V start"() -> (w1138:dbl)
                        n645 = call "pho_DBCheck_LIV_meas_recipe.vi"("V start"=w1138, "Sweep Direction (Keysight)"=w1139, "V end"=w1137, "points"=w1136, "I compliance sweep"=w1135, "sweep delay ms"=w1134) -> ("RecipeID"=w1133:string)  [unwired: 8 in, 1 out]
                        n646 = local write "RecipeID"(w1133) -> ()
                        n647 = Equal?(x=w1133, y="") -> (x = y?=w1131:bool)
                        n648 = case shown="True" w1131 {
                          frame False {
                          }
                          frame True {
                            n649 = local read "I compliance sweep"() -> (w1143:dbl)
                            n650 = local read "sweep delay ms"() -> (w1142:dbl)
                            n651 = local read "Sweep Direction (Keysight)"() -> (w1147:i32)
                            n652 = local read "points"() -> (w1144:u16)
                            n653 = local read "V end"() -> (w1145:dbl)
                            n654 = local read "V start"() -> (w1146:dbl)
                            n655 = call "pho_DB_Insert_LIV_meas_recipe.vi"("V start"=w1146, "Sweep Direction (Keysight)"=w1147, "V end"=w1145, "points"=w1144, "I compliance sweep"=w1143, "sweep delay ms"=w1142) -> ("RecipeID"=w1141:string)  [unwired: 9 in]
                            n656 = local write "RecipeID"(w1141) -> ()
                          }
                        }
                      }
                      frame #3 {
                        n657 = local read "current y"() -> (w1163:i32)
                        n658 = local read "current x"() -> (w1162:i32)
                        n659 = local read "Temp Data"() -> (w1151:T1)
                        n660 = local read "Device Name"() -> (w1159:string)
                        n661 = local read "Wafer Name"() -> (w1158:string)
                        n662 = local read "Varray manual"() -> (w1165:dbl[])
                        n663 = local read "Iarray manual"() -> (w1164:dbl[])
                        n664 = local read "Operator"() -> (w1148:string)
                        n665 = To Double Precision Float(number=w1162) -> (double precision float=w1160:dbl)
                        n666 = To Double Precision Float(number=w1163) -> (double precision float=w1161:dbl)
                        n667 = Get Date/Time In Seconds() -> (seconds since 1Jan1904=w1170:timestamp)
                        n668 = local read "Parameters Flash"() -> (w1153:T4)
                        n669 = local read "RecipeID"() -> (w1152:string)
                        n670 = local read "Wafer Info 3"() -> (w1150:T2)
                        n671 = call "get Flash FileName .vi"("Time"=w1170, "Device Name"=w1159, "Operator"=w1148, "Wafer Name"=w1158, "FineTest save path"=w1157) -> ("appended path"=w1154:path)  [unwired: 6 in]
                        n672 = Build Array(w1165, w1164) -> (w1156:dbl[][])
                        n673 = Bundle(w1160, w1161) -> (w1149:cluster{dbl, dbl})  [unwired: 1 in]
                        n674 = Get Date/Time String(seconds (now)=w1170, want seconds? (F)=TRUE) -> (date string=w1166:string, time string=w1168:string)  [unwired: 1 in]
                        n675 = local read "Mask"() -> (w1155:string)
                        n676 = call <vilib>:"Space Constant.vi"() -> ("String"=w1169:string)
                        n677 = Concatenate Strings(w1166, w1169, w1168) -> ()  [unwired: 1 out]
                        n678 = call "WriteFlashFile NEW.vi"("Input File Path"=w1154, "IV array"=w1156, "Parameters"=w1153, "RecipeID"=w1152, "User"=w1148, "Coords"=w1149, "Wafer Info"=w1150, "Mask Name"=w1155, "Temp Data"=w1151) -> ()  [unwired: 18 in, 1 out]
                      }
                    }
                  }
                }
              }
            }
          }
          frame "generate prelim report" {
            n679 = call <vilib>:"System Exec.vi"("wait until completion? (T)"=FALSE, "working directory"=path "C:/Users/Flash/Documents/GitHub/solarjunction", "command line"="C:\\Windows\\system32\\cmd.exe /k python3 generate_prelim_report.py") -> ()  [unwired: 5 in, 4 out]
          }
          frame "update wafer" {
            # "Takes wafer name and pulls info from the database, and updates relevant variables"
            n680 = local read "Wafer Name"() -> (w1178:string)
            n681 = Enqueue Element At Opposite End(queue=w1187, element="idle", error in (no error)=w1180) -> (queue out=w1186:refnum<queue>, error out=w1185:errorcluster)  [unwired: 1 in, 1 out]
            n682 = call "getDB Wafer Info.vi"("Wafer Name"=w1178) -> ("WaferInfo"=w1179:T19)  [unwired: 9 in, 1 out]
            n683 = Unbundle By Name(w1179) -> ("WaferName"=w1176:string, "Scribe"=w1184:string, "Lot"=w1183:string, "Mask"=w1182:string)  [unwired: 1 out]
            n684 = local write "Scribe"(w1184) -> ()
            n685 = local write "Lot"(w1183) -> ()
            n686 = local write "Mask"(w1182) -> ()
            n687 = Equal?(x=w1178, y=w1176) -> (x = y?=w1177:bool)
            n688 = case shown="True" w1177 {
              tunnel: w1176 -> [w1189 _]
              frame False {
                n689 = local write "Wafer Name"(w1189) -> ()
              }
              frame True {
              }
            }
          }
          frame "desired wafer to current wafer" {
            # "This only runs in the lot test. It updates the wafer name from the wafer list. The Wafer counter keeps track of the iteration of the auto test the lot test is currently on. Once the wafer name is updated, the Wafer counter in incremented by one. If the Wafer list has reached its end, the wafer counter is returned to 0"
            n690 = flat-sequence {
              frame #0 {
                n691 = local read "WaferCounter"() -> (w1194:i32)
                n692 = property on="Wafer List" class="LstBox (strict)"() -> ("Item Names"=w1193:string[])  [unwired: 2 in, 2 out]
                n693 = Index Array(array=w1193, index=w1194) -> (element=w1192:string)
                n694 = local write "Wafer Name"(w1192) -> ()
              }
              frame #1 {
                n695 = local read "WaferCounter"() -> (w1196:i32)
                n696 = Increment(x=w1196) -> (x+1=w1195:i32)
                n697 = local write "WaferCounter"(w1195) -> ()
              }
              frame #2 {
                n698 = local read "WaferCounter"() -> (w1198:i32)
                n699 = property on="Wafer List" class="LstBox (strict)"() -> ("Item Names"=w1200:string[])  [unwired: 2 in, 2 out]
                n700 = Array Size(array=w1200) -> (size(s)=w1199:i32)
                n701 = Equal?(x=w1199, y=w1198) -> (x = y?=w1197:bool)
                n702 = case shown="True" w1197 {
                  frame False {
                  }
                  frame True {
                    n703 = local write "WaferCounter"(0 ("WaferCounter")) -> ()
                  }
                }
              }
            }
          }
          frame "idle" {
            n704 = local write "Status"("idle" ("Status")) -> ()
          }
          frame "change plot" {
            # "Switch from linear to logarithmic plot and back on the maual test tab"
            n705 = Enqueue Element At Opposite End(queue=w1207, element="idle", error in (no error)=w1209) -> (queue out=w1206:refnum<queue>, error out=w1208:errorcluster)  [unwired: 1 in, 1 out]
            n706 = local read "Manual IV settting"() -> (w1213:enum32{"Linear plot", "Log plot"})
            n707 = case shown="\"Log plot\"" w1213 {
              tunnel: [w1216 w1219] -> w1212
              frame "Linear plot", Default {
                n708 = property on="Manual IV" class="XYGraph (strict)"("YScale.Mapping Mode"=u8 0 ("Y Scale.Mapping Mode")) -> ()  [unwired: 2 in, 2 out]
                n709 = local read "Manual Plot 0"() -> (w1216:cluster{"V manual":dbl[], "I manual":dbl[]}[])
                n710 = property on="Manual IV" class="XYGraph (strict)"("YScale.NameLbl.Text"="Current (A)" ("Y Scale.Name Label.Text")) -> ()  [unwired: 2 in, 2 out]
              }
              frame "Log plot" {
                n711 = property on="Manual IV" class="XYGraph (strict)"("YScale.Mapping Mode"=u8 1 ("Y Scale.Mapping Mode")) -> ()  [unwired: 2 in, 2 out]
                n712 = property on="Manual IV" class="XYGraph (strict)"("YScale.NameLbl.Text"="Abs(I)" ("Y Scale.Name Label.Text")) -> ()  [unwired: 2 in, 2 out]
                n713 = local read "Manaul Plot 1"() -> (w1219:cluster{"V manual":dbl[], dbl[]}[])
              }
            }
            n714 = local write "Manual IV"(w1212) -> ()
          }
          frame "select" {
            # "Selects Best ten devices (in seperate VI). If less than ten devices are within the voltage and current bounds, it selects all the devices that are within the parameters. If no devices are in the parameters, it still saves the mask file but it will be empty"
            n715 = local read "Raw Test Skipped"() -> (w1221:bool)
            n716 = Enqueue Element At Opposite End(queue=w1224, element="idle", error in (no error)=w1223) -> (queue out=w1226:refnum<queue>, error out=w1225:errorcluster)  [unwired: 1 in, 1 out]
            n717 = Not(x=w1221) -> (.not. x?=w1220:bool)
            n718 = case shown="True" w1220 {
              frame False {
              }
              frame True {
                n719 = local read "I meas"() -> (w1230:dbl[])
                n720 = Array Size(array=w1230) -> (size(s)=w1228:i32)
                n721 = Greater Than 0?(x=w1228) -> (x > 0?=w1229:bool)
                n722 = case shown="True" w1229 {
                  tunnel: w1228 -> [_ w1248]
                  frame False {
                  }
                  frame True {
                    n723 = Initialize Array(nan ("element"), w1248) -> (w1244:dbl[])
                    n724 = local read "Wafer Name"() -> (w1256:string)
                    n725 = local read "RawData file"() -> (w1236:path)
                    n726 = local read "new raw data save path"() -> (w1250:path)
                    n727 = local read "V meas"() -> (w1240:dbl[])
                    n728 = local read "I meas"() -> (w1239:dbl[])
                    n729 = local read "Laser Current (mA)"() -> (w1233:dbl)
                    n730 = local read "Number Select"() -> (w1254:u16)
                    n731 = local read "Mask File Raw"() -> (w1255:path)
                    n732 = Bundle("V meas"=w1240, "I meas"=w1239) -> (w1238:cluster{"V meas":dbl[], "I meas":dbl[]})  [unwired: 1 in]
                    n733 = Greater Than 0?(x=w1233) -> (x > 0?=w1232:bool)
                    n734 = local read "Vmax"() -> (w1253:dbl)
                    n735 = local read "Vmin"() -> (w1252:dbl)
                    n736 = call "select RawTestData.vi"("Light > 0?"=w1232, "Number Select"=w1254, "Vmax"=w1253, "Vmin"=w1252, "V meas"=w1240, "I meas"=w1239) -> ("Selected V"=w1247:dbl[], "Selected I"=w1245:dbl[], "Selected Index"=w1234:dbl[])  [unwired: 2 in, 1 out]
                    n737 = call "save FineMask.vi"("Selected Index"=w1234, "RawData Save Path"=w1250, "Text Add"=w1256, "Mask File Raw"=w1255) -> ("Output path"=w1251:path)  [unwired: 7 in]
                    n738 = call "updatedFile RawTestSelect.vi"("Column Number"=u32 21, "Selected Index"=w1234, "Path"=w1236) -> ()  [unwired: 9 in]
                    n739 = local write "Mask File Fine"(w1251) -> ()
                    n740 = Replace Array Subset(array=w1244, new element=w1247, index=0) -> (w1242:dbl[])
                    n741 = Replace Array Subset(array=w1244, new element=w1245, index=0) -> (w1241:dbl[])
                    n742 = Bundle(w1242, w1241) -> (w1231:cluster{dbl[], dbl[]})  [unwired: 1 in]
                    n743 = Build Array(w1238, w1231) -> (w1237:cluster{"V meas":dbl[], "I meas":dbl[]}[])
                    n744 = local write "Spec Plot"(w1237) -> ()
                  }
                }
              }
            }
          }
          frame "update measurement log" {
            # "Collects measurement parameters (such a test type) and saves them to the measurement log CSV file."
            n745 = flat-sequence {
              tunnel: [w1269] -> w1259
              tunnel: w1259 -> [w1285]
              tunnel: [w1276] -> w1258
              tunnel: w1258 -> [w1297]
              frame #0 {
                n746 = local read "Wafer Name"() -> (w1273:string)
                n747 = local read "Operator"() -> (w1272:string)
                n748 = Get Date/Time In Seconds() -> (seconds since 1Jan1904=w1271:timestamp)
                n749 = local read "Test Type"() -> (w1262:string)
                n750 = Get Date/Time String(seconds (now)=w1271) -> (date string=w1265:string, time string=w1270:string)  [unwired: 2 in]
                n751 = Search and Replace String(replace all?=TRUE ("replace all? (F)"), input string=w1265, search string="/", replace string="_" ("replace string (\"\")")) -> (result string=w1264:string)  [unwired: 4 in, 3 out]
                n752 = Bundle("result string"=w1264, "time string"=w1270, "Wafer Name"=w1273, "Operator"=w1272, "Test description"="Test description", "Test Type"=w1262) -> (w1269:T15)  [unwired: 1 in]
                "Last Measurement" <- w1269
              }
              frame #1 {
                w1274 = ","
                n753 = Unbundle(w1285) -> ("result string"=w1281:string, "time string"=w1280:string, "Wafer Name"=w1279:string, "Operator"=w1278:string, "Test description"=w1277:string, "Test Type"=w1275:string)
                n754 = Concatenate Strings(w1281, w1274, w1280, w1274, w1279, w1274, w1278, w1274, w1277, w1274, w1275) -> (w1282:string)
                n755 = call <vilib>:"Check if File or Folder Exists.vi"("path"=path "C:/Users/Flash/Desktop/Data/Detector test data/MeasurementLog.csv") -> ("file or folder exists?"=w1283:bool, "dup path"=w1276:path)  [unwired: 1 in, 8 out]
                n756 = case shown="True" w1283 {
                  tunnel: w1276 -> [w1290 w1295]
                  tunnel: w1282 -> [w1287 w1292]
                  frame False {
                    n757 = Build Array(w1287) -> (w1286:string[])
                    n758 = call-poly <vilib>:"Write To Spreadsheet File.vi"("delimiter (\\t)"="," ("delimiter (\\t)"), "append to file? (new file:F)"=FALSE, "1D data"=w1286, "file path (dialog if empty)"=w1290) -> ()  [unwired: 4 in, 1 out]
                  }
                  frame True {
                    n759 = Build Array(w1292) -> (w1291:string[])
                    n760 = call-poly <vilib>:"Write To Spreadsheet File.vi"("delimiter (\\t)"="," ("delimiter (\\t)"), "append to file? (new file:F)"=TRUE, "1D data"=w1291, "file path (dialog if empty)"=w1295) -> ()  [unwired: 4 in, 1 out]
                  }
                }
              }
              frame #2 {
                n761 = call-poly <vilib>:"Read From Spreadsheet File.vi"("file path (dialog if empty)"=w1297) -> ("all rows"=w1296:string[][])  [unwired: 6 in, 4 out]
                n762 = property on="Logview" class="MCListbox (strict)"("ItemNames"=w1296) -> ()  [unwired: 2 in, 2 out]
              }
            }
          }
          frame "load raw data" {
            # "Prompts the user to pick a raw data file, and then displays that data on the graphical display  on the raw test tab"
            n763 = Enqueue Element At Opposite End(queue=w1305, element="idle", error in (no error)=w1304) -> (queue out=w1307:refnum<queue>, error out=w1306:errorcluster)  [unwired: 1 in, 1 out]
            n764 = local read "RawData Save Path"() -> (w1298:path)
            n765 = call "File Dialog"("start path"=w1298, "prompt"="Please pick a raw test data file", "pattern (all files)"="*.csv" ("pattern label")) -> ("selected path"=w1300:path, "cancelled"=w1303:bool)  [unwired: 9 in, 2 out]
            n766 = case shown="False" w1303 {
              tunnel: w1300 -> [_ w1310]
              frame True {
              }
              frame False {
                n767 = Strip Path(path=w1310) -> (stripped path=w1309:path)  [unwired: 1 out]
                n768 = local write "new raw data save path"(w1309) -> ()
                n769 = local write "RawData file"(w1310) -> ()
                n770 = Strip Path(path=w1310) -> (name=w1311:string)  [unwired: 1 out]
                n771 = call "read Raw.vi"("Path"=w1310) -> ("Session Info"=w1329:T20, "Die Info"=w1338:T21, "Wafer Info"=w1337:T9, "V"=w1315:dbl[], "I"=w1314:dbl[])  [unwired: 6 in]
                n772 = local write "Test FileName"(w1311) -> ()
                n773 = local write "I meas"(w1314) -> ()
                n774 = local write "V meas"(w1315) -> ()
                n775 = Unbundle By Name(w1329) -> ("V set"=w1328:dbl, "I compliance"=w1327:dbl, "J set"=w1326:dbl, "I set"=w1325:dbl, "V compliance"=w1324:dbl, "Laser Power (mW)"=w1322:dbl, "Operator"=w1323:string)
                n776 = Unbundle By Name(w1338) -> ("Device Name"=w1332:string, "ActiveArea_um2"=w1331:dbl, "MesaArea_um2"=w1330:dbl)
                n777 = Unbundle By Name(w1337) -> ("Wafer Name"=w1336:string, "Scribe"=w1335:string, "Mask"=w1334:string, "Lot"=w1333:string)
                n778 = Array Size(array=w1314) -> (size(s)=w1320:i32)
                n779 = Bundle("V"=w1315, "I"=w1314) -> (w1318:cluster{"V":dbl[], "I":dbl[]})  [unwired: 1 in]
                n780 = call <vilib>:"Histogram.vi"("X"=w1315) -> ("Histogram Graph"=w1312:T14)  [unwired: 7 in, 3 out]
                n781 = call <vilib>:"Histogram.vi"("X"=w1314) -> ("Histogram Graph"=w1313:T14)  [unwired: 7 in, 3 out]
                n782 = local write "Mask"(w1334) -> ()
                n783 = local write "Lot"(w1333) -> ()
                n784 = local write "V set"(w1328) -> ()
                n785 = local write "I set"(w1325) -> ()
                n786 = local write "Vforward hist"(w1312) -> ()
                n787 = local write "Idark hist"(w1313) -> ()
                n788 = local write "Scribe"(w1335) -> ()
                n789 = local write "MesaArea_um2"(w1330) -> ()
                n790 = local write "Device Name"(w1332) -> ()
                n791 = local write "ActiveArea_um2"(w1331) -> ()
                n792 = Initialize Array(nan ("element"), w1320) -> (w1319:dbl[])
                n793 = local write "Laser Current (mA)"(w1322) -> ()
                n794 = local write "Operator"(w1323) -> ()
                n795 = local write "Wafer Name"(w1336) -> ()
                n796 = local write "I compliance"(w1327) -> ()
                n797 = local write "J set A/cm2"(w1326) -> ()
                n798 = local write "V compliance"(w1324) -> ()
                n799 = Bundle(w1319, w1319) -> (w1317:cluster{dbl[], dbl[]})  [unwired: 1 in]
                n800 = local write "Selected Data"(w1317) -> ()
                n801 = Build Array(w1318, w1317) -> (w1316:cluster{"V":dbl[], "I":dbl[]}[])
                n802 = local write "Spec Plot"(w1316) -> ()
              }
            }
          }
          frame "start fine" {
            # "Executes Fine test. If \"no file\" is true, it means that raw test was skipped, but then no previous raw data was found to run the fine test. The fine test will be skipped in this case.\n1) Loads  the fine mask files and updates relevant parameters\n2) Passes the parameters to the data clusters. There are three data clusters due to different versions of the save flash file. It saves the wafer information, time and date, current power, temperature, and other assorted parameters. Many parameters are leftover from the solar cell testing program, and are consequently always left as 0.\n3)The sweep is run using the Keithley sweep sub VI\n4) The directory is found/created to save the IV file (see guide for saving structure)\n5) data is saved and prober is returned to 0  0"
            n803 = flat-sequence {
              tunnel: w1344 -> [w1348]
              frame #0 {
                n804 = local read "no file"() -> (w1347:bool)
                n805 = Not(x=w1347) -> (.not. x?=w1346:bool)
                n806 = case shown="True" w1346 {
                  tunnel: w1348 -> [_ w1349]
                  frame False {
                  }
                  frame True {
                    n807 = flat-sequence {
                      tunnel: [w1355] -> w1350
                      tunnel: w1349 -> [w1353]
                      tunnel: w1350 -> [w1367]
                      frame #0 {
                        w1356 = u8 0 ("Progress 2")
                        n808 = local read "points"() -> (w1358:u16)
                        n809 = local write "Progress 2"(w1356) -> ()
                        n810 = Initialize Array(nan ("element"), w1358) -> (w1360:dbl[])
                        n811 = local write "Tab Control"(T16."Fine Test" ("Tab Control")) -> ()
                        n812 = local write "Status"("prepare fine test" ("Status")) -> ()
                        n813 = Bundle(w1360, w1360) -> (w1359:cluster{dbl[], dbl[]})  [unwired: 1 in]
                        n814 = case shown="True" w1353 {
                          tunnel: "Mask File Fine" -> [w1365 w1366]
                          tunnel: [w1365 w1366] -> w1351
                          frame False {
                          }
                          frame True {
                          }
                        }
                        n815 = local write "Mask File Fine"(w1351) -> ()
                        n816 = call "Device Files v1.vi"("Rows"=1200, "Mask file path"=w1351) -> ("size(s)"=w1355:i32, "Array of Cell Clusters"=→"Fine Cell Clusters":T5)  [unwired: 6 in, 2 out]
                        "Total Device" <- w1355
                        n817 = Initialize Array(w1359, w1355) -> (→"IV fine linear" →"IV fine log":cluster{dbl[], dbl[]}[])
                        "Current Device" <- w1356
                      }
                      frame #1 {
                        n818 = for {
                          N: w1367 -> [w1397]
                          i -> [w1398]
                          n819 = flat-sequence {
                            tunnel: w1398 -> [w1413]
                            tunnel: [w1421] -> w1392
                            tunnel: [w1420] -> w1391
                            tunnel: [w1417] -> w1390
                            tunnel: [w1416] -> w1389
                            tunnel: [w1415] -> w1388
                            tunnel: [w1414] -> w1387
                            tunnel: [w1413] -> w1379
                            tunnel: w1392 -> [w1436]
                            tunnel: w1391 -> [w1435]
                            tunnel: w1390 -> [w1433]
                            tunnel: w1389 -> [w1432]
                            tunnel: w1388 -> [w1431]
                            tunnel: w1387 -> [w1430]
                            tunnel: [w1429] -> w1386
                            tunnel: [w1428] -> w1385
                            tunnel: [w1427] -> w1380
                            tunnel: w1379 -> [w1427]
                            tunnel: w1386 -> [w1439]
                            tunnel: w1385 -> [w1438]
                            tunnel: [w1437] -> w1381
                            tunnel: w1380 -> [w1437]
                            tunnel: [w1450] -> w1375
                            tunnel: w1381 -> [w1450]
                            tunnel: w1375 -> [w1476]
                            tunnel: [w1476] -> w1374
                            tunnel: w1374 -> [w1491]
                            tunnel: [w1491] -> w1377
                            tunnel: [w1484] -> w1376
                            tunnel: w1377 -> [w1512]
                            tunnel: [w1503] -> w1373
                            tunnel: [w1497] -> w1372
                            tunnel: [w1496] -> w1371
                            tunnel: w1376 -> [w1495]
                            tunnel: [w1525] -> w1370
                            tunnel: [w1526] -> w1369
                            tunnel: [w1527] -> w1368
                            tunnel: w1371 -> [w1527]
                            tunnel: w1372 -> [w1526]
                            tunnel: w1373 -> [w1525]
                            tunnel: w1370 -> [w1551]
                            tunnel: w1369 -> [w1538]
                            tunnel: w1368 -> [w1545]
                            frame #0 {
                              n820 = local read "Prober GPIB"() -> (w1422:string)
                              n821 = local read "current y"() -> (w1418:i32)
                              n822 = local read "current x"() -> (w1419:i32)
                              n823 = local read "Laser Current (mA)"() -> (w1409:dbl)
                              n824 = local read "Laser Current (mA)"() -> (w1407:dbl)
                              n825 = local read "Parameters Flash 2"() -> (w1412:T4)
                              n826 = local read "Fine Cell Clusters"() -> (w1426:T5)
                              n827 = local read "ActiveArea_um2"() -> (w1405:dbl)
                              n828 = local read "Output Power (mW)"() -> (w1403:dbl)
                              n829 = local read "Output Power (mW)"() -> (w1406:dbl)
                              n830 = call "EG2001 Move Z Down.vi"("GPIB Address"=w1422) -> ("Error Out"=w1420:errorcluster, "GPIB Address Out"=w1421:string)  [unwired: 9 in]
                              n831 = Divide(x=w1405, y=100000000.0) -> (x/y=w1400:dbl)
                              n832 = Index Array(array=w1426, index=w1413) -> (element=w1410:T22)
                              n833 = Unbundle By Name(w1410) -> ("Cell Name"=w1425:string, "X-coord"=w1415:dbl, "Y-coord"=w1414:dbl, "Area"=w1424:dbl, "Mesa Area"=w1423:dbl)
                              n834 = call "get Area.vi"("Laser"=w1409, "Cell Data Cluster"=w1410) -> ("Area"=w1411:dbl)  [unwired: 9 in]
                              n835 = Multiply(x=w1403, y=0.001) -> (x*y=w1401:dbl)
                              n836 = Subtract(x=w1414, y=w1418) -> (x-y=w1416:dbl)
                              n837 = Subtract(x=w1415, y=w1419) -> (x-y=w1417:dbl)
                              n838 = local write "Device Name"(w1425) -> ()
                              n839 = local write "ActiveArea_um2"(w1424) -> ()
                              n840 = local write "MesaArea_um2"(w1423) -> ()
                              n841 = Divide(x=w1401, y=w1400) -> (x/y=w1399:dbl)
                              n842 = Bundle By Name(cluster=w1412, "Cell Area (cm²)"=w1411, "Input Current (mA)"=w1407, "Power Density (W/cm^2)"=w1399, "Incident Power"=w1406) -> (w1408:T4)
                              n843 = local write "Parameters Flash"(w1408) -> ()
                            }
                            frame #1 {
                              n844 = local write "current x"(w1431) -> ()
                              n845 = local write "current y"(w1430) -> ()
                              n846 = call "EG2001 Move Machine Step X-Y.vi"("Y"=w1432, "Steps/Microns"=enum32{"Steps", "Microns"}."Microns", "X"=w1433, "error in (no error)"=w1435, "GPIB Address"=w1436) -> ("Error Out"=w1428:errorcluster, "GPIB Address Out"=w1429:string)  [unwired: 5 in]
                            }
                            frame #2 {
                              n847 = call "EG2001 Move Z Up.vi"("error in (no error)"=w1438, "GPIB Address"=w1439) -> ()  [unwired: 10 out]
                            }
                            frame #3 {
                              n848 = call "DAQ Assistant"() -> ("data"=w1443:dynamicdata)  [unwired: 17 in, 2 out]
                              n849 = local read "Channel"() -> (w1459:enum32{"Channel A", "Channel B"})
                              n850 = local read "Temp Setpoint"() -> (w1445:string)
                              n851 = local read "Wafer Info Flash 2"() -> (w1449:T3)
                              n852 = local read "I compliance sweep"() -> (w1454:dbl)
                              n853 = local read "sweep delay ms"() -> (w1453:dbl)
                              n854 = local read "Sweep Settings"() -> (w1461:T10)
                              n855 = local read "Device Name"() -> (w1448:string)
                              n856 = local read "Temp Data"() -> (w1446:T1)
                              n857 = Decimal String To Number(string=w1445) -> (number=w1442:i32)  [unwired: 2 in, 1 out]
                              n858 = Bundle By Name(cluster=w1449, "Cell Name"=w1448) -> (w1447:T3)
                              n859 = Bundle By Name(cluster=w1446, "Ambient Temperature"=w1443, "Chuck Set Temperature"=w1442) -> (w1444:T1)
                              n860 = local read "V start"() -> (w1457:dbl)
                              n861 = local read "points"() -> (w1456:u16)
                              n862 = local read "V end"() -> (w1458:dbl)
                              n863 = local read "NPLC"() -> (w1455:dbl)
                              n864 = local write "Wafer Info Flash"(w1447) -> ()
                              n865 = Bundle By Name(cluster=w1461, "Channel"=w1459, "Vstart"=w1457, "Vend"=w1458, "# of points"=w1456, "NPLC"=w1455, "I compliance"=w1454, "Delay ms"=w1453) -> (w1460:T10)
                              n866 = local write "Temp Data"(w1444) -> ()
                              n867 = local read "4-wire"() -> (w1440:bool)
                              n868 = local read "Keysight"() -> (w1441:bool)
                              n869 = case shown="False" w1441 {
                                tunnel: w1460 -> [w1467 w1472]
                                tunnel: [w1464 w1471] -> w1452
                                tunnel: [w1465 w1470] -> w1451
                                tunnel: w1440 -> [w1466 w1469]
                                frame False {
                                n870 = local read "Sweep Direction (Keysight)"() -> (w1462:i32)
                                n871 = call "IVSweep (SubVI).vi"("SweepSettings"=w1467, "4 wire"=w1466, "VISA Refnum in"="Keysight SMU", "Sweep Direction (0: Up)"=w1462) -> ("V"=w1465:dbl[], "I"=w1464:dbl[])  [unwired: 2 out]
                                }
                                frame True {
                                n872 = local read "Keithley SMU"() -> (w1468:refnum<visa-resource-name>)
                                n873 = call "K2602 Vsweep.vi"("4-wire"=w1469, "Settings"=w1472, "SMU"=w1468) -> ("V"=w1470:dbl[], "I"=w1471:dbl[])  [unwired: 6 in, 1 out]
                                }
                              }
                              n874 = local write "I fine"(w1452) -> ()
                              n875 = local write "V fine"(w1451) -> ()
                            }
                            frame #4 {
                              n876 = local read "Device Name"() -> (w1474:string)
                              n877 = local read "Wafer Info 3"() -> (w1475:T2)
                              n878 = Bundle By Name(cluster=w1475, "Cell Name (Automatic)"=w1474) -> (w1473:T2)
                              n879 = local write "Wafer Info 3"(w1473) -> ()
                            }
                            frame #5 {
                              n880 = local read "FineTest save path"() -> (w1483:path)
                              n881 = local read "Lot"() -> (w1482:string)
                              n882 = local read "Wafer Name"() -> (w1480:string)
                              n883 = local read "Device Name"() -> (w1490:string)
                              n884 = local read "Output Power (mW)"() -> (w1489:dbl)
                              n885 = Build Path(base path=w1483, name or relative path=w1482) -> (appended path=w1481:path)
                              n886 = call "CreateDirectory.vi"("Path to be created"=w1481) -> ()  [unwired: 10 in, 1 out]
                              n887 = Build Path(base path=w1481, name or relative path=w1480) -> (appended path=w1479:path)
                              n888 = Number To Decimal String(number=w1489) -> (decimal integer string=w1487:string)  [unwired: 1 in]
                              n889 = call "CreateDirectory.vi"("Path to be created"=w1479) -> ()  [unwired: 10 in, 1 out]
                              n890 = Concatenate Strings(w1487, " mW" ("string")) -> (w1485:string)
                              n891 = Build Path(base path=w1479, name or relative path="IV") -> (appended path=w1477:path)
                              n892 = call "CreateDirectory.vi"("Path to be created"=w1477) -> ()  [unwired: 10 in, 1 out]
                              n893 = Build Path(base path=w1477, name or relative path=w1490) -> (appended path=w1488:path)
                              n894 = call "CreateDirectory.vi"("Path to be created"=w1488) -> ()  [unwired: 10 in, 1 out]
                              n895 = Build Path(base path=w1488, name or relative path=w1485) -> (appended path=w1484:path)
                              n896 = call "CreateDirectory.vi"("Path to be created"=w1484) -> ()  [unwired: 10 in, 1 out]
                            }
                            frame #6 {
                              n897 = local read "V fine"() -> (w1502:dbl[])
                              n898 = local read "I fine"() -> (w1508:dbl[])
                              n899 = local read "Wafer Name"() -> (w1506:string)
                              n900 = local read "IV fine linear"() -> (w1515:cluster{dbl[], dbl[]}[])
                              n901 = local read "Comments"() -> (w1493:string)
                              n902 = local read "IV fine log"() -> (w1510:cluster{dbl[], dbl[]}[])
                              n903 = local read "Operator"() -> (w1505:string)
                              n904 = local read "current y"() -> (w1498:i32)
                              n905 = local read "current x"() -> (w1499:i32)
                              n906 = Bundle("V fine"=w1502, "I fine"=w1508) -> (w1513:cluster{"V fine":dbl[], "I fine":dbl[]})  [unwired: 1 in]
                              n907 = Absolute Value(x=w1508) -> (abs(x)=w1509:dbl[])
                              n908 = local read "Device Name"() -> (w1504:string)
                              n909 = Replace Array Subset(array=w1515, new element=w1513, index=w1512) -> (w1514:cluster{dbl[], dbl[]}[])
                              n910 = To Double Precision Float(number=w1499) -> (double precision float=w1501:dbl)
                              n911 = To Double Precision Float(number=w1498) -> (double precision float=w1500:dbl)
                              n912 = Bundle("V fine"=w1502, w1509) -> (w1507:cluster{"V fine":dbl[], dbl[]})  [unwired: 1 in]
                              n913 = Get Date/Time In Seconds() -> (seconds since 1Jan1904=w1496:timestamp)
                              n914 = local read "Wafer Info 3"() -> (w1494:T2)
                              n915 = Bundle By Name(cluster=w1494, "Comment"=w1493) -> (w1492:T2)
                              n916 = local write "IV fine linear"(w1514) -> ()
                              n917 = call "get Flash FileName .vi"("Time"=w1496, "Device Name"=w1504, "Operator"=w1505, "Wafer Name"=w1506, "FineTest save path"=w1495) -> ("appended path"=w1503:path)  [unwired: 6 in]
                              n918 = Replace Array Subset(array=w1510, new element=w1507, index=w1512) -> (w1511:cluster{dbl[], dbl[]}[])
                              n919 = Bundle(w1501, w1500) -> (w1497:cluster{dbl, dbl})  [unwired: 1 in]
                              n920 = local write "IV fine log"(w1511) -> ()
                              n921 = local write "Wafer Info 3"(w1492) -> ()
                            }
                            frame #7 {
                              n922 = local read "I compliance sweep"() -> (w1520:dbl)
                              n923 = local read "sweep delay ms"() -> (w1521:dbl)
                              n924 = local read "Sweep Direction (Keysight)"() -> (w1516:i32)
                              n925 = local read "points"() -> (w1519:u16)
                              n926 = local read "V end"() -> (w1518:dbl)
                              n927 = local read "V start"() -> (w1517:dbl)
                              n928 = call "pho_DBCheck_LIV_meas_recipe.vi"("V start"=w1517, "Sweep Direction (Keysight)"=w1516, "V end"=w1518, "points"=w1519, "I compliance sweep"=w1520, "sweep delay ms"=w1521) -> ("RecipeID"=w1522:string)  [unwired: 8 in, 1 out]
                              n929 = local write "RecipeID"(w1522) -> ()
                              n930 = Equal?(x=w1522, y="") -> (x = y?=w1524:bool)
                              n931 = case shown="True" w1524 {
                                frame False {
                                }
                                frame True {
                                n932 = local read "I compliance sweep"() -> (w1530:dbl)
                                n933 = local read "sweep delay ms"() -> (w1529:dbl)
                                n934 = local read "Sweep Direction (Keysight)"() -> (w1534:i32)
                                n935 = local read "points"() -> (w1531:u16)
                                n936 = local read "V end"() -> (w1532:dbl)
                                n937 = local read "V start"() -> (w1533:dbl)
                                n938 = call "pho_DB_Insert_LIV_meas_recipe.vi"("V start"=w1533, "Sweep Direction (Keysight)"=w1534, "V end"=w1532, "points"=w1531, "I compliance sweep"=w1530, "sweep delay ms"=w1529) -> ("RecipeID"=w1528:string)  [unwired: 9 in]
                                n939 = local write "RecipeID"(w1528) -> ()
                                }
                              }
                            }
                            frame #8 {
                              n940 = local read "V fine"() -> (w1548:dbl[])
                              n941 = local read "I fine"() -> (w1549:dbl[])
                              n942 = Get Date/Time String(seconds (now)=w1545, want seconds? (F)=TRUE) -> (date string=w1544:string, time string=w1542:string)  [unwired: 1 in]
                              n943 = local read "Operator"() -> (w1535:string)
                              n944 = local read "Parameters Flash"() -> (w1546:T4)
                              n945 = Build Array(w1548, w1549) -> (w1547:dbl[][])
                              n946 = call <vilib>:"Space Constant.vi"() -> ("String"=w1541:string)
                              n947 = local read "RecipeID"() -> (w1536:string)
                              n948 = Concatenate Strings(w1544, w1541, w1542) -> (w1540:string)
                              n949 = local read "Temp Data"() -> (w1539:T1)
                              n950 = local read "Mask"() -> (w1550:string)
                              n951 = call "WriteFlashFile NEW.vi"("Input File Path"=w1551, "IV array"=w1547, "Parameters"=w1546, "RecipeID"=w1536, "User"=w1535, "Coords"=w1538, "Wafer Info"="Wafer Info 3", "Mask Name"=w1550, "Temp Data"=w1539, "Die Number"=w1540) -> ()  [unwired: 17 in, 1 out]
                            }
                          }
                          n952 = Increment(x=w1398) -> (x+1=w1378:i32)
                          n953 = local write "Current Device"(w1378) -> ()
                          n954 = Divide(x=w1378, y=w1397) -> (x/y=w1396:dbl)
                          n955 = Number To Decimal String(number=w1378) -> (decimal integer string=w1383:string)  [unwired: 1 in]
                          n956 = Concatenate Strings("IV test for die number: " ("string"), w1383) -> (w1382:string)
                          n957 = Multiply(x=100.0, y=w1396) -> (x*y=w1394:dbl)
                          n958 = local write "Status"(w1382) -> ()
                          n959 = To Unsigned Byte Integer(number=w1394) -> (unsigned 8bit integer=w1393:u8)
                          n960 = local write "Progress 2"(w1393) -> ()
                        }
                      }
                      frame #2 {
                        w1556 = -1 ("x")
                        n961 = local read "Prober GPIB"() -> (w1560:string)
                        n962 = local read "current y"() -> (w1557:i32)
                        n963 = local read "current x"() -> (w1558:i32)
                        n964 = Multiply(x=w1557, y=w1556) -> (x*y=w1554:i32)
                        n965 = Multiply(x=w1556, y=w1558) -> (x*y=w1555:i32)
                        n966 = call "EG2001 Move Z Down.vi"("GPIB Address"=w1560) -> ("Error Out"=w1559:errorcluster, "GPIB Address Out"=w1561:string)  [unwired: 9 in]
                        n967 = call "EG2001 Move Machine Step X-Y.vi"("Flip X Coordinates?"=FALSE, "Y"=w1554, "Steps/Microns"=enum32{"Steps", "Microns"}."Microns", "X"=w1555, "error in (no error)"=w1559, "GPIB Address"=w1561) -> ()  [unwired: 4 in, 2 out]
                      }
                      frame #3 {
                        w1562 = 0 ("current x")
                        n968 = local write "current y"(w1562) -> ()
                        n969 = local write "current x"(w1562) -> ()
                      }
                    }
                  }
                }
              }
              frame #1 {
                n970 = local write "no file"(FALSE ("no file")) -> ()
              }
            }
            n971 = Enqueue Element At Opposite End(queue=w1340, element="idle", error in (no error)=w1341) -> (queue out=w1342:refnum<queue>, error out=w1343:errorcluster)  [unwired: 1 in, 1 out]
          }
          frame "update temperature" {
            # "Temptronics is communicatied via VISA sreial commands. RS sets the temperature, and ST tells the TEC to set the current temperature on the output pins to be read"
            n972 = local read "Temp Setpoint"() -> (w1571:string)
            n973 = local read "Temptronics VISA"() -> (w1569:refnum<visa-resource-name>)
            n974 = Concatenate Strings("rs" ("string"), w1571) -> (w1570:string)
            n975 = VISA Write(VISA resource name=w1569, write buffer=w1570) -> (VISA resource name out=w1568:refnum<visa-resource-name>)  [unwired: 1 in, 2 out]
            n976 = VISA Write(VISA resource name=w1568, write buffer="st") -> (VISA resource name out=w1566:refnum<visa-resource-name>, return count=w1565:u32)  [unwired: 1 in, 1 out]
            n977 = VISA Read(VISA resource name=w1566, byte count=w1565) -> (read buffer=w1564:string)  [unwired: 1 in, 3 out]
            n978 = local write "Current Temp"(w1564) -> ()
          }
          frame "Update Laser" {
            # "Sets the laser current to the values set in the Laser Current (mA) box. Then uses the calibration file to find the appropriate power and updates that. Finally updates the compliance for the sweeps so illuminated IV curves don't just hit compliance due to photogenerated current"
            n979 = flat-sequence {
              frame #0 {
                n980 = local read "TL4000 In"() -> (w1581:refnum<visa-resource-name>)
                n981 = local read "Laser Current (mA)"() -> (w1578:dbl)
                n982 = Divide(x=w1578, y=1000.0) -> (x/y=w1593:dbl)
                n983 = call <instrlib>:"TL4000 Set Laser Diode Current Setpoint.vi"("Laser Diode Current Setpoint (0.0)"=w1593, "instrument handle"=w1581) -> ()  [unwired: 8 in, 2 out]
                n984 = call-poly <vilib>:"Read From Spreadsheet File.vi"("delimiter (\\t)"="," ("delimiter (\\t)"), "file path (dialog if empty)"="Load Calibration File") -> ("all rows"=w1588:dbl[][])  [unwired: 5 in, 4 out]
                n985 = Index Array(array=w1588, index (row)=0) -> (element=w1590:dbl[])  [unwired: 1 in]
                n986 = Index Array(array=w1588, index (row)=1) -> (element=w1580:dbl[])  [unwired: 1 in]
                n987 = Array Size(array=w1580) -> (size(s)=w1579:i32)
                n988 = call "Convert to Dynamic Data2"("Array"=w1580) -> ("Dynamic Data Type"=w1592:dynamicdata)  [unwired: 3 in]
                n989 = call "Convert to Dynamic Data"("Array"=w1590) -> ("Dynamic Data Type"=w1591:dynamicdata)  [unwired: 3 in]
                n990 = for {
                  N: w1579 -> [_]
                  tunnel: w1590 -> [w1598] mode=indexing
                  tunnel: w1578 -> [w1599]
                  tunnel: w1580 -> [w1597]
                  tunnel: [w1595] -> w1585
                  i -> [w1596]
                  stop <- w1594 stop-if-true
                  n991 = Equal?(x=w1598, y=w1599) -> (x = y?=w1594:bool)
                  n992 = case shown="False" w1594 {
                    tunnel: w1597 -> [_ w1602]
                    tunnel: w1596 -> [_ w1601]
                    tunnel: [_ w1600] -> w1595
                    frame False {
                    }
                    frame True {
                      n993 = Index Array(array=w1602, index=w1601) -> (element=w1600:dbl)
                    }
                  }
                }
                "Output Power (mW)" <- w1585
                n994 = call "Build XY Graph"("Y Input"=w1592, "X Input"=w1591) -> ("XY Graph"=→"Calibration":cluster{"Y":dbl[], "Y":dbl[]}[])  [unwired: 3 in, 6 out]
              }
              frame #1 {
                n995 = case shown="True" "Auto Adjust Compliance?" {
                  frame False {
                  }
                  frame True {
                    n996 = local read "Output Power (mW)"() -> (w1606:dbl)
                    n997 = Greater Or Equal?(x=w1606, y=0.1) -> (x >= y?=w1604:bool)
                    n998 = case shown="False" w1604 {
                      frame False {
                        n999 = local write "I compliance sweep"(0.001 ("I compliance sweep")) -> ()
                      }
                      frame True {
                        n1000 = local read "Output Power (mW)"() -> (w1610:dbl)
                        n1001 = Multiply(x=w1610, y=0.001) -> (x*y=w1608:dbl)
                        n1002 = local write "I compliance sweep"(w1608) -> ()
                      }
                    }
                  }
                }
              }
            }
          }
          frame "Zero Laser" {
            # "Does not actually update laser - just changer the laser current variable to zero."
            n1003 = local write "Laser Current (mA)"(0.0) -> ()
          }
          frame "raw mask updated" {
            # "Asks if the manual mask should be updated to match the new raw mask file"
            n1004 = Enqueue Element At Opposite End(queue=w1622, element="idle", error in (no error)=w1621) -> (queue out=w1624:refnum<queue>, error out=w1623:errorcluster)  [unwired: 1 in, 1 out]
            n1005 = Two Button Dialog(message="Wold you like to update the Manual mask?", 1:"No" ("F button name (\"Cancel\")"), 2:"Yes" ("T button name (\"OK\")")) -> (T button?=w1615:bool)
            n1006 = case shown="True" w1615 {
              frame False {
              }
              frame True {
                n1007 = local read "Mask File Raw"() -> (w1625:path)
                n1008 = local write "Mask File Manual"(w1625) -> ()
              }
            }
          }
          frame "mask manual update" {
            # "asks if the raw test mask should be changed to math manual mask"
            n1009 = Enqueue Element At Opposite End(queue=w1633, element="idle", error in (no error)=w1632) -> (queue out=w1635:refnum<queue>, error out=w1634:errorcluster)  [unwired: 1 in, 1 out]
            n1010 = Two Button Dialog(message="Would you like update mask file for raw test?", 1:"No" ("F button name (\"Cancel\")"), 2:"Yes" ("T button name (\"OK\")")) -> (T button?=w1626:bool)
            n1011 = case shown="True" w1626 {
              frame False {
              }
              frame True {
                n1012 = local read "Mask File Manual"() -> (w1636:path)
                n1013 = local write "Mask File Raw"(w1636) -> ()
              }
            }
          }
          frame "save comment" {
            # "Uses activex to open the measurement log, save the comment to the approprate cell, and attempt to close the file again. As it stands, the file always stays open after this is run."
            n1014 = flat-sequence {
              frame #0 {
                w1645 = "C:\\Users\\Flash\\Desktop\\Data\\Detector test data\\MeasurementLog.csv"
                # "6"
                # "5"
                # "4"
                # "3"
                # "2"
                # "1"
                # "This example demonstrates how to close a Worksheet from an Excel Workbook. \n\nThe steps are as follows:\n1) Open Excel\n2) Open the specific workbook\n3) Open a Specific Sheet\n4) Find a range in that sheet to clear \n5) For adding individual data points, you can use the same range refnum to send in coordinates and the new values. \n6) Close all open references"
                n1015 = Automation Open(Automation Refnum=refnum<k7> refnum ("Excel._Application")) -> (Automation Refnum=w1686:refnum<k7>, error out=w1685:errorcluster)  [unwired: 3 in]
                n1016 = property on="Property Node" class="_Application"(reference=w1686, error in=w1685, "Visible"=TRUE) -> (reference out=w1682:refnum<k7>, error out=w1681:errorcluster, "Workbooks"=w1683:refnum<k7>)
                n1017 = invoke on="Invoke Node" class="Workbooks" method="Open"(reference=w1683, error in=w1681, "Filename"=w1645, "ReadOnly"=FALSE, "Editable"=TRUE) -> (error out=w1680:errorcluster, "Open"=w1651:refnum<k7>)  [unwired: 13 in, 16 out]
                n1018 = property on="Property Node" class="_Workbook"(reference=w1651, error in=w1680) -> (reference out=w1648:refnum<k7>, error out=w1679:errorcluster, "Worksheets"=w1674:refnum<k7>)
                n1019 = invoke on="Invoke Node" class="Sheets" method="Item"(reference=w1674, error in=w1679, "Index"="MeasurementLog") -> (reference out=w1668:refnum<k7>, error out=w1673:errorcluster, "Item"=w1676:variant)  [unwired: 1 in, 1 out]
                n1020 = local read "Logview"() -> (w1687:i32)
                n1021 = Variant To Data(error in=w1673, type=refnum<k7> refnum ("reference"), Variant=w1676) -> (data=w1646:refnum<k7>, error out=w1661:errorcluster)
                n1022 = Build Array(w1687) -> (w1657:i32[])
                n1023 = To Variant(anything="A1") -> (Variant=w1669:variant)
                n1024 = To Variant(anything="A1") -> (Variant=w1670:variant)
                n1025 = local read "Add Comments"() -> (w1658:string)
                n1026 = invoke on="Invoke Node" class="_Worksheet" method="Range"(reference=w1646, error in=w1661, "Cell1"=w1669, "Cell2"=w1670) -> (error out=w1660:errorcluster, "Range"=w1663:refnum<k7>)  [unwired: 1 in, 3 out]
                n1027 = Index Array(array=w1657, index=0) -> (element=w1654:i32)
                n1028 = Add(x=w1654, y=1) -> (x+y=w1652:i32)
                n1029 = invoke on="Invoke Node" class="Range" method="ListNames"(reference=w1663, error in=w1660) -> (reference out=w1662:refnum<k7>, error out=w1659:errorcluster)  [unwired: 1 in, 1 out]
                n1030 = To Variant(anything=w1658) -> (Variant=w1666:variant)
                n1031 = invoke on="Invoke Node" class="Range" method="Item"(reference=w1662, error in=w1659, "RowIndex"=w1652, "ColumnIndex"=7, "newValue"=w1666) -> (reference out=w1664:refnum<k7>, error out=w1647:errorcluster)  [unwired: 1 in, 4 out]
                n1032 = invoke class="_Worksheet" method="SaveAs"(reference=w1646, error in=w1647, "Filename"=w1645) -> (reference out=w1642:refnum<k7>, error out=w1641:errorcluster)  [unwired: 10 in, 11 out]
                n1033 = Close Reference(reference=w1664, error in (no error)=w1641) -> (error out=w1675:errorcluster)
                n1034 = Close Reference(reference=w1668, error in (no error)=w1675) -> (error out=w1649:errorcluster)
                n1035 = Close Reference(reference=w1648, error in (no error)=w1649) -> (error out=w1650:errorcluster)
                n1036 = Close Reference(reference=w1682, error in (no error)=w1650) -> (error out=w1644:errorcluster)
                n1037 = Close Reference(reference=w1642, error in (no error)=w1644) -> (error out=w1643:errorcluster)
                n1038 = call <vilib>:"Simple Error Handler.vi"("error in (no error)"=w1643) -> ()  [unwired: 4 in, 5 out]
              }
            }
          }
          frame "update viewer" {
            # "Makes the logview table match the measurements log csv"
            n1039 = call-poly <vilib>:"Read From Spreadsheet File.vi"("file path (dialog if empty)"=path "C:/Users/Flash/Desktop/Data/Detector test data/MeasurementLog.csv") -> ("all rows"=w1691:string[][])  [unwired: 6 in, 4 out]
            n1040 = property on="Logview" class="MCListbox (strict)"("ItemNames"=w1691) -> ()  [unwired: 2 in, 2 out]
          }
          frame "refresh device names" {
            # "Ideally populates device nam elist for auto test with devices from the appropriate mask file. Isnt woking at this time, the user needs to manually type in device names"
            n1041 = Enqueue Element At Opposite End(queue=w1703, element="idle", error in (no error)=w1702) -> (queue out=w1704:refnum<queue>, error out=w1698:errorcluster)  [unwired: 1 in, 1 out]
            n1042 = call "getDB unique Device.vi"("error in (no error)"=w1698, "Mask"="Mask Name") -> ("NameList"=w1694:string[])  [unwired: 8 in, 1 out]
            "NameList" <- w1694
            n1043 = Equal?(x=w1694, y=string[] []) -> (x = y?=w1696:bool[])
            n1044 = And Array Elements(Boolean array=w1696) -> (logical AND=w1695:bool)
            n1045 = case shown="True" w1695 {
              tunnel: w1694 -> [w1705 w1707]
              tunnel: [w1705 w1706] -> w1693
              frame False {
              }
              frame True {
                n1046 = call "Prompt User for Input"() -> ("YES"=w1708:bool)  [unwired: 18 in, 1 out]
                n1047 = case shown="True" w1708 {
                  tunnel: w1707 -> [w1709 _]
                  tunnel: [w1709 w1710] -> w1706
                  frame False {
                  }
                  frame True {
                    # "GET DEVICES FROM FILE"
                    n1048 = local read "Mask File all"() -> (w1711:path)
                    n1049 = call "Select unique devices from File.vi"("MaskFile"=w1711) -> ("Device Array"=w1710:string[])  [unwired: 10 in]
                  }
                }
              }
            }
            n1050 = property on="Available Device Name" class="CmbBox"("Strings[]"=w1693) -> ()  [unwired: 2 in, 2 out]
          }
          frame "add to list" {
            # "Adds available device name to test list. If Skip Raw Test Is selected, it appends (skip) on the device name, which the auto test uses to know when to skip the raw test."
            n1051 = Enqueue Element At Opposite End(queue=w1716, element="idle", error in (no error)=w1714) -> (queue out=w1718:refnum<queue>, error out=w1717:errorcluster)  [unwired: 1 in, 1 out]
            n1052 = case shown="False" "Skip Raw Test?" {
              frame False {
                n1053 = property on="Test List" class="LstBox (strict)"() -> ("Item Names"=w1719:string[])  [unwired: 2 in, 2 out]
                n1054 = local read "Available Device Name"() -> (w1720:string)
                n1055 = Build Array (concatenate)(w1719, w1720) -> (w1721:string[])
                n1056 = property on="Test List" class="LstBox (strict)"("Item Names"=w1721) -> ()  [unwired: 2 in, 2 out]
              }
              frame True {
                n1057 = property on="Test List" class="LstBox (strict)"() -> ("Item Names"=w1725:string[])  [unwired: 2 in, 2 out]
                n1058 = local read "Available Device Name"() -> (w1724:string)
                n1059 = Concatenate Strings(w1724, "(skip)" ("string")) -> (w1722:string)
                n1060 = Build Array (concatenate)(w1725, w1722) -> (w1726:string[])
                n1061 = property on="Test List" class="LstBox (strict)"("Item Names"=w1726) -> ()  [unwired: 2 in, 2 out]
              }
            }
          }
          frame "skip raw?" {
            # "First checks to see of (skip) is appended on the current device name. If it isnt, it sets \"raw test skipped\" to false. It (skip) is appended on the end, then it removes it and sets \"raw test skipped\" to true."
            n1062 = property on="Test List" class="LstBox (strict)"() -> ("Item Names"=w1736:string[])  [unwired: 2 in, 2 out]
            n1063 = local read "Counter"() -> (w1735:i32)
            n1064 = Index Array(array=w1736, index=w1735) -> (element=w1734:string)
            "device name w skip" <- w1734
            n1065 = Search/Split String(string=w1734, search string/char (-)="(skip)") -> (match + rest of string=w1732:string)  [unwired: 1 in, 2 out]
            n1066 = Equal?(x=w1732, y="") -> (x = y?=w1730:bool)
            n1067 = local write "no file"(FALSE ("no file")) -> ()
            n1068 = Not(x=w1730) -> (.not. x?=w1729:bool)
            n1069 = case shown="False" w1729 {
              frame False {
                n1070 = local write "Raw Test Skipped"(FALSE ("Skipped")) -> ()
              }
              frame True {
                n1071 = flat-sequence {
                  tunnel: [w1745] -> w1742
                  tunnel: [w1744] -> w1741
                  tunnel: [w1743] -> w1740
                  tunnel: w1742 -> [w1753]
                  tunnel: w1741 -> [w1752]
                  tunnel: w1740 -> [w1751]
                  frame #0 {
                    n1072 = local read "Counter"() -> (w1744:i32)
                    n1073 = property on="Test List" class="LstBox (strict)"() -> ("Item Names"=w1745:string[])  [unwired: 2 in, 2 out]
                    n1074 = Index Array(array=w1745, index=w1744) -> (element=w1747:string)
                    n1075 = Search/Split String(string=w1747, search string/char (-)="(skip)") -> (substring before match=w1743:string)  [unwired: 1 in, 2 out]
                  }
                  frame #1 {
                    n1076 = Delete From Array(array=w1753, index=w1752) -> (array with subset deleted=w1750:string[])  [unwired: 1 in, 1 out]
                    n1077 = Insert Into Array(array=w1750, index=w1752, new element=w1751) -> (w1749:string[])
                    n1078 = property on="Test List" class="LstBox (strict)"("Item Names"=w1749) -> ()  [unwired: 2 in, 2 out]
                    "Raw Test Skipped" <- TRUE ("Skipped")
                  }
                }
              }
            }
          }
          frame "add to laser list" {
            # "Adds \"desired current\" value to current list"
            n1079 = property on="Laser List" class="LstBox (strict)"() -> ("Item Names"=w1758:string[])  [unwired: 2 in, 2 out]
            n1080 = local read "Desired Current (mA)"() -> (w1755:dbl)
            n1081 = Format Into String(format string="%08.4f", w1755) -> (resulting string=w1754:string)  [unwired: 2 in, 1 out]
            n1082 = Build Array (concatenate)(w1758, w1754) -> (w1757:string[])
            n1083 = property on="Laser List" class="LstBox (strict)"("Item Names"=w1757) -> ()  [unwired: 2 in, 2 out]
          }
          frame "remove from laser list" {
            # "removes highlighted value from laser list"
            n1084 = local read "Laser List"() -> (w1767:i32)
            n1085 = property on="Laser List" class="LstBox (strict)"() -> ("Item Names"=w1766:string[])  [unwired: 2 in, 2 out]
            n1086 = Delete From Array(array=w1766, index=w1767) -> (array with subset deleted=w1765:string[])  [unwired: 1 in, 1 out]
            n1087 = property on="Laser List" class="LstBox (strict)"("Item Names"=w1765) -> ()  [unwired: 2 in, 2 out]
          }
          frame "clear laser list" {
            # "removes all values from laser list"
            n1088 = property on="Laser List" class="LstBox (strict)"("Item Names"=string[] []) -> ()  [unwired: 2 in, 2 out]
          }
          frame "remove from list" {
            # "removes highlighted value from test list"
            n1089 = property on="Test List" class="LstBox (strict)"() -> ("Item Names"=w1774:string[])  [unwired: 2 in, 2 out]
            n1090 = local read "Test List"() -> (w1772:i32)
            n1091 = Enqueue Element At Opposite End(queue=w1776, element="idle", error in (no error)=w1775) -> (queue out=w1778:refnum<queue>, error out=w1777:errorcluster)  [unwired: 1 in, 1 out]
            n1092 = Delete From Array(array=w1774, index=w1772) -> (array with subset deleted=w1773:string[])  [unwired: 1 in, 1 out]
            n1093 = property on="Test List" class="LstBox (strict)"("Item Names"=w1773) -> ()  [unwired: 2 in, 2 out]
          }
          frame "clear list" {
            # "removes all values from test list"
            n1094 = property on="Test List" class="LstBox (strict)"("Item Names"=string[] []) -> ()  [unwired: 2 in, 2 out]
            n1095 = Enqueue Element(queue=w1785, element="idle", error in (no error)=w1783) -> (queue out=w1787:refnum<queue>, error out=w1786:errorcluster)  [unwired: 1 in, 1 out]
          }
          frame "add to temp list" {
            # "Adds \"desired temperature\" valiue to temp list"
            n1096 = local read "Desired Temperature"() -> (w1791:dbl)
            n1097 = property on="Single Device Temperature List" class="LstBox (strict)"() -> ("Item Names"=w1790:string[])  [unwired: 2 in, 2 out]
            n1098 = Format Into String(format string="%08.4f", w1791) -> (resulting string=w1789:string)  [unwired: 2 in, 1 out]
            n1099 = Build Array (concatenate)(w1790, w1789) -> (w1788:string[])
            n1100 = property on="Single Device Temperature List" class="LstBox (strict)"("Item Names"=w1788) -> ()  [unwired: 2 in, 2 out]
          }
          frame "remove from temp list" {
            # "Removes highlighted value from temperatre list"
            n1101 = property on="Single Device Temperature List" class="LstBox (strict)"() -> ("Item Names"=w1797:string[])  [unwired: 2 in, 2 out]
            n1102 = local read "Single Device Temperature List"() -> (w1796:i32)
            n1103 = Delete From Array(array=w1797, index=w1796) -> (array with subset deleted=w1795:string[])  [unwired: 1 in, 1 out]
            n1104 = property on="Single Device Temperature List" class="LstBox (strict)"("Item Names"=w1795) -> ()  [unwired: 2 in, 2 out]
          }
          frame "clear temp list" {
            # "Removes all values from temp list"
            n1105 = property on="Single Device Temperature List" class="LstBox (strict)"("Item Names"=string[] []) -> ()  [unwired: 2 in, 2 out]
          }
          frame "pick device" {
            # "Takes the device for the current iteration of the auto test and updates the test name. The Counter keeps track of which iteration of the auto test the program is running. After the device name is updated, the counter is incremented by one. If th elast device is reached, the counter is reset to zero for the next test."
            n1106 = Enqueue Element(queue=w1808, element="idle", error in (no error)=w1806) -> (queue out=w1807:refnum<queue>, error out=w1805:errorcluster)  [unwired: 1 in, 1 out]
            n1107 = flat-sequence {
              frame #0 {
                n1108 = local read "Mask File all"() -> (w1811:path)
                n1109 = property on="Test List" class="LstBox (strict)"() -> ("Item Names"=w1813:string[])  [unwired: 2 in, 2 out]
                n1110 = local read "Counter"() -> (w1812:i32)
                n1111 = Index Array(array=w1813, index=w1812) -> (element=w1809:string)
                n1112 = local write "Device Name"(w1809) -> ()
                n1113 = call "Mask file select device.vi"("Device"=w1809, "MaskFile"=w1811) -> ("RawMask"=w1810:path)  [unwired: 9 in]
                n1114 = local write "Mask File Raw"(w1810) -> ()
              }
              frame #1 {
                n1115 = local read "Counter"() -> (w1815:i32)
                n1116 = Increment(x=w1815) -> (x+1=w1814:i32)
                n1117 = local write "Counter"(w1814) -> ()
              }
              frame #2 {
                n1118 = property on="Test List" class="LstBox (strict)"() -> ("Item Names"=w1818:string[])  [unwired: 2 in, 2 out]
                n1119 = local read "Counter"() -> (w1819:i32)
                n1120 = Array Size(array=w1818) -> (size(s)=w1817:i32)
                n1121 = Equal?(x=w1819, y=w1817) -> (x = y?=w1816:bool)
                n1122 = case shown="False" w1816 {
                  frame False {
                  }
                  frame True {
                    n1123 = local write "Counter"(0 ("Counter")) -> ()
                  }
                }
              }
            }
          }
          frame "pick laser" {
            # "See pick device. Mechanics are exactly the same, except for laser instead of device name"
            n1124 = flat-sequence {
              frame #0 {
                n1125 = property on="Laser List" class="LstBox (strict)"() -> ("Item Names"=w1826:string[])  [unwired: 2 in, 2 out]
                n1126 = local read "Laser Counter"() -> (w1827:i32)
                n1127 = Index Array(array=w1826, index=w1827) -> (element=w1825:string)
                n1128 = Fract/Exp String To Number(string=w1825) -> (number=w1824:dbl)  [unwired: 3 in, 1 out]
                n1129 = local write "Laser Current (mA)"(w1824) -> ()
              }
              frame #1 {
                n1130 = local read "Laser Counter"() -> (w1829:i32)
                n1131 = Increment(x=w1829) -> (x+1=w1828:i32)
                n1132 = local write "Laser Counter"(w1828) -> ()
              }
              frame #2 {
                n1133 = property on="Laser List" class="LstBox (strict)"() -> ("Item Names"=w1830:string[])  [unwired: 2 in, 2 out]
                n1134 = local read "Laser Counter"() -> (w1833:i32)
                n1135 = Array Size(array=w1830) -> (size(s)=w1832:i32)
                n1136 = Equal?(x=w1833, y=w1832) -> (x = y?=w1831:bool)
                n1137 = case shown="True" w1831 {
                  frame False {
                  }
                  frame True {
                    n1138 = local write "Laser Counter"(0 ("Counter")) -> ()
                  }
                }
              }
            }
          }
          frame "reset skip" {
            # "If the raw test was skipped, during the auto test the (skip) tag was removed from the device mane during testing. This replaces the (skip)tag so the user can run another test"
            n1139 = local read "Counter"() -> (w1837:i32)
            n1140 = property on="Test List" class="LstBox (strict)"() -> ("Item Names"=w1839:string[])  [unwired: 2 in, 2 out]
            n1141 = Not Equal?(x=w1837, y=0) -> (x != y?=w1835:bool)
            n1142 = case shown="False" w1835 {
              tunnel: w1839 -> [w1845 w1854]
              tunnel: [w1846 w1850] -> w1838
              frame False {
                n1143 = Array Size(array=w1845) -> (size(s)=w1844:i32)
                n1144 = Decrement(x=w1844) -> (x-1=w1843:i32)
                n1145 = Delete From Array(array=w1845, index=w1843) -> (array with subset deleted=w1847:string[])  [unwired: 1 in, 1 out]
                n1146 = local read "device name w skip"() -> (w1848:string)
                n1147 = Insert Into Array(array=w1847, index=w1843, new element=w1848) -> (w1846:string[])
              }
              frame True {
                n1148 = local read "Counter"() -> (w1851:i32)
                n1149 = Subtract(x=w1851, y=1) -> (x-y=w1849:i32)
                n1150 = Delete From Array(array=w1854, index=w1849) -> (array with subset deleted=w1852:string[])  [unwired: 1 in, 1 out]
                n1151 = local read "device name w skip"() -> (w1853:string)
                n1152 = Insert Into Array(array=w1852, index=w1849, new element=w1853) -> (w1850:string[])
              }
            }
            n1153 = property on="Test List" class="LstBox (strict)"("Item Names"=w1838) -> ()  [unwired: 2 in, 2 out]
          }
          frame "load wafer" {
            # "tells probe station to load wafer"
            n1154 = flat-sequence {
              frame #0 {
                n1155 = local read "Prober GPIB"() -> (w1862:string)
                n1156 = call "EG2001 Load Wafer.vi"("Enable Error Message"=FALSE, "error in (no error)"=errorcluster {"status"=FALSE, "code"=0, "source"=""}, "Characters to Write"="LO", "GPIB Address"=w1862) -> ()  [unwired: 5 in, 3 out]
                n1157 = local write "Status"("loading..." ("Status")) -> ()
              }
              frame #1 {
                n1158 = local write "Status"("load complete" ("Status")) -> ()
              }
            }
          }
          frame "profile z" {
            # "tells pobe station to run \"profile z\" program"
            n1159 = local read "Prober GPIB"() -> (w1865:string)
            n1160 = call "EG2001 Profile Wafer Only.vi"("GPIB Address"=w1865) -> ("Error Out"=→"Error Out":errorcluster)  [unwired: 9 in, 1 out]
          }
          frame "auto align" {
            # "tells prober to run \"auto align\" feature. Only works if ref is already stored, if find target needs to be run, that needs to be done manually, (see prober guide for details)."
            n1161 = flat-sequence {
              frame #0 {
                n1162 = local read "Prober GPIB"() -> (w1871:string)
                n1163 = local write "Status"("aligning" ("Status")) -> ()
                n1164 = call "EG2001 Auto Align Wafer.vi"("GPIB Address"=w1871) -> ()  [unwired: 8 in, 3 out]
              }
              frame #1 {
                n1165 = local write "Status"("idle" ("Status")) -> ()
              }
            }
          }
          frame "wait" {
            # "delays for a certain number of seconds, determined by the \"wait after load\" parameter"
            n1166 = Multiply(x="Wait after load", y=u32 1000) -> (x*y=w1873:u32)
            n1167 = Wait (ms)(milliseconds to wait=w1873) -> ()  [unwired: 1 out]
          }
          frame "add to wafer list" {
            # "adds \"desired wafer name\" to wafer list"
            n1168 = property on="Wafer List" class="LstBox (strict)"() -> ("Item Names"=w1879:string[])  [unwired: 2 in, 2 out]
            n1169 = local read "Desired Wafer Name"() -> (w1880:string)
            n1170 = Build Array (concatenate)(w1879, w1880) -> (w1878:string[])
            n1171 = property on="Wafer List" class="LstBox (strict)"("Item Names"=w1878) -> ()  [unwired: 2 in, 2 out]
          }
          frame "remove from wafer list" {
            # "Removes highlighted value from wafer list"
            n1172 = property on="Wafer List" class="LstBox (strict)"() -> ("Item Names"=w1884:string[])  [unwired: 2 in, 2 out]
            n1173 = local read "Wafer List"() -> (w1885:i32)
            n1174 = Delete From Array(array=w1884, index=w1885) -> (array with subset deleted=w1883:string[])  [unwired: 1 in, 1 out]
            n1175 = property on="Wafer List" class="LstBox (strict)"("Item Names"=w1883) -> ()  [unwired: 2 in, 2 out]
          }
          frame "clear wafer list" {
            # "Deletes all values in wafer list"
            n1176 = property on="Wafer List" class="LstBox (strict)"("Item Names"=string[] []) -> ()  [unwired: 2 in, 2 out]
          }
          frame "desired device change" {
            # "works the same as \"die number changed\" but in the temperature tab"
            n1177 = local write "Status"("Changing Die" ("Status")) -> ()
            n1178 = flat-sequence {
              frame #0 {
                n1179 = local read "Desired Device"() -> (w1900:u16)
                n1180 = local read "Array of Cell Data Clusters"() -> (w1901:T12)
                n1181 = Index Array(array=w1901, index=w1900) -> (element=w1899:T17)
                n1182 = Unbundle By Name(w1899) -> ("Cell Name"=w1898:string, "X-coord"=w1895:dbl, "Y-coord"=w1894:dbl, "Area"=w1897:dbl, "Meas Area"=w1896:dbl)
                "X" <- w1895
                "Y" <- w1894
                n1183 = local write "Device Name"(w1898) -> ()
                n1184 = local write "x target"(w1895) -> ()
                n1185 = local write "y target"(w1894) -> ()
                n1186 = local write "ActiveArea_um2"(w1897) -> ()
                n1187 = local write "MesaArea_um2"(w1896) -> ()
              }
              frame #1 {
                n1188 = local read "J set A/cm2"() -> (w1907:dbl)
                n1189 = local read "Laser Current (mA)"() -> (w1904:dbl)
                n1190 = Equal To 0?(x=w1904) -> (x = 0?=w1903:bool)
                n1191 = case shown="True" w1903 {
                  tunnel: [w1909 w1910] -> w1902
                  frame False {
                    n1192 = local read "ActiveArea_um2"() -> (w1909:dbl)
                  }
                  frame True {
                    n1193 = local read "MesaArea_um2"() -> (w1910:dbl)
                  }
                }
                n1194 = Divide(x=w1902, y=100000000.0) -> (x/y=w1906:dbl)
                n1195 = Multiply(x=w1906, y=w1907) -> (x*y=w1908:dbl)
                n1196 = local write "I set"(w1908) -> ()
              }
            }
          }
          frame "select temperature" {
            # "Updates the current temperature from the temperature list, and updates the counter, which operates the same as laser, wafer, and auto test counters"
            n1197 = flat-sequence {
              frame #0 {
                n1198 = property on="Auto Temperature List" class="LstBox (strict)"() -> ("Item Names"=w1913:string[])  [unwired: 2 in, 2 out]
                n1199 = local read "Auto Temp Counter"() -> (w1916:i32)
                n1200 = Index Array(array=w1913, index=w1916) -> (element=w1914:string)
                n1201 = local write "Status"("selecting temperature" ("Status")) -> ()
                n1202 = local write "Temp Setpoint"(w1914) -> ()
              }
              frame #1 {
                n1203 = local read "Auto Temp Counter"() -> (w1918:i32)
                n1204 = Increment(x=w1918) -> (x+1=w1917:i32)
                n1205 = local write "Auto Temp Counter"(w1917) -> ()
              }
              frame #2 {
                n1206 = property on="Auto Temperature List" class="LstBox (strict)"() -> ("Item Names"=w1919:string[])  [unwired: 2 in, 2 out]
                n1207 = local read "Auto Temp Counter"() -> (w1922:i32)
                n1208 = Array Size(array=w1919) -> (size(s)=w1921:i32)
                n1209 = Equal?(x=w1922, y=w1921) -> (x = y?=w1920:bool)
                n1210 = case shown="True" w1920 {
                  frame False {
                  }
                  frame True {
                    n1211 = local write "Auto Temp Counter"(0 ("Counter")) -> ()
                  }
                }
              }
            }
          }
          frame "wait for temperature" {
            # "This while loop checks every five seconds whether the temperature has reached the setpoint, and if it has it exits the while loop and allows the program to continue"
            n1212 = while {
              i -> [w1929]
              stop <- w1926 stop-if-true
              n1213 = flat-sequence {
                tunnel: [w1935] -> w1928
                tunnel: w1929 -> [w1943]
                tunnel: [w1942] -> w1927
                frame #0 {
                  n1214 = local read "Temptronics VISA"() -> (w1939:refnum<visa-resource-name>)
                  n1215 = local read "Temp Setpoint"() -> (w1931:string)
                  n1216 = VISA Write(VISA resource name=w1939, write buffer="st") -> (VISA resource name out=w1938:refnum<visa-resource-name>, return count=w1937:u32)  [unwired: 1 in, 1 out]
                  n1217 = local write "Status"("waiting for temperature..." ("Status")) -> ()
                  n1218 = VISA Read(VISA resource name=w1938, byte count=w1937) -> (read buffer=w1933:string)  [unwired: 1 in, 3 out]
                  n1219 = Wait (ms)(milliseconds to wait=u32 500) -> ()  [unwired: 1 out]
                  n1220 = Decimal String To Number(string=w1931) -> (number=w1930:i32)  [unwired: 2 in, 1 out]
                  n1221 = Decimal String To Number(string=w1933) -> (number=w1932:i32)  [unwired: 2 in, 1 out]
                  n1222 = Equal?(x=w1932, y=w1930) -> (x = y?=w1935:bool)
                }
                frame #1 {
                  n1223 = Equal?(x=w1943, y=500) -> ()  [unwired: 1 out]
                  n1224 = case shown="False" FALSE {
                    tunnel: [_ w1945] -> w1942
                    frame False {
                    }
                    frame True {
                      n1225 = One Button Dialog(message="Temperature Timeout") -> (true=w1945:bool)  [unwired: 1 in]
                    }
                  }
                }
              }
              n1226 = Or(x=w1927, y=w1928) -> (x .or. y?=w1926:bool)
            }
          }
          frame "temp to 25" {
            n1227 = local write "Temp Setpoint"("25" ("Temp Setpoint")) -> ()
          }
          frame "load file for temp" {
            # "same as load manual mask file, but in the temperature tab"
            n1228 = flat-sequence {
              tunnel: [w1960] -> w1955
              tunnel: w1955 -> [w1963]
              frame #0 {
                n1229 = local read "Mask File Temperature"() -> (w1956:path)
                n1230 = local write "Status"("Loading mask file" ("Status")) -> ()
                n1231 = call "Device Files v1.vi"("Rows"=1200, "Mask file path"=w1956) -> ("Mask Name"=w1961:string, "size(s)"=w1960:i32, "Array of Cell Clusters"=w1957:T5)  [unwired: 6 in, 1 out]
                n1232 = local write "Mask"(w1961) -> ()
                n1233 = local write "Array of Cell Data Clusters"(w1957) -> ()
              }
              frame #1 {
                n1234 = for {
                  N: w1963 -> [_]
                  tunnel: [w1964] -> w1962 mode=indexing
                  i -> [w1965]
                  n1235 = Number To Decimal String(number=w1965) -> (decimal integer string=w1964:string)  [unwired: 1 in]
                }
                n1236 = property on="Desired Device" class="Ring (strict)"("Strings []"=w1962) -> ()  [unwired: 2 in, 2 out]
              }
              frame #2 {
                n1237 = local read "Desired Device"() -> (w1972:u16)
                n1238 = local read "Array of Cell Data Clusters"() -> (w1973:T12)
                n1239 = Index Array(array=w1973, index=w1972) -> (element=w1971:T17)
                n1240 = Unbundle By Name(w1971) -> ("Cell Name"=w1966:string, "X-coord"=w1969:dbl, "Y-coord"=w1970:dbl, "Area"=w1968:dbl, "Meas Area"=w1967:dbl)
                n1241 = local write "Device Name"(w1966) -> ()
                n1242 = local write "x target"(w1969) -> ()
                n1243 = local write "y target"(w1970) -> ()
                n1244 = local write "ActiveArea_um2"(w1968) -> ()
                n1245 = local write "MesaArea_um2"(w1967) -> ()
              }
              frame #3 {
                n1246 = local read "J set A/cm2"() -> (w1979:dbl)
                n1247 = local read "Laser Current (mA)"() -> (w1976:dbl)
                n1248 = Equal To 0?(x=w1976) -> (x = 0?=w1975:bool)
                n1249 = case shown="False" w1975 {
                  tunnel: [w1981 w1982] -> w1974
                  frame False {
                    n1250 = local read "ActiveArea_um2"() -> (w1981:dbl)
                  }
                  frame True {
                    n1251 = local read "MesaArea_um2"() -> (w1982:dbl)
                  }
                }
                n1252 = Divide(x=w1974, y=100000000.0) -> (x/y=w1978:dbl)
                n1253 = Multiply(x=w1978, y=w1979) -> (x*y=w1980:dbl)
                n1254 = local write "I set"(w1980) -> ()
              }
            }
            n1255 = Enqueue Element(queue=w1954, element="idle", error in (no error)=w1952) -> (queue out=w1953:refnum<queue>, error out=w1951:errorcluster)  [unwired: 1 in, 1 out]
          }
          frame "begin temperature series" {
            # "In Progress"
            n1256 = flat-sequence {
              frame #0 {
                n1257 = local read "Mask File Temperature"() -> (w1988:path)
                n1258 = local read "points"() -> (w1990:u16)
                n1259 = Initialize Array(nan ("element"), w1990) -> (w1992:dbl[])
                n1260 = local write "Mask File Temperature"(w1988) -> ()
                n1261 = local write "Tab Control"(T16."Temperature Series Single Device" ("Tab Control")) -> ()
                n1262 = call "Device Files v1.vi"("Rows"=1200, "Mask file path"=w1988) -> ("size(s)"=w1987:i32, "Array of Cell Clusters"=w1986:T5)  [unwired: 6 in, 2 out]
                n1263 = Bundle(w1992, w1992) -> (w1991:cluster{dbl[], dbl[]})  [unwired: 1 in]
                n1264 = Initialize Array(w1991, w1987) -> (w1985:cluster{dbl[], dbl[]}[])
                n1265 = local write "Fine Cell Clusters"(w1986) -> ()
                n1266 = local write "Total Device"(w1987) -> ()
                n1267 = local write "IV temp linear"(w1985) -> ()
                n1268 = local write "IV temp log"(w1985) -> ()
                n1269 = local write "Status"("prepare temperature test" ("Status")) -> ()
              }
              frame #1 {
                n1270 = property on="Single Device Temperature List" class="LstBox (strict)"() -> ("Item Names"=w1996:string[])  [unwired: 2 in, 2 out]
                n1271 = for {
                  tunnel: w1996 -> [_] mode=indexing
                  i -> [w1997]
                  n1272 = flat-sequence {
                    frame #0 {
                      n1273 = flat-sequence {
                        frame #0 {
                          n1274 = local read "TempCounter"() -> (w2001:i32)
                          n1275 = property on="Single Device Temperature List" class="LstBox (strict)"() -> ("Item Names"=w2000:string[])  [unwired: 2 in, 2 out]
                          n1276 = local write "Status"("selecting temperature" ("Status")) -> ()
                          n1277 = Index Array(array=w2000, index=w2001) -> (element=w1998:string)
                          n1278 = local write "Temp Setpoint"(w1998) -> ()
                        }
                        frame #1 {
                          n1279 = local read "TempCounter"() -> (w2003:i32)
                          n1280 = Increment(x=w2003) -> (x+1=w2002:i32)
                          n1281 = local write "TempCounter"(w2002) -> ()
                        }
                        frame #2 {
                          n1282 = property on="Single Device Temperature List" class="LstBox (strict)"() -> ("Item Names"=w2004:string[])  [unwired: 2 in, 2 out]
                          n1283 = local read "TempCounter"() -> (w2007:i32)
                          n1284 = Array Size(array=w2004) -> (size(s)=w2006:i32)
                          n1285 = Equal?(x=w2007, y=w2006) -> (x = y?=w2005:bool)
                          n1286 = case shown="False" w2005 {
                            frame False {
                            }
                            frame True {
                              n1287 = local write "TempCounter"(0 ("Counter")) -> ()
                            }
                          }
                        }
                      }
                    }
                    frame #1 {
                      n1288 = local read "Temp Setpoint"() -> (w2010:string)
                      n1289 = local read "Temptronics VISA"() -> (w2012:refnum<visa-resource-name>)
                      n1290 = Concatenate Strings("rs" ("string"), w2010) -> (w2011:string)
                      n1291 = VISA Write(VISA resource name=w2012, write buffer=w2011) -> (VISA resource name out=w2013:refnum<visa-resource-name>)  [unwired: 1 in, 2 out]
                      n1292 = VISA Write(VISA resource name=w2013, write buffer="st") -> (VISA resource name out=w2015:refnum<visa-resource-name>, return count=w2016:u32)  [unwired: 1 in, 1 out]
                      n1293 = VISA Read(VISA resource name=w2015, byte count=w2016) -> (read buffer=w2017:string)  [unwired: 1 in, 3 out]
                      n1294 = local write "Current Temp"(w2017) -> ()
                    }
                    frame #2 {
                      n1295 = while {
                        i -> [w2021]
                        stop <- w2018 stop-if-true
                        n1296 = flat-sequence {
                          tunnel: [w2027] -> w2020
                          tunnel: w2021 -> [w2034]
                          tunnel: [w2033] -> w2019
                          frame #0 {
                            n1297 = local read "Temptronics VISA"() -> (w2031:refnum<visa-resource-name>)
                            n1298 = Wait (ms)(milliseconds to wait=u32 500) -> ()  [unwired: 1 out]
                            n1299 = VISA Write(VISA resource name=w2031, write buffer="st") -> (VISA resource name out=w2030:refnum<visa-resource-name>, return count=w2029:u32)  [unwired: 1 in, 1 out]
                            n1300 = local read "Temp Setpoint"() -> (w2023:string)
                            n1301 = local write "Status"("waiting for temperature..." ("Status")) -> ()
                            n1302 = VISA Read(VISA resource name=w2030, byte count=w2029) -> (read buffer=w2025:string)  [unwired: 1 in, 3 out]
                            n1303 = Decimal String To Number(string=w2025) -> (number=w2024:i32)  [unwired: 2 in, 1 out]
                            n1304 = Decimal String To Number(string=w2023) -> (number=w2022:i32)  [unwired: 2 in, 1 out]
                            n1305 = Equal?(x=w2024, y=w2022) -> (x = y?=w2027:bool)
                          }
                          frame #1 {
                            n1306 = Equal?(x=w2034, y=1000) -> (x = y?=w2036:bool)
                            n1307 = case shown="False" w2036 {
                              tunnel: [_ w2037] -> w2033
                              frame False {
                              }
                              frame True {
                                n1308 = One Button Dialog(message="Temperature Timeout") -> (true=w2037:bool)  [unwired: 1 in]
                              }
                            }
                          }
                        }
                        n1309 = Or(x=w2019, y=w2020) -> (x .or. y?=w2018:bool)
                      }
                    }
                    frame #3 {
                      n1310 = local read "Desired Device"() -> (w2051:u16)
                      n1311 = flat-sequence {
                        tunnel: [w2088] -> w2065
                        tunnel: [w2087] -> w2064
                        tunnel: [w2084] -> w2063
                        tunnel: [w2083] -> w2062
                        tunnel: [w2082] -> w2061
                        tunnel: [w2081] -> w2060
                        tunnel: [w2066] -> w2059
                        tunnel: w2051 -> [w2066]
                        tunnel: w2065 -> [w2104]
                        tunnel: w2064 -> [w2103]
                        tunnel: w2063 -> [w2101]
                        tunnel: w2062 -> [w2100]
                        tunnel: w2061 -> [w2099]
                        tunnel: w2060 -> [w2098]
                        tunnel: [w2097] -> w2058
                        tunnel: [w2096] -> w2057
                        tunnel: [w2095] -> w2056
                        tunnel: w2059 -> [w2095]
                        tunnel: w2058 -> [w2114]
                        tunnel: w2057 -> [w2113]
                        tunnel: [w2112] -> w2055
                        tunnel: w2056 -> [w2112]
                        tunnel: [w2125] -> w2054
                        tunnel: w2055 -> [w2125]
                        tunnel: w2054 -> [w2150]
                        tunnel: [w2150] -> w2053
                        tunnel: w2053 -> [w2165]
                        tunnel: [w2165] -> w2042
                        tunnel: [w2158] -> w2040
                        tunnel: w2042 -> [w2176]
                        tunnel: [w2176] -> w2041
                        tunnel: w2040 -> [w2175]
                        tunnel: [w2175] -> w2039
                        tunnel: w2041 -> [_]
                        tunnel: [w2201] -> w2050
                        tunnel: [w2195] -> w2048
                        tunnel: [w2194] -> w2046
                        tunnel: w2039 -> [w2193]
                        tunnel: [w2189] -> w2044
                        tunnel: [w2187] -> w2043
                        tunnel: w2050 -> [w2218]
                        tunnel: [w2218] -> w2049
                        tunnel: w2048 -> [w2217]
                        tunnel: [w2217] -> w2047
                        tunnel: w2046 -> [w2216]
                        tunnel: [w2216] -> w2045
                        tunnel: w2044 -> [w2214]
                        tunnel: w2043 -> [w2215]
                        tunnel: w2049 -> [w2235]
                        tunnel: w2047 -> [w2229]
                        tunnel: w2045 -> [w2228]
                        frame #0 {
                          n1312 = local read "Prober GPIB"() -> (w2089:string)
                          n1313 = local read "current y"() -> (w2085:i32)
                          n1314 = local read "current x"() -> (w2086:i32)
                          n1315 = local read "Laser Current (mA)"() -> (w2077:dbl)
                          n1316 = local read "Laser Current (mA)"() -> (w2075:dbl)
                          n1317 = local read "Parameters Flash 2"() -> (w2080:T4)
                          n1318 = local read "Fine Cell Clusters"() -> (w2093:T5)
                          n1319 = local read "ActiveArea_um2"() -> (w2073:dbl)
                          n1320 = local read "Output Power (mW)"() -> (w2071:dbl)
                          n1321 = local read "Output Power (mW)"() -> (w2074:dbl)
                          n1322 = call "EG2001 Move Z Down.vi"("GPIB Address"=w2089) -> ("Error Out"=w2087:errorcluster, "GPIB Address Out"=w2088:string)  [unwired: 9 in]
                          n1323 = Divide(x=w2073, y=100000000.0) -> (x/y=w2068:dbl)
                          n1324 = Index Array(array=w2093, index=w2066) -> (element=w2078:T22)
                          n1325 = Unbundle By Name(w2078) -> ("Cell Name"=w2092:string, "X-coord"=w2082:dbl, "Y-coord"=w2081:dbl, "Area"=w2091:dbl, "Mesa Area"=w2090:dbl)
                          n1326 = call "get Area.vi"("Laser"=w2077, "Cell Data Cluster"=w2078) -> ("Area"=w2079:dbl)  [unwired: 9 in]
                          n1327 = Multiply(x=w2071, y=0.001) -> (x*y=w2069:dbl)
                          n1328 = Subtract(x=w2081, y=w2085) -> (x-y=w2083:dbl)
                          n1329 = Subtract(x=w2082, y=w2086) -> (x-y=w2084:dbl)
                          n1330 = local write "Device Name"(w2092) -> ()
                          n1331 = local write "ActiveArea_um2"(w2091) -> ()
                          n1332 = local write "MesaArea_um2"(w2090) -> ()
                          n1333 = Divide(x=w2069, y=w2068) -> (x/y=w2067:dbl)
                          n1334 = Bundle By Name(cluster=w2080, "Cell Area (cm²)"=w2079, "Input Current (mA)"=w2075, "Power Density (W/cm^2)"=w2067, "Incident Power"=w2074) -> (w2076:T4)
                          n1335 = local write "Parameters Flash"(w2076) -> ()
                        }
                        frame #1 {
                          n1336 = local write "current x"(w2099) -> ()
                          n1337 = local write "current y"(w2098) -> ()
                          n1338 = case shown="False" FALSE {
                            tunnel: w2104 -> [_ w2111]
                            tunnel: w2103 -> [_ w2110]
                            tunnel: enum32{"Steps", "Microns"}."Microns" ("Steps/Microns") -> [_ w2109]
                            tunnel: w2101 -> [_ w2108]
                            tunnel: w2100 -> [_ w2107]
                            tunnel: [_ w2106] -> w2097
                            tunnel: [_ w2105] -> w2096
                            frame False {
                            }
                            frame True {
                              n1339 = call "EG2001 Move Machine Step X-Y.vi"("Y"=w2107, "Steps/Microns"=w2109, "X"=w2108, "error in (no error)"=w2110, "GPIB Address"=w2111) -> ("Error Out"=w2105:errorcluster, "GPIB Address Out"=w2106:string)  [unwired: 5 in]
                            }
                          }
                        }
                        frame #2 {
                          n1340 = call "EG2001 Move Z Up.vi"("error in (no error)"=w2113, "GPIB Address"=w2114) -> ()  [unwired: 10 out]
                        }
                        frame #3 {
                          n1341 = call "DAQ Assistant2"() -> ("data"=w2117:dynamicdata)  [unwired: 17 in, 2 out]
                          n1342 = local read "Channel"() -> (w2134:enum32{"Channel A", "Channel B"})
                          n1343 = local read "Temp Setpoint"() -> (w2119:string)
                          n1344 = local read "Wafer Info Flash 2"() -> (w2124:T3)
                          n1345 = local read "I compliance sweep"() -> (w2129:dbl)
                          n1346 = local read "sweep delay ms"() -> (w2128:dbl)
                          n1347 = local read "Sweep Settings"() -> (w2136:T10)
                          n1348 = local read "Device Name"() -> (w2123:string)
                          n1349 = local read "Temp Data"() -> (w2120:T1)
                          n1350 = Decimal String To Number(string=w2119) -> (number=w2116:i32)  [unwired: 2 in, 1 out]
                          n1351 = Bundle By Name(cluster=w2124, "Cell Name"=w2123) -> (w2122:T3)
                          n1352 = Bundle By Name(cluster=w2120, "Ambient Temperature"=w2117, "Chuck Set Temperature"=w2116) -> (w2118:T1)
                          n1353 = local read "V start"() -> (w2132:dbl)
                          n1354 = local read "points"() -> (w2131:u16)
                          n1355 = local read "V end"() -> (w2133:dbl)
                          n1356 = local read "NPLC"() -> (w2130:dbl)
                          n1357 = local write "Wafer Info Flash"(w2122) -> ()
                          n1358 = Bundle By Name(cluster=w2136, "Channel"=w2134, "Vstart"=w2132, "Vend"=w2133, "# of points"=w2131, "NPLC"=w2130, "I compliance"=w2129, "Delay ms"=w2128) -> (w2135:T10)
                          n1359 = local read "Keysight"() -> (w2115:bool)
                          n1360 = local write "Temp Data"(w2118) -> ()
                          n1361 = local read "4-wire"() -> (w2121:bool)
                          n1362 = case shown="False" w2115 {
                            tunnel: w2135 -> [w2141 w2146]
                            tunnel: [w2139 w2144] -> w2127
                            tunnel: [w2138 w2143] -> w2126
                            tunnel: w2121 -> [w2137 w2145]
                            frame False {
                              n1363 = local read "Keithley SMU"() -> (w2140:refnum<visa-resource-name>)
                              n1364 = call "K2602 Vsweep.vi"("4-wire"=w2137, "Settings"=w2141, "SMU"=w2140) -> ("V"=w2138:dbl[], "I"=w2139:dbl[])  [unwired: 6 in, 1 out]
                            }
                            frame True {
                              n1365 = local read "Keysight SMU"() -> (w2142:refnum<visa-resource-name>)
                              n1366 = call "IVSweep (SubVI).vi"("SweepSettings"=w2146, "4 wire"=w2145, "VISA Refnum in"=w2142) -> ("V"=w2143:dbl[], "I"=w2144:dbl[])  [unwired: 1 in, 2 out]
                            }
                          }
                          n1367 = local write "V fine"(w2126) -> ()
                          n1368 = local write "I fine"(w2127) -> ()
                        }
                        frame #4 {
                          n1369 = local read "Device Name"() -> (w2148:string)
                          n1370 = local read "Wafer Info 3"() -> (w2149:T2)
                          n1371 = Bundle By Name(cluster=w2149, "Cell Name (Automatic)"=w2148) -> (w2147:T2)
                          n1372 = local write "Wafer Info 3"(w2147) -> ()
                        }
                        frame #5 {
                          n1373 = local read "Temperature Series save path"() -> (w2157:path)
                          n1374 = local read "Lot"() -> (w2156:string)
                          n1375 = local read "Wafer Name"() -> (w2154:string)
                          n1376 = local read "Device Name"() -> (w2164:string)
                          n1377 = local read "Output Power (mW)"() -> (w2163:dbl)
                          n1378 = Build Path(base path=w2157, name or relative path=w2156) -> (appended path=w2155:path)
                          n1379 = call "CreateDirectory.vi"("Path to be created"=w2155) -> ()  [unwired: 10 in, 1 out]
                          n1380 = Build Path(base path=w2155, name or relative path=w2154) -> (appended path=w2153:path)
                          n1381 = Number To Decimal String(number=w2163) -> (decimal integer string=w2161:string)  [unwired: 1 in]
                          n1382 = call "CreateDirectory.vi"("Path to be created"=w2153) -> ()  [unwired: 10 in, 1 out]
                          n1383 = Concatenate Strings(w2161, " mW" ("string")) -> (w2159:string)
                          n1384 = Build Path(base path=w2153, name or relative path="Temperature Series") -> (appended path=w2151:path)
                          n1385 = call "CreateDirectory.vi"("Path to be created"=w2151) -> ()  [unwired: 10 in, 1 out]
                          n1386 = Build Path(base path=w2151, name or relative path=w2164) -> (appended path=w2162:path)
                          n1387 = call "CreateDirectory.vi"("Path to be created"=w2162) -> ()  [unwired: 10 in, 1 out]
                          n1388 = Build Path(base path=w2162, name or relative path=w2159) -> (appended path=w2158:path)
                          n1389 = call "CreateDirectory.vi"("Path to be created"=w2158) -> ()  [unwired: 10 in, 1 out]
                        }
                        frame #6 {
                          n1390 = local read "I compliance sweep"() -> (w2170:dbl)
                          n1391 = local read "sweep delay ms"() -> (w2169:dbl)
                          n1392 = local read "Sweep Direction (Keysight)"() -> (w2174:i32)
                          n1393 = local read "points"() -> (w2171:u16)
                          n1394 = local read "V end"() -> (w2172:dbl)
                          n1395 = local read "V start"() -> (w2173:dbl)
                          n1396 = call "pho_DBCheck_LIV_meas_recipe.vi"("V start"=w2173, "Sweep Direction (Keysight)"=w2174, "V end"=w2172, "points"=w2171, "I compliance sweep"=w2170, "sweep delay ms"=w2169) -> ("RecipeID"=w2168:string)  [unwired: 8 in, 1 out]
                          n1397 = local write "RecipeID"(w2168) -> ()
                          n1398 = Equal?(x=w2168, y="") -> (x = y?=w2166:bool)
                          n1399 = case shown="True" w2166 {
                            frame False {
                            }
                            frame True {
                              n1400 = local read "I compliance sweep"() -> (w2179:dbl)
                              n1401 = local read "sweep delay ms"() -> (w2178:dbl)
                              n1402 = local read "Sweep Direction (Keysight)"() -> (w2183:i32)
                              n1403 = local read "points"() -> (w2180:u16)
                              n1404 = local read "V end"() -> (w2181:dbl)
                              n1405 = local read "V start"() -> (w2182:dbl)
                              n1406 = call "pho_DB_Insert_LIV_meas_recipe.vi"("V start"=w2182, "Sweep Direction (Keysight)"=w2183, "V end"=w2181, "points"=w2180, "I compliance sweep"=w2179, "sweep delay ms"=w2178) -> ("RecipeID"=w2177:string)  [unwired: 9 in]
                              n1407 = local write "RecipeID"(w2177) -> ()
                            }
                          }
                        }
                        frame #7 {
                          n1408 = local read "Temp Setpoint"() -> (w2186:string)
                          n1409 = local read "iteration"() -> (w2189:i32)
                          n1410 = local read "V fine"() -> (w2200:dbl[])
                          n1411 = local read "I fine"() -> (w2206:dbl[])
                          n1412 = local read "IV temp linear"() -> (w2212:cluster{dbl[], dbl[]}[])
                          n1413 = local read "Wafer Name"() -> (w2204:string)
                          n1414 = local read "Comments"() -> (w2191:string)
                          n1415 = local read "IV temp log"() -> (w2208:cluster{dbl[], dbl[]}[])
                          n1416 = local read "Operator"() -> (w2203:string)
                          n1417 = local read "current y"() -> (w2196:i32)
                          n1418 = local read "current x"() -> (w2197:i32)
                          n1419 = Bundle("V fine"=w2200, "I fine"=w2206) -> (w2210:cluster{"V fine":dbl[], "I fine":dbl[]})  [unwired: 1 in]
                          n1420 = Absolute Value(x=w2206) -> (abs(x)=w2207:dbl[])
                          n1421 = Decimal String To Number(string=w2186) -> (number=w2185:i32)  [unwired: 2 in, 1 out]
                          n1422 = local read "Device Name"() -> (w2202:string)
                          n1423 = Number To Decimal String(number=w2185) -> (decimal integer string=w2184:string)  [unwired: 1 in]
                          n1424 = Replace Array Subset(array=w2212, new element=w2210, index=w2189) -> (w2211:cluster{dbl[], dbl[]}[])
                          n1425 = To Double Precision Float(number=w2197) -> (double precision float=w2199:dbl)
                          n1426 = To Double Precision Float(number=w2196) -> (double precision float=w2198:dbl)
                          n1427 = Bundle("V fine"=w2200, w2207) -> (w2205:cluster{"V fine":dbl[], dbl[]})  [unwired: 1 in]
                          n1428 = Get Date/Time In Seconds() -> (seconds since 1Jan1904=w2194:timestamp)
                          n1429 = local read "Wafer Info 3"() -> (w2192:T2)
                          n1430 = local write "IV temp linear"(w2211) -> ()
                          n1431 = Bundle By Name(cluster=w2192, "Comment"=w2191) -> (w2190:T2)
                          n1432 = call "get Flash FileName .vi"("Time"=w2194, "Device Name"=w2202, "Operator"=w2203, "Wafer Name"=w2204, "FineTest save path"=w2193) -> ("appended path"=w2201:path)  [unwired: 6 in]
                          n1433 = Replace Array Subset(array=w2208, new element=w2205, index=w2189) -> (w2209:cluster{dbl[], dbl[]}[])
                          n1434 = Bundle(w2199, w2198) -> (w2195:cluster{dbl, dbl})  [unwired: 1 in]
                          n1435 = Concatenate Strings(w2184, " C" ("string")) -> (w2187:string)
                          n1436 = local write "IV temp log"(w2209) -> ()
                          n1437 = local write "Wafer Info 3"(w2190) -> ()
                        }
                        frame #8 {
                          n1438 = Increment(x=w2214) -> (x+1=w2213:i32)
                          n1439 = property on="IV temp linear" class="XYGraph (strict)"("Active Plot"=w2214, "Plot.Plot Name"=w2215, "LegNumRows"=w2213) -> ()  [unwired: 2 in, 2 out]
                          n1440 = property on="IV temp log" class="XYGraph (strict)"("Active Plot"=w2214, "Plot.Plot Name"=w2215, "LegNumRows"=w2213) -> ()  [unwired: 2 in, 2 out]
                        }
                        frame #9 {
                          n1441 = local read "V fine"() -> (w2232:dbl[])
                          n1442 = local read "I fine"() -> (w2233:dbl[])
                          n1443 = Get Date/Time String(seconds (now)=w2228, want seconds? (F)=TRUE) -> (date string=w2227:string, time string=w2225:string)  [unwired: 1 in]
                          n1444 = local read "Parameters Flash"() -> (w2230:T4)
                          n1445 = local read "RecipeID"() -> (w2220:string)
                          n1446 = Build Array(w2232, w2233) -> (w2231:dbl[][])
                          n1447 = call <vilib>:"Space Constant.vi"() -> ("String"=w2224:string)
                          n1448 = local read "Wafer Info 3"() -> (w2221:T2)
                          n1449 = Concatenate Strings(w2227, w2224, w2225) -> (w2223:string)
                          n1450 = local read "Temp Data"() -> (w2222:T1)
                          n1451 = local read "Mask"() -> (w2234:string)
                          n1452 = local read "Operator"() -> (w2219:string)
                          n1453 = call "WriteFlashFile NEW.vi"("Input File Path"=w2235, "IV array"=w2231, "Parameters"=w2230, "RecipeID"=w2220, "User"=w2219, "Coords"=w2229, "Wafer Info"=w2221, "Mask Name"=w2234, "Temp Data"=w2222, "Die Number"=w2223) -> ()  [unwired: 17 in, 1 out]
                        }
                      }
                      n1454 = local write "Status"("IV test running..." ("string")) -> ()
                    }
                  }
                  "iteration" <- w1997
                }
              }
              frame #2 {
                w2248 = -1 ("x")
                n1455 = local read "Temptronics VISA"() -> (w2237:refnum<visa-resource-name>)
                n1456 = local read "Prober GPIB"() -> (w2244:string)
                n1457 = local read "current y"() -> (w2247:i32)
                n1458 = local read "current x"() -> (w2246:i32)
                n1459 = Multiply(x=w2247, y=w2248) -> (x*y=w2250:i32)
                n1460 = Multiply(x=w2248, y=w2246) -> (x*y=w2249:i32)
                n1461 = call "EG2001 Move Z Down.vi"("GPIB Address"=w2244) -> ("Error Out"=w2245:errorcluster, "GPIB Address Out"=w2243:string)  [unwired: 9 in]
                n1462 = VISA Write(VISA resource name=w2237, write buffer="rs25" ("string")) -> (VISA resource name out=w2238:refnum<visa-resource-name>)  [unwired: 1 in, 2 out]
                n1463 = VISA Write(VISA resource name=w2238, write buffer="st") -> (VISA resource name out=w2240:refnum<visa-resource-name>, return count=w2241:u32)  [unwired: 1 in, 1 out]
                n1464 = call "EG2001 Move Machine Step X-Y.vi"("Flip X Coordinates?"=FALSE, "Y"=w2250, "Steps/Microns"=enum32{"Steps", "Microns"}."Microns", "X"=w2249, "error in (no error)"=w2245, "GPIB Address"=w2243) -> ()  [unwired: 4 in, 2 out]
                n1465 = VISA Read(VISA resource name=w2240, byte count=w2241) -> (read buffer=w2242:string)  [unwired: 1 in, 3 out]
                n1466 = local write "Current Temp"(w2242) -> ()
              }
              frame #3 {
                w2254 = 0 ("current x")
                n1467 = local write "current y"(w2254) -> ()
                n1468 = local write "current x"(w2254) -> ()
                n1469 = local write "Status"("idle" ("Status")) -> ()
              }
            }
          }
          frame "add temp auto" {
            n1470 = local read "Auto Temp Set"() -> (w2259:dbl)
            n1471 = property on="Auto Temperature List" class="LstBox (strict)"() -> ("Item Names"=w2257:string[])  [unwired: 2 in, 2 out]
            n1472 = Format Into String(format string="%08.4f", w2259) -> (resulting string=w2256:string)  [unwired: 2 in, 1 out]
            n1473 = Build Array (concatenate)(w2257, w2256) -> (w2255:string[])
            n1474 = property on="Auto Temperature List" class="LstBox (strict)"("Item Names"=w2255) -> ()  [unwired: 2 in, 2 out]
          }
          frame "remove temp auto" {
            n1475 = local read "Auto Temperature List"() -> (w2262:i32)
            n1476 = property on="Auto Temperature List" class="LstBox (strict)"() -> ("Item Names"=w2264:string[])  [unwired: 2 in, 2 out]
            n1477 = Delete From Array(array=w2264, index=w2262) -> (array with subset deleted=w2263:string[])  [unwired: 1 in, 1 out]
            n1478 = property on="Auto Temperature List" class="LstBox (strict)"("Item Names"=w2263) -> ()  [unwired: 2 in, 2 out]
          }
          frame "clear temp auto" {
            n1479 = property on="Auto Temperature List" class="LstBox (strict)"("Item Names"=string[] []) -> ()  [unwired: 2 in, 2 out]
          }
          frame "explore data" {
          }
        }
      }
      n1480 = Release Queue(queue=w43, force destroy? (F)=TRUE, error in (no error)=w34) -> (error out=→"error out":errorcluster)  [unwired: 2 out]
    }
  }
